vi "PDC.vi"() -> ()   [LabVIEW 2013]
uses:
  CTRLs/PMU_CMDs.ctl
panel:
  out "path":path
  out "T button?":bool
  out "PMU1 CFG Packet 2":string[](array[string])
  out "PMU Row Number":i32
  out "UDP STRNG 2":string
  out "Date/Time 4":string
  out "Phasor Row Number":i32
  in  "Tab Control 2":T1(tab)
  out "MagnitudePMU":waveform(sgl)(graph)
  out "FrequencyPMU":waveform(sgl)(graph)
  out "PMUROCOF":waveform(sgl)(graph)
  out "PMUAnalogs":waveform(sgl)(graph)
  out "seconds":dbl
  out "Array 2":u16[][](array[numeric]) format="%b"
  out "Array":string[][](array[string])
  out "Analogs":string[][](array[string])
  out "Freq Floating?":bool[](array[boolean])
  out "Analog Floating?":bool[](array[boolean])
  out "Polar?":bool[](array[boolean])
  out "Transposed":string[][](array[string])
  out "Real":string[][](array[string])
  out "Imaginary":string[][](array[string])
  out "transposed array 5":sgl[][](array[numeric])
  out "transposed array 4":sgl[][](array[numeric])
  out "Phasors Floatingpoint?":bool[](array[boolean])
  out "Format":u16[](array[numeric]) format="%b"
  out "Digitals":u16[](array[numeric])
  out "Analog":u16[](array[numeric])
  out "Phasor":u16[](array[numeric])
  out "DGTL Packet":string[](array[string])
  out "ANG Packet":string[](array[string])
  out "DFREQ Packet":string[](array[string])
  out "FREQ Packet":string[](array[string])
  out "PZRs Packet":string[](array[string])
  out "UNITs 2":T2
  out "Date/Time 3":string
  out "PMU DATA Packet 2":string[](array[string])
  out "DATA FRAME 2":string
  out "error out 2":errorcluster
  out "UDP STRNG":string
  out "UNITs":T2
  out "Date/Time 2":string
  in  "Start Com Button":bool
  in  "User Configuration":T3(tab)
  in  "IP Address":string="127.0.0.1"
  in  "remote port":u16=4712
  in  "Device ID":u16
  in  "Unicast Address":string="192.168.0.101"
  in  "Local Port":u16=58431
  in  "TTL":u16=16
  in  "Send to Port":u16=58432
  out "Alert Incorrect \nNetwork Info":bool
  in  "Data Display":T4(tab)
  in  "PMU Phasors":i32(listbox)
  in  "PMU Analogs":i32(listbox)
  in  "PMU Digitals":i32(listbox)
  in  "dFreq":sgl[](array[numeric])
  in  "Frequency":sgl[](array[numeric])
  in  "Tab Control":T5(tab)
  in  "Complex Phasors":csg[][](array[numeric])
  in  "Magnitude":sgl[][](array[numeric])
  in  "Angle":sgl[][](array[numeric])
  in  "Analog Values":sgl[][](array[numeric])
  out "Boolean array":bool[][](array[boolean])
  out "Magnitude":sgl[](array[numeric])
  out "Angle":sgl[](array[numeric])
  out "Complex Phasors":csg[](array[numeric])
  out "DFREQ Values":dbl[](array[numeric])
  out "FREQ Values":dbl[](array[numeric])
  out "Chosen Data 2":i32(listbox)
  out "DATA ONLINE":bool
  in  "Display Cluster Output":bool
  out "UDP String":string
  in  "Data Selector":T6(tab)
  out "No. of Digitals in this PMU":u8
  out "No. of Analogs in this PMU":u8
  out "No. of Phasors in this PMU":u8
  out "Freq/dFreq Format":string
  out "Analog Format":string
  out "Phasor Format":string
  out "Phasor Type":string
  out "DATA_RATE":u32
  in  "Names of PMUs":i32(listbox)
  out "Nominal_Frequency":string
  out "NUM_of_PMUs":u32
  in  "PMU Phasors List 2":i32(listbox)
  out "Phasor_Names":string[](array[string])
  in  "PMU Phasors List":i32(listbox)
  out "Phasors Index":u16[](array[numeric])
  out "PMU number in List":i32[](array[numeric])
  out "Phasor number in selected PMU":i32[](array[numeric])
  out "PMU DATA Packet":string[](array[string])
  out "Data size to read":u32
  out "Size of DATA Frame":u32
  out "CFG-2 Frame":string
  out "PMU1 CFG Packet":string[](array[string])
  out "Date/Time":string
  out "TIME_BASE":u32
  out "FRACSEC":u64
  out "SOC":u64
  out "IDCODE":u32
  out "FRAMSIZE":u32
  out "SYNC":u32
  out "Valid?!":bool
  out "CRC-Bytes":string
  out "DATA FRAME":string
  in  "Stop Button":bool
  out "COMMAND Frame":string
  out "bytes written":i32
  in  "DATA ON":bool
  in  "DATA OFF":bool
  out "length":i32
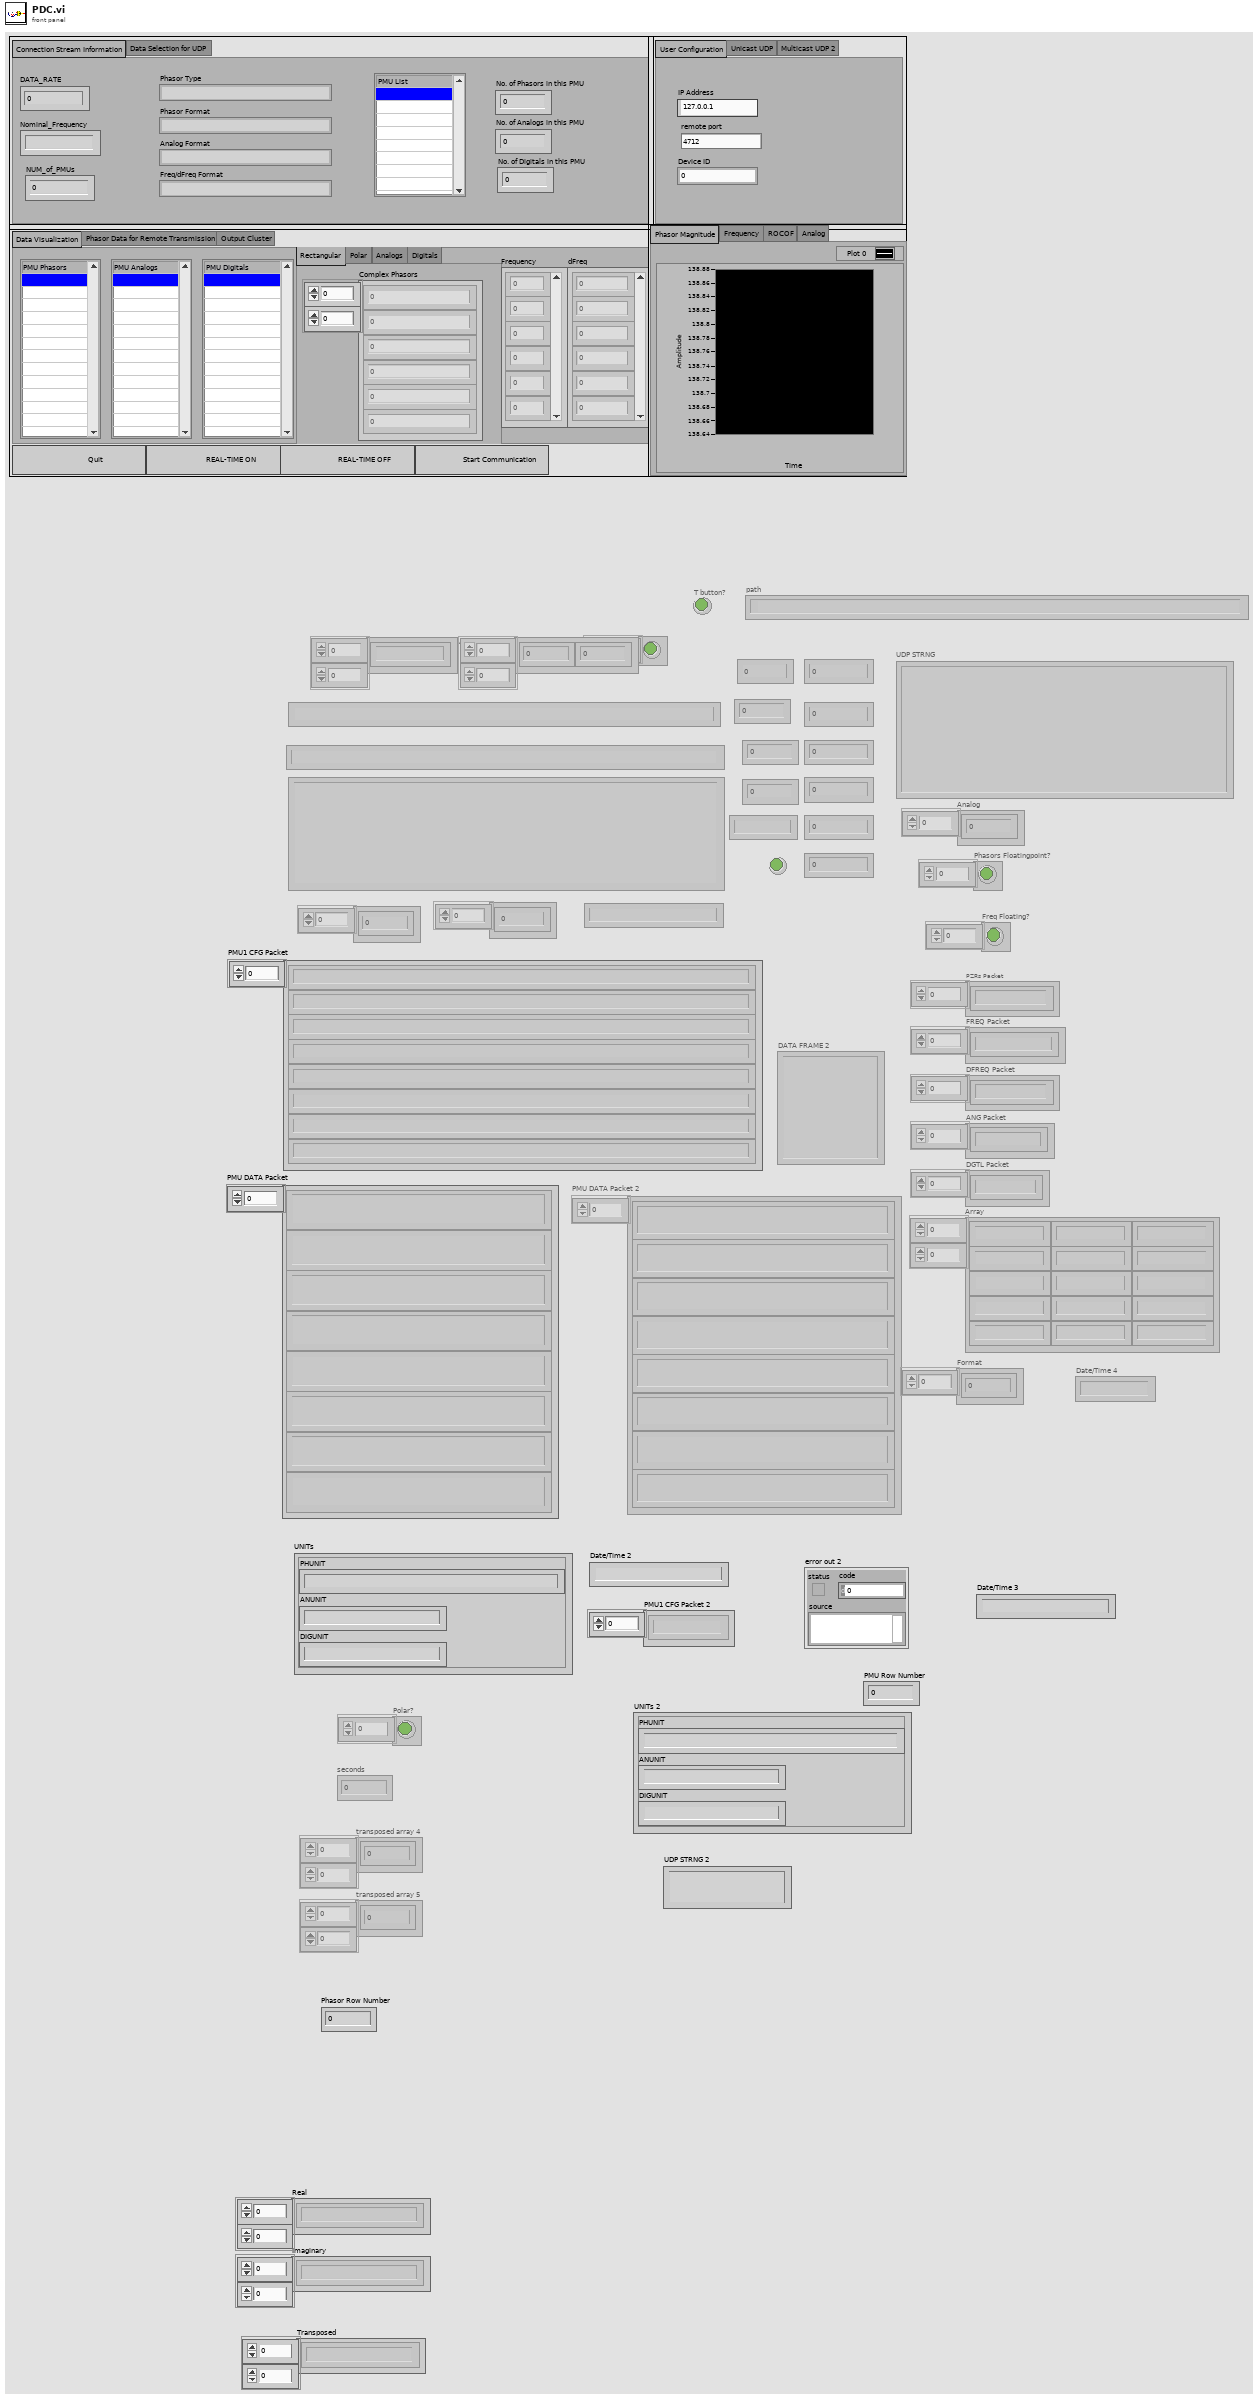
[diagram p1: front panel]
types:
  T1 = enum32{"Phasor Magnitude", "Frequency", "ROCOF", "Analog"}
  T2 = cluster{"PHUNIT":string, "ANUNIT":string, "DIGUNIT":string}
  T3 = enum32{"User Configuration", "Unicast UDP", "Multicast UDP 2"}
  T4 = enum32{"Data Visualization", "Phasor Data for Remote Transmission", "Output Cluster"}
  T5 = enum32{"Rectangular", "Polar", "Analogs", "Digitals"}
  T6 = enum32{"Connection Stream Information", "Data Selection for UDP"}
  T7 = cluster{"Date/Time":string, "DATA_DTLD":cluster{"PZRs Packet":string[], "FREQ Packet":string[], "DFREQ Packet":string[], "ANG Packet":string[], "DGTL Packet":string[]}}
  T8 = typedef "PMU_CMDs.ctl" = enum16{"dummy", "Turn off Transmission of Data Frame", "Turn on Transmission of Data Frame", "Send Header Frame", "Send CFG-1 Frame", "Send CFG-2 Frame", "Extended Frame"}
  T9 = cluster{"SYNC":u32, "FRAMSIZE":u32, "IDCODE":u32, "SOC":u64, "DATA_RATE":u32, "FRACSEC":u64, "TIME_BASE":u32, "NUM_PMU":u32}
  T10 = cluster{"PHASORS":cluster{"PZR 1":string, "PZR 2":string, "PZR 3":string, "PZR 4":string, "PZR 5":string, "PZR 6":string}, "NUMs":cluster{"PHNMR":u8, "ANNMR":u8, "DGNMR":u8}, "FORMAT":cluster{"PH_MAG_ANG":u16, "PH_FLOATING":u16, "AN_FLOATING":u16, "FREQ_DFREQ_FLOATING":u16}, "ANGs":cluster{"AN1":string, "AN2":string, "AN3":string}, "DIGs":cluster{"DIG 1":string, "DIG 2":string, "DIG 3":string, "DIG 4":string, "DIG 5":string, "DIG 6":string, "DIG 7":string, "DIG 8":string, "DIG 9":string, "DIG 10":string, "DIG 11":string, "DIG 12":string, "DIG 13":string, "DIG 14":string, "DIG 15":string, "DIG 16":string}, "IDCODE":u16, "Station Name":string, "UNITs":cluster{"PHUNIT":string, "ANUNIT":string, "DIGUNIT":string}, "FNOM":string, "CFGCNT":string}
  T11 = cluster{"PZRs Packet":string[], "FREQ Packet":string[], "DFREQ Packet":string[], "ANG Packet":string[], "DGTL Packet":string[]}
  T12 = typedef "LVDateTimeRec.ctl" = cluster{"fractional second":dbl, "second":i32, "minute":i32, "hour":i32, "day of month":i32, "month":i32, "year":i32, "day of week":i32, "day of year":i32, "DST":i32}
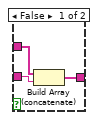
[diagram p4: hidden frame]
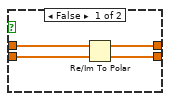
[diagram p5: hidden frame]
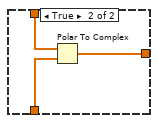
[diagram p6: hidden frame]
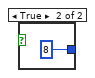
[diagram p7: hidden frame]
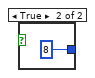
[diagram p8: hidden frame]
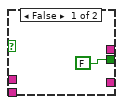
[diagram p11: hidden frame]
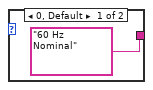
[diagram p14: hidden frame]
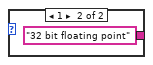
[diagram p15: hidden frame]
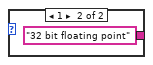
[diagram p16: hidden frame]
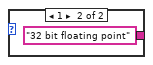
[diagram p17: hidden frame]
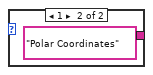
[diagram p18: hidden frame]
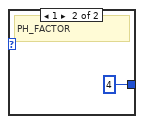
[diagram p19: hidden frame]
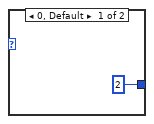
[diagram p20: hidden frame]
diagram:
  # "This file is part of BFE.\n\n    BFE is free software: you can redistribute it and/or modify\n    it under the terms of the GNU General Public License as published by\n    the Free Software Foundation, either version 3 of the License, or\n    (at your option) any later version.\n\n   BFE is distributed in the hope that it will be useful,\n    but WITHOUT ANY WARRANTY; without even the implied warranty of\n    MERCHANTABILITY or FITNESS FOR A PARTICULAR PURPOSE.  See the\n    GNU General Public License for more details.\n\n    You should have received a copy of the GNU General Public License\n    along with BFE.  If not, see <http://www.gnu.org/licenses/>."
  n1 = flat-sequence {
    tunnel: [w84] -> w64
    tunnel: [w83] -> w62
    frame #0 {
      w74 = "" ("Phasor Type")
      w73 = u8 0 ("No. of Phasors in this PMU")
      w72 = string[] [""] ("Phasor Name")
      # "License Prompt"
      # "Initializing all variables to their default values"
      n2 = Two Button Dialog(message="<BFE>  Copyright (C) <2016>  <Luigi Vanfretti, Muhammad Shoaib Almas, Maxime Baudette>\n    This program comes with ABSOLUTELY NO WARRANTY; for details click on \"show details\"'.\n    This is free software, and you are welcome to redistribute it\n    under certain conditions; click on `show details' for details.", 1:"Show Details" ("F button name (\"Cancel\")"), 2:"OK" ("T button name (\"OK\")")) -> (T button?=w67:bool)
      "T button?" <- w67
      n3 = Equal?(x=w67, y=FALSE) -> (x = y?=w65:bool)
      n4 = case shown="True" w65 {
        frame False {
        }
        frame True {
          n5 = Current VI's Path() -> (path=w79:path)
          "path" <- w79
          n6 = Strip Path(path=w79) -> (stripped path=w77:path)  [unwired: 1 out]
          n7 = Build Path(base path=w77, name or relative path="License") -> (appended path=w75:path)
          n8 = call <vilib>:"System Exec.vi"("working directory"=w75, "command line"="Notepad COPYING") -> ()  [unwired: 6 in, 4 out]
        }
      }
      n9 = property on="NUM_of_PMUs" class="DigNum (strict)"("Value"=w73) -> ()  [unwired: 2 in, 2 out]
      n10 = property on="DATA_RATE" class="DigNum (strict)"("Value"=w73) -> ()  [unwired: 2 in, 2 out]
      n11 = property on="No. of Phasors in this PMU" class="DigNum (strict)"("Value"=w73) -> ()  [unwired: 2 in, 2 out]
      n12 = property on="No. of Analogs in this PMU" class="DigNum (strict)"("Value"=w73) -> ()  [unwired: 2 in, 2 out]
      n13 = property on="No. of Digitals in this PMU" class="DigNum (strict)"("Value"=w73) -> ()  [unwired: 2 in, 2 out]
      n14 = property on="Analog Format" class="Str"("Value"=w74) -> ()  [unwired: 2 in, 2 out]
      n15 = property on="Phasor Type" class="Str"("Value"=w74) -> ()  [unwired: 2 in, 2 out]
      n16 = property on="Phasor Format" class="Str"("Value"=w74) -> ()  [unwired: 2 in, 2 out]
      n17 = property on="Freq/dFreq Format" class="Str"("Value"=w74) -> ()  [unwired: 2 in, 2 out]
      n18 = property on="Phasors Index" class="Arr (strict)"("Value"=u16[] [0, 0, 0, 0] ("Phasors Index")) -> ()  [unwired: 2 in, 2 out]
      n19 = property on="Nominal_Frequency" class="Str"("Value"=w74) -> ()  [unwired: 2 in, 2 out]
      n20 = property on="PMU Phasors List" class="LstBox (strict)"("Item Names"=w72) -> ()  [unwired: 2 in, 2 out]
      n21 = property on="PMU Analogs" class="LstBox (strict)"("Item Names"=w72) -> ()  [unwired: 2 in, 2 out]
      n22 = property on="PMU Phasors" class="LstBox (strict)"("Item Names"=w72) -> ()  [unwired: 2 in, 2 out]
      n23 = property on="PMU Digitals" class="LstBox (strict)"("Item Names"=w72) -> ()  [unwired: 2 in, 2 out]
      n24 = property on="Names of PMUs" class="LstBox (strict)"("Item Names"=w72) -> ()  [unwired: 2 in, 2 out]
      n25 = property on="Names of PMUs" class="LstBox (strict)"("Item Names"=w72) -> ()  [unwired: 2 in, 2 out]
      n26 = property on="Phasor_Names" class="Arr (strict)"("Value"=w72) -> ()  [unwired: 2 in, 2 out]
    }
    frame #1 {
      n27 = while {
        stop <- "Start Com Button" stop-if-true
      }
    }
    frame #2 {
      n28 = TCP Open Connection(address="IP Address", remote port or service name="remote port") -> (connection ID=w84:refnum<k5>, error out=w83:errorcluster)  [unwired: 3 in]
    }
  }
  n29 = flat-sequence {
    tunnel: w64 -> [w90]
    tunnel: w62 -> [w91]
    tunnel: [w89] -> w50
    tunnel: [w88] -> w49
    tunnel: ["Device ID"] -> w24
    tunnel: w50 -> [w95]
    tunnel: [w98] -> w48
    tunnel: w49 -> [w96]
    tunnel: [w97] -> w46
    tunnel: w24 -> [w92]
    tunnel: [w92] -> w23
    tunnel: w48 -> [w107]
    tunnel: [w108] -> w47
    tunnel: w46 -> [w106]
    tunnel: [w109] -> w45
    tunnel: [w100] -> w44
    tunnel: w23 -> [w99]
    tunnel: [w99] -> w22
    tunnel: w47 -> [w114]
    tunnel: [w114] -> w52
    tunnel: w45 -> [w113]
    tunnel: [w113] -> w51
    tunnel: w44 -> [w111]
    tunnel: [w111] -> w43
    tunnel: w22 -> [w110]
    tunnel: [w110] -> w21
    tunnel: w52 -> [w120]
    tunnel: [w119] -> w41
    tunnel: w51 -> [w118]
    tunnel: [w117] -> w40
    tunnel: w43 -> [w122]
    tunnel: [w122] -> w39
    tunnel: w21 -> [w115]
    tunnel: [w115] -> w20
    tunnel: w41 -> [w127]
    tunnel: w40 -> [w126]
    tunnel: [w129] -> w60
    tunnel: [w128] -> w59
    tunnel: w39 -> [w124]
    tunnel: [w124] -> w42
    tunnel: w20 -> [w123]
    tunnel: w60 -> [w141]
    tunnel: w59 -> [w140]
    tunnel: [w143] -> w58
    tunnel: [w142] -> w57
    tunnel: [w131] -> w56
    tunnel: w42 -> [w139]
    tunnel: w58 -> [w158]
    tunnel: w57 -> [w157]
    tunnel: w56 -> [w149]
    tunnel: [w158] -> w55
    tunnel: [w157] -> w54
    tunnel: [w149] -> w53
    tunnel: [w144] -> w38
    tunnel: w55 -> [w197]
    tunnel: w54 -> [w196]
    tunnel: w53 -> [w195]
    tunnel: w38 -> [w176]
    tunnel: [w197] -> w33
    tunnel: [w196] -> w32
    tunnel: [w172] -> w31
    tunnel: w33 -> [w218]
    tunnel: w32 -> [w217]
    tunnel: w31 -> [w216]
    tunnel: [w218] -> w28
    tunnel: [w217] -> w27
    tunnel: [w216] -> w26
    tunnel: [w230] -> w30
    tunnel: [w227] -> w61
    tunnel: [w225] -> w63
    tunnel: w28 -> [w226]
    tunnel: w27 -> [w228]
    tunnel: w26 -> [w230]
    frame #0 {
      n30 = call "CMD.vi"("PMU ID"="Device ID", "command"=PMU_CMDs."Turn off Transmission of Data Frame") -> ("CMD"=w87:string)  [unwired: 4 in, 1 out]
      n31 = TCP Write(connection ID=w90, data in=w87, error in (no error)=w91) -> (connection ID out=w89:refnum<k5>, error out=w88:errorcluster)  [unwired: 1 in, 1 out]
    }
    frame #1 {
      n32 = call "CMD.vi"("PMU ID"=w92, "command"=PMU_CMDs."Send CFG-2 Frame") -> ("CMD"=w93:string)  [unwired: 4 in, 1 out]
      n33 = TCP Write(connection ID=w95, data in=w93, error in (no error)=w96) -> (connection ID out=w98:refnum<k5>, error out=w97:errorcluster)  [unwired: 1 in, 1 out]
    }
    frame #2 {
      w103 = 2 ("offset (0)")
      n34 = TCP Read(connection ID=w107, bytes to read=4, error in (no error)=w106) -> (connection ID out=w108:refnum<k5>, data out=w104:string, error out=w109:errorcluster)  [unwired: 2 in]
      n35 = String Subset(string=w104, offset (0)=w103, length (rest)=w103) -> (substring=w102:string)
      n36 = Type Cast(type=u16 0 ("bytes to read"), x=w102) -> (*(type *) &x=w100:u16)
    }
    frame #3 {
      n37 = Wait (ms)(milliseconds to wait=u32 20) -> ()  [unwired: 1 out]
    }
    frame #4 {
      n38 = call "CMD.vi"("PMU ID"=w115, "command"=PMU_CMDs."Turn off Transmission of Data Frame") -> ("CMD"=w121:string)  [unwired: 4 in, 1 out]
      n39 = TCP Write(connection ID=w120, data in=w121, error in (no error)=w118) -> (connection ID out=w119:refnum<k5>, error out=w117:errorcluster)  [unwired: 1 in, 1 out]
    }
    frame #5 {
      n40 = call "CMD.vi"("PMU ID"=w123, "command"=PMU_CMDs."Send CFG-2 Frame") -> ("CMD"=w125:string)  [unwired: 4 in, 1 out]
      n41 = TCP Write(connection ID=w127, data in=w125, error in (no error)=w126) -> (connection ID out=w129:refnum<k5>, error out=w128:errorcluster)  [unwired: 1 in, 1 out]
    }
    frame #6 {
      w137 = 4 ("y")
      n42 = TCP Read(connection ID=w141, bytes to read=w139, error in (no error)=w140) -> (connection ID out=w143:refnum<k5>, data out=w132:string, error out=w142:errorcluster)  [unwired: 2 in]
      n43 = String Length(string=w132) -> (length=w138:i32)
      n44 = Subtract(x=w138, y=w137) -> (x-y=w133:i32)
      n45 = String Subset(string=w132, offset (0)=w133, length (rest)=w137) -> (substring=w136:string)
      n46 = String Subset(string=w132, offset (0)=0, length (rest)=w133) -> (substring=w135:string)
      n47 = Concatenate Strings(w136, w135) -> (w131:string)
      "CFG-2 Frame" <- w131
    }
    frame #7 {
      n48 = call "CHK_CRC.vi"("data in"=w149) -> ("Valid?!"=→"Valid?!":bool, "CRC-Bytes"=→"CRC-Bytes":string)
      n49 = call "SYS_INFO.vi"("CFG-2"=w149) -> ("output cluster"=w150:T9)
      n50 = Unbundle By Name(w150) -> ("SYNC"=→"SYNC":u32, "FRAMSIZE"=→"FRAMSIZE":u32, "IDCODE"=→"IDCODE":u32, "SOC"=w148:u64, "FRACSEC"=w146:u64, "TIME_BASE"=w145:u32, "NUM_PMU"=w144:u32, "DATA_RATE"=→"DATA_RATE":u32)
      "SOC" <- w148
      "FRACSEC" <- w146
      "TIME_BASE" <- w145
      "NUM_of_PMUs" <- w144
      n51 = call "UNIX-DATE_TIME.vi"("TIME_BASE"=w145, "FRACSEC"=w146, "SOC"=w148) -> ("Date/Time"=→"Date/Time":string)  [unwired: 1 out]
    }
    frame #8 {
      w192 = 4
      w174 = 2
      n52 = call "PMU_CFG-2_PACK.vi"("String"=w195) -> ("PMU1 CFG Packet"=w172:string[])
      "PMU1 CFG Packet" <- w172
      n53 = Index Array(array=w172, index=0) -> (element=w194:string)
      n54 = call "PMU_INFO.vi"("data in"=w194) -> ("RET_DATA"=w162:T10)
      n55 = Unbundle By Name(w162) -> ("FNOM"=w161:string)
      n56 = Type Cast(type=u16 2 ("length (rest)"), x=w161) -> (*(type *) &x=w160:u16)
      n57 = Unbundle By Name(w162) -> ("FORMAT.PH_MAG_ANG"=w168:u16, "FORMAT.PH_FLOATING"=w167:u16, "FORMAT.AN_FLOATING"=w166:u16, "FORMAT.FREQ_DFREQ_FLOATING"=w165:u16)
      n58 = case shown="1" w160 {
        tunnel: ["60 Hz Nominal" "50 Hz"] -> w159
        frame 0, Default {
        }
        frame 1 {
        }
      }
      "Nominal_Frequency" <- w159
      n59 = case shown="0, Default" w168 {
        tunnel: ["Rectangular Coordinates" "Polar Coordinates"] -> w164
        frame 0, Default {
        }
        frame 1 {
        }
      }
      "Phasor Type" <- w164
      n60 = case shown="0, Default" w167 {
        tunnel: ["16 bit integer" "32 bit floating point"] -> w171
        frame 0, Default {
        }
        frame 1 {
        }
      }
      "Phasor Format" <- w171
      n61 = case shown="0, Default" w166 {
        tunnel: ["16 bit integer" "32 bit floating point"] -> w170
        frame 0, Default {
        }
        frame 1 {
        }
      }
      "Analog Format" <- w170
      n62 = case shown="0, Default" w165 {
        tunnel: ["16 bit integer" "32 bit floating point"] -> w169
        frame 0, Default {
        }
        frame 1 {
        }
      }
      "Freq/dFreq Format" <- w169
      n63 = Unbundle By Name(w162) -> ("FORMAT.PH_FLOATING"=w185:u16, "FORMAT.AN_FLOATING"=w184:u16, "FORMAT.FREQ_DFREQ_FLOATING"=w186:u16, "NUMs.PHNMR"=w190:u8, "NUMs.ANNMR"=w182:u8, "NUMs.DGNMR"=w179:u8)  [unwired: 1 out]
      n64 = case shown="0, Default" w185 {
        tunnel: [4 8] -> w191
        frame 0, Default {
        }
        frame 1 {
          # "PH_FACTOR"
        }
      }
      n65 = case shown="0, Default" w184 {
        tunnel: [2 4] -> w183
        frame 0, Default {
        }
        frame 1 {
          # "PH_FACTOR"
        }
      }
      n66 = Multiply(x=w179, y=2) -> (x*y=w180:i32)
      n67 = case shown="1" w186 {
        tunnel: [2 4] -> w187
        frame 0, Default {
        }
        frame 1 {
          # "PH_FACTOR"
        }
      }
      n68 = Multiply(x=w191, y=w190) -> (x*y=w188:i32)
      n69 = Multiply(x=w182, y=w183) -> (x*y=w181:i32)
      n70 = Compound Arithmetic op=ADD(2, w188, w187, w187, w181, w180) -> (w177:i32)
      n71 = Multiply(x=w177, y=w176) -> (x*y=w175:u32)
      n72 = Compound Arithmetic op=ADD(w174, w174, w174, w192, w192, w175, w174) -> (→"Size of DATA Frame":u32)
    }
    frame #9 {
      n73 = property on="NUM_of_PMUs" class="DigNum (strict)"() -> ("Value"=w215:u32)  [unwired: 2 in, 2 out]
      n74 = for {
        N: w215 -> [_]
        tunnel: w216 -> [w222] mode=indexing
        tunnel: [w219] -> w214 mode=indexing
        n75 = String Subset(string=w222, offset (0)=0, length (rest)=16 ("length (rest)")) -> (substring=w219:string)
      }
      n76 = property on="PMU Phasors List 2" class="LstBox (strict)"("Item Names"=w214) -> ()  [unwired: 2 in, 2 out]
      n77 = property on="Names of PMUs" class="LstBox (strict)"("Item Names"=w214) -> ()  [unwired: 2 in, 2 out]
    }
    frame #10 {
      n78 = local read "Device ID"() -> (w223:u16)
      n79 = call "CMD.vi"("PMU ID"=w223, "command"=PMU_CMDs."Turn off Transmission of Data Frame") -> ("CMD"=w229:string)  [unwired: 4 in, 1 out]
      n80 = TCP Write(connection ID=w226, data in=w229, error in (no error)=w228) -> (connection ID out=w225:refnum<k5>, error out=w227:errorcluster)  [unwired: 1 in, 1 out]
    }
  }
  n81 = flat-sequence {
    tunnel: ["Send to Port"] -> w10
    tunnel: [w249] -> w7
    tunnel: [w248] -> w9
    tunnel: [w236] -> w8
    frame #0 {
      # "Local Port number on this\nmachine"
      # "Time To Live edit\nbox usually 16 is the\nbest to send over networks"
      # "IP Address of destination\nsite over UDP."
      # "send the phasor\nparameters to this\nUDP port edit box"
      # "Open a UDP port for Multicast Write Only."
      n82 = String To IP(1:"0.0.0.0" ("x")) -> (0:w245:u32)
      n83 = String To IP(1:"223.255.255.255" ("x")) -> (0:w244:u32)
      n84 = String To IP(1:"Unicast Address") -> (0:w236:u32)
      n85 = String To IP(1:"240.255.255.255" ("x")) -> (0:w240:u32)
      n86 = String To IP(1:"247.255.255.255" ("x")) -> (0:w239:u32)
      n87 = Greater Or Equal?(x=w236, y=w245) -> (x >= y?=w247:bool)
      n88 = Less Or Equal?(x=w236, y=w244) -> (x <= y?=w246:bool)
      n89 = Greater Or Equal?(x=w236, y=w240) -> (x >= y?=w235:bool)
      n90 = Less Or Equal?(x=w236, y=w239) -> (x <= y?=w234:bool)
      n91 = Not And(1:w246, 2:w247) -> (0:w233:bool)
      n92 = Not And(1:w234, 2:w235) -> (0:w232:bool)
      n93 = And(x=w233, y=w232) -> (x .and. y?=w231:bool)
      "Alert Incorrect \nNetwork Info" <- w231
      n94 = case shown="True" w231 {
        frame False {
        }
        frame True {
          n95 = call "Display Message to User"() -> ()  [unwired: 10 in, 2 out]
        }
      }
      n96 = UDP Open(9:"TTL", 11:"Local Port") -> (port=w249:refnum<k16>, 0:w248:errorcluster)  [unwired: 3 in, 1 out]
      "error out 2" <- w248
    }
  }
  n97 = Obtain Queue(name (unnamed)="DISP DATA", element data type=T7 {"Date/Time"="26-12-2013, 0:30:36 0.866666", "DATA_DTLD"={"PZRs Packet"=[], "FREQ Packet"=[], "DFREQ Packet"=[], "ANG Packet"=[], "DGTL Packet"=[]}}) -> (queue out=w4:refnum<queue>, error out=w3:errorcluster)  [unwired: 3 in, 1 out]
  n98 = Obtain Queue(name (unnamed)="DATA FRAME", element data type=cluster{"DATA Type":string, "CFG Type":string[]} {"DATA Type"="", "CFG Type"=["PMU.001\u0000\u0000\u0000\u0000\u0000\u0000\u0000\u0000\u0000\u0000\u0001\u0000\u000f\u0000\u0006\u0000\u0003\u0000\u0001PZR.AI          PZR.BV          PZR.CI          PZR.AV          PZR.BI          PZR.CV          ANA1            ANA2            ANA3            DIG.stat1_01    DIG.stat1_02    DIG.stat1_03    DIG.stat1_04    DIG.stat1_05    DIG.stat1_06    DIG.stat1_07    DIG.stat1_08    DIG.stat1_09    DIG.stat1_10    DIG.stat1_11    DIG.stat1_12    DIG.stat1_13    DIG.stat1_14    DIG.stat1_15    DIG.stat1_16    \u0001\u0000\u0000\u0000\u0000\u0000\u0000\u0000\u0001\u0000\u0000\u0000\u0000\u0000\u0000\u0000\u0001\u0000\u0000\u0000\u0000\u0000\u0000\u0000\u0000\u0000\u0000\u0000\u0000\u0000\u0000\u0000\u0000\u0000\u0000\u0000ÿÿ\u0000\u0000\u0000\u0000\u0000\u0000", "PMU.002\u0000\u0000\u0000\u0000\u0000\u0000\u0000\u0000\u0000\u0000\u0002\u0000\u000f\u0000\u0006\u0000\u0003\u0000\u0001PZR.AI          PZR.BV          PZR.CI          PZR.AV          PZR.BI          PZR.CV          ANA1            ANA2            ANA3            DIG.stat1_01    DIG.stat1_02    DIG.stat1_03    DIG.stat1_04    DIG.stat1_05    DIG.stat1_06    DIG.stat1_07    DIG.stat1_08    DIG.stat1_09    DIG.stat1_10    DIG.stat1_11    DIG.stat1_12    DIG.stat1_13    DIG.stat1_14    DIG.stat1_15    DIG.stat1_16    \u0001\u0000\u0000\u0000\u0000\u0000\u0000\u0000\u0001\u0000\u0000\u0000\u0000\u0000\u0000\u0000\u0001\u0000\u0000\u0000\u0000\u0000\u0000\u0000\u0000\u0000\u0000\u0000\u0000\u0000\u0000\u0000\u0000\u0000\u0000\u0000ÿÿ\u0000\u0000\u0000\u0000\u0000\u0000", "PMU.003\u0000\u0000\u0000\u0000\u0000\u0000\u0000\u0000\u0000\u0000\u0003\u0000\u000f\u0000\u0006\u0000\u0003\u0000\u0001PZR.AI          PZR.BV          PZR.CI          PZR.AV          PZR.BI          PZR.CV          ANA1            ANA2            ANA3            DIG.stat1_01    DIG.stat1_02    DIG.stat1_03    DIG.stat1_04    DIG.stat1_05    DIG.stat1_06    DIG.stat1_07    DIG.stat1_08    DIG.stat1_09    DIG.stat1_10    DIG.stat1_11    DIG.stat1_12    DIG.stat1_13    DIG.stat1_14    DIG.stat1_15    DIG.stat1_16    \u0001\u0000\u0000\u0000\u0000\u0000\u0000\u0000\u0001\u0000\u0000\u0000\u0000\u0000\u0000\u0000\u0001\u0000\u0000\u0000\u0000\u0000\u0000\u0000\u0000\u0000\u0000\u0000\u0000\u0000\u0000\u0000\u0000\u0000\u0000\u0000ÿÿ\u0000\u0000\u0000\u0000\u0000\u0000", "PMU.004\u0000\u0000\u0000\u0000\u0000\u0000\u0000\u0000\u0000\u0000\u0004\u0000\u000f\u0000\u0006\u0000\u0003\u0000\u0001PZR.AI          PZR.BV          PZR.CI          PZR.AV          PZR.BI          PZR.CV          ANA1            ANA2            ANA3            DIG.stat1_01    DIG.stat1_02    DIG.stat1_03    DIG.stat1_04    DIG.stat1_05    DIG.stat1_06    DIG.stat1_07    DIG.stat1_08    DIG.stat1_09    DIG.stat1_10    DIG.stat1_11    DIG.stat1_12    DIG.stat1_13    DIG.stat1_14    DIG.stat1_15    DIG.stat1_16    \u0001\u0000\u0000\u0000\u0000\u0000\u0000\u0000\u0001\u0000\u0000\u0000\u0000\u0000\u0000\u0000\u0001\u0000\u0000\u0000\u0000\u0000\u0000\u0000\u0000\u0000\u0000\u0000\u0000\u0000\u0000\u0000\u0000\u0000\u0000\u0000ÿÿ\u0000\u0000\u0000\u0000\u0000\u0000", "PMU.005\u0000\u0000\u0000\u0000\u0000\u0000\u0000\u0000\u0000\u0000\u0005\u0000\u000f\u0000\u0006\u0000\u0003\u0000\u0001PZR.AI          PZR.BV          PZR.CI          PZR.AV          PZR.BI          PZR.CV          ANA1            ANA2            ANA3            DIG.stat1_01    DIG.stat1_02    DIG.stat1_03    DIG.stat1_04    DIG.stat1_05    DIG.stat1_06    DIG.stat1_07    DIG.stat1_08    DIG.stat1_09    DIG.stat1_10    DIG.stat1_11    DIG.stat1_12    DIG.stat1_13    DIG.stat1_14    DIG.stat1_15    DIG.stat1_16    \u0001\u0000\u0000\u0000\u0000\u0000\u0000\u0000\u0001\u0000\u0000\u0000\u0000\u0000\u0000\u0000\u0001\u0000\u0000\u0000\u0000\u0000\u0000\u0000\u0000\u0000\u0000\u0000\u0000\u0000\u0000\u0000\u0000\u0000\u0000\u0000ÿÿ\u0000\u0000\u0000\u0000\u0000\u0000", "PMU.006\u0000\u0000\u0000\u0000\u0000\u0000\u0000\u0000\u0000\u0000\u0006\u0000\u000f\u0000\u0006\u0000\u0003\u0000\u0001PZR.AI          PZR.BV          PZR.CI          PZR.AV          PZR.BI          PZR.CV          ANA1            ANA2            ANA3            DIG.stat1_01    DIG.stat1_02    DIG.stat1_03    DIG.stat1_04    DIG.stat1_05    DIG.stat1_06    DIG.stat1_07    DIG.stat1_08    DIG.stat1_09    DIG.stat1_10    DIG.stat1_11    DIG.stat1_12    DIG.stat1_13    DIG.stat1_14    DIG.stat1_15    DIG.stat1_16    \u0001\u0000\u0000\u0000\u0000\u0000\u0000\u0000\u0001\u0000\u0000\u0000\u0000\u0000\u0000\u0000\u0001\u0000\u0000\u0000\u0000\u0000\u0000\u0000\u0000\u0000\u0000\u0000\u0000\u0000\u0000\u0000\u0000\u0000\u0000\u0000ÿÿ\u0000\u0000\u0000\u0000\u0000\u0000", "PMU.007\u0000\u0000\u0000\u0000\u0000\u0000\u0000\u0000\u0000\u0000\u0007\u0000\u000f\u0000\u0006\u0000\u0003\u0000\u0001PZR.AI          PZR.BV          PZR.CI          PZR.AV          PZR.BI          PZR.CV          ANA1            ANA2            ANA3            DIG.stat1_01    DIG.stat1_02    DIG.stat1_03    DIG.stat1_04    DIG.stat1_05    DIG.stat1_06    DIG.stat1_07    DIG.stat1_08    DIG.stat1_09    DIG.stat1_10    DIG.stat1_11    DIG.stat1_12    DIG.stat1_13    DIG.stat1_14    DIG.stat1_15    DIG.stat1_16    \u0001\u0000\u0000\u0000\u0000\u0000\u0000\u0000\u0001\u0000\u0000\u0000\u0000\u0000\u0000\u0000\u0001\u0000\u0000\u0000\u0000\u0000\u0000\u0000\u0000\u0000\u0000\u0000\u0000\u0000\u0000\u0000\u0000\u0000\u0000\u0000ÿÿ\u0000\u0000\u0000\u0000\u0000\u0000", "PMU.008\u0000\u0000\u0000\u0000\u0000\u0000\u0000\u0000\u0000\u0000\b\u0000\u000f\u0000\u0006\u0000\u0003\u0000\u0001PZR.AI          PZR.BV          PZR.CI          PZR.AV          PZR.BI          PZR.CV          ANA1            ANA2            ANA3            DIG.stat1_01    DIG.stat1_02    DIG.stat1_03    DIG.stat1_04    DIG.stat1_05    DIG.stat1_06    DIG.stat1_07    DIG.stat1_08    DIG.stat1_09    DIG.stat1_10    DIG.stat1_11    DIG.stat1_12    DIG.stat1_13    DIG.stat1_14    DIG.stat1_15    DIG.stat1_16    \u0001\u0000\u0000\u0000\u0000\u0000\u0000\u0000\u0001\u0000\u0000\u0000\u0000\u0000\u0000\u0000\u0001\u0000\u0000\u0000\u0000\u0000\u0000\u0000\u0000\u0000\u0000\u0000\u0000\u0000\u0000\u0000\u0000\u0000\u0000\u0000ÿÿ\u0000\u0000\u0000\u0000\u0000\u0000", "PMU.009\u0000\u0000\u0000\u0000\u0000\u0000\u0000\u0000\u0000\u0000\t\u0000\u000f\u0000\u0006\u0000\u0003\u0000\u0001PZR.AI          PZR.BV          PZR.CI          PZR.AV          PZR.BI          PZR.CV          ANA1            ANA2            ANA3            DIG.stat1_01    DIG.stat1_02    DIG.stat1_03    DIG.stat1_04    DIG.stat1_05    DIG.stat1_06    DIG.stat1_07    DIG.stat1_08    DIG.stat1_09    DIG.stat1_10    DIG.stat1_11    DIG.stat1_12    DIG.stat1_13    DIG.stat1_14    DIG.stat1_15    DIG.stat1_16    \u0001\u0000\u0000\u0000\u0000\u0000\u0000\u0000\u0001\u0000\u0000\u0000\u0000\u0000\u0000\u0000\u0001\u0000\u0000\u0000\u0000\u0000\u0000\u0000\u0000\u0000\u0000\u0000\u0000\u0000\u0000\u0000\u0000\u0000\u0000\u0000ÿÿ\u0000\u0000\u0000\u0000\u0000\u0000", "PMU.010\u0000\u0000\u0000\u0000\u0000\u0000\u0000\u0000\u0000\u0000\n\u0000\u000f\u0000\u0006\u0000\u0003\u0000\u0001PZR.AI          PZR.BV          PZR.CI          PZR.AV          PZR.BI          PZR.CV          ANA1            ANA2            ANA3            DIG.stat1_01    DIG.stat1_02    DIG.stat1_03    DIG.stat1_04    DIG.stat1_05    DIG.stat1_06    DIG.stat1_07    DIG.stat1_08    DIG.stat1_09    DIG.stat1_10    DIG.stat1_11    DIG.stat1_12    DIG.stat1_13    DIG.stat1_14    DIG.stat1_15    DIG.stat1_16    \u0001\u0000\u0000\u0000\u0000\u0000\u0000\u0000\u0001\u0000\u0000\u0000\u0000\u0000\u0000\u0000\u0001\u0000\u0000\u0000\u0000\u0000\u0000\u0000\u0000\u0000\u0000\u0000\u0000\u0000\u0000\u0000\u0000\u0000\u0000\u0000ÿÿ\u0000\u0000\u0000\u0000\u0000\u0000", "PMU.011\u0000\u0000\u0000\u0000\u0000\u0000\u0000\u0000\u0000\u0000\u000b\u0000\u000f\u0000\u0006\u0000\u0003\u0000\u0001PZR.AI          PZR.BV          PZR.CI          PZR.AV          PZR.BI          PZR.CV          ANA1            ANA2            ANA3            DIG.stat1_01    DIG.stat1_02    DIG.stat1_03    DIG.stat1_04    DIG.stat1_05    DIG.stat1_06    DIG.stat1_07    DIG.stat1_08    DIG.stat1_09    DIG.stat1_10    DIG.stat1_11    DIG.stat1_12    DIG.stat1_13    DIG.stat1_14    DIG.stat1_15    DIG.stat1_16    \u0001\u0000\u0000\u0000\u0000\u0000\u0000\u0000\u0001\u0000\u0000\u0000\u0000\u0000\u0000\u0000\u0001\u0000\u0000\u0000\u0000\u0000\u0000\u0000\u0000\u0000\u0000\u0000\u0000\u0000\u0000\u0000\u0000\u0000\u0000\u0000ÿÿ\u0000\u0000\u0000\u0000\u0000\u0000", "PMU.012\u0000\u0000\u0000\u0000\u0000\u0000\u0000\u0000\u0000\u0000\f\u0000\u000f\u0000\u0006\u0000\u0003\u0000\u0001PZR.AI          PZR.BV          PZR.CI          PZR.AV          PZR.BI          PZR.CV          ANA1            ANA2            ANA3            DIG.stat1_01    DIG.stat1_02    DIG.stat1_03    DIG.stat1_04    DIG.stat1_05    DIG.stat1_06    DIG.stat1_07    DIG.stat1_08    DIG.stat1_09    DIG.stat1_10    DIG.stat1_11    DIG.stat1_12    DIG.stat1_13    DIG.stat1_14    DIG.stat1_15    DIG.stat1_16    \u0001\u0000\u0000\u0000\u0000\u0000\u0000\u0000\u0001\u0000\u0000\u0000\u0000\u0000\u0000\u0000\u0001\u0000\u0000\u0000\u0000\u0000\u0000\u0000\u0000\u0000\u0000\u0000\u0000\u0000\u0000\u0000\u0000\u0000\u0000\u0000ÿÿ\u0000\u0000\u0000\u0000\u0000\u0000", "PMU.013\u0000\u0000\u0000\u0000\u0000\u0000\u0000\u0000\u0000\u0000\r\u0000\u000f\u0000\u0006\u0000\u0003\u0000\u0001PZR.AI          PZR.BV          PZR.CI          PZR.AV          PZR.BI          PZR.CV          ANA1            ANA2            ANA3            DIG.stat1_01    DIG.stat1_02    DIG.stat1_03    DIG.stat1_04    DIG.stat1_05    DIG.stat1_06    DIG.stat1_07    DIG.stat1_08    DIG.stat1_09    DIG.stat1_10    DIG.stat1_11    DIG.stat1_12    DIG.stat1_13    DIG.stat1_14    DIG.stat1_15    DIG.stat1_16    \u0001\u0000\u0000\u0000\u0000\u0000\u0000\u0000\u0001\u0000\u0000\u0000\u0000\u0000\u0000\u0000\u0001\u0000\u0000\u0000\u0000\u0000\u0000\u0000\u0000\u0000\u0000\u0000\u0000\u0000\u0000\u0000\u0000\u0000\u0000\u0000ÿÿ\u0000\u0000\u0000\u0000\u0000\u0000", "PMU.014\u0000\u0000\u0000\u0000\u0000\u0000\u0000\u0000\u0000\u0000\u000e\u0000\u000f\u0000\u0006\u0000\u0003\u0000\u0001PZR.AI          PZR.BV          PZR.CI          PZR.AV          PZR.BI          PZR.CV          ANA1            ANA2            ANA3            DIG.stat1_01    DIG.stat1_02    DIG.stat1_03    DIG.stat1_04    DIG.stat1_05    DIG.stat1_06    DIG.stat1_07    DIG.stat1_08    DIG.stat1_09    DIG.stat1_10    DIG.stat1_11    DIG.stat1_12    DIG.stat1_13    DIG.stat1_14    DIG.stat1_15    DIG.stat1_16    \u0001\u0000\u0000\u0000\u0000\u0000\u0000\u0000\u0001\u0000\u0000\u0000\u0000\u0000\u0000\u0000\u0001\u0000\u0000\u0000\u0000\u0000\u0000\u0000\u0000\u0000\u0000\u0000\u0000\u0000\u0000\u0000\u0000\u0000\u0000\u0000ÿÿ\u0000\u0000\u0000\u0000\u0000\u0000", "PMU.015\u0000\u0000\u0000\u0000\u0000\u0000\u0000\u0000\u0000\u0000\u000f\u0000\u000f\u0000\u0006\u0000\u0003\u0000\u0001PZR.AI          PZR.BV          PZR.CI          PZR.AV          PZR.BI          PZR.CV          ANA1            ANA2            ANA3            DIG.stat1_01    DIG.stat1_02    DIG.stat1_03    DIG.stat1_04    DIG.stat1_05    DIG.stat1_06    DIG.stat1_07    DIG.stat1_08    DIG.stat1_09    DIG.stat1_10    DIG.stat1_11    DIG.stat1_12    DIG.stat1_13    DIG.stat1_14    DIG.stat1_15    DIG.stat1_16    \u0001\u0000\u0000\u0000\u0000\u0000\u0000\u0000\u0001\u0000\u0000\u0000\u0000\u0000\u0000\u0000\u0001\u0000\u0000\u0000\u0000\u0000\u0000\u0000\u0000\u0000\u0000\u0000\u0000\u0000\u0000\u0000\u0000\u0000\u0000\u0000ÿÿ\u0000\u0000\u0000\u0000\u0000\u0000", "PMU.016\u0000\u0000\u0000\u0000\u0000\u0000\u0000\u0000\u0000\u0000\u0010\u0000\u000f\u0000\u0006\u0000\u0003\u0000\u0001PZR.AI          PZR.BV          PZR.CI          PZR.AV          PZR.BI          PZR.CV          ANA1            ANA2            ANA3            DIG.stat1_01    DIG.stat1_02    DIG.stat1_03    DIG.stat1_04    DIG.stat1_05    DIG.stat1_06    DIG.stat1_07    DIG.stat1_08    DIG.stat1_09    DIG.stat1_10    DIG.stat1_11    DIG.stat1_12    DIG.stat1_13    DIG.stat1_14    DIG.stat1_15    DIG.stat1_16    \u0001\u0000\u0000\u0000\u0000\u0000\u0000\u0000\u0001\u0000\u0000\u0000\u0000\u0000\u0000\u0000\u0001\u0000\u0000\u0000\u0000\u0000\u0000\u0000\u0000\u0000\u0000\u0000\u0000\u0000\u0000\u0000\u0000\u0000\u0000\u0000ÿÿ\u0000\u0000\u0000\u0000\u0000\u0000", "PMU.017\u0000\u0000\u0000\u0000\u0000\u0000\u0000\u0000\u0000\u0000\u0011\u0000\u000f\u0000\u0006\u0000\u0003\u0000\u0001PZR.AI          PZR.BV          PZR.CI          PZR.AV          PZR.BI          PZR.CV          ANA1            ANA2            ANA3            DIG.stat1_01    DIG.stat1_02    DIG.stat1_03    DIG.stat1_04    DIG.stat1_05    DIG.stat1_06    DIG.stat1_07    DIG.stat1_08    DIG.stat1_09    DIG.stat1_10    DIG.stat1_11    DIG.stat1_12    DIG.stat1_13    DIG.stat1_14    DIG.stat1_15    DIG.stat1_16    \u0001\u0000\u0000\u0000\u0000\u0000\u0000\u0000\u0001\u0000\u0000\u0000\u0000\u0000\u0000\u0000\u0001\u0000\u0000\u0000\u0000\u0000\u0000\u0000\u0000\u0000\u0000\u0000\u0000\u0000\u0000\u0000\u0000\u0000\u0000\u0000ÿÿ\u0000\u0000\u0000\u0000\u0000\u0000", "PMU.018\u0000\u0000\u0000\u0000\u0000\u0000\u0000\u0000\u0000\u0000\u0012\u0000\u000f\u0000\u0006\u0000\u0003\u0000\u0001PZR.AI          PZR.BV          PZR.CI          PZR.AV          PZR.BI          PZR.CV          ANA1            ANA2            ANA3            DIG.stat1_01    DIG.stat1_02    DIG.stat1_03    DIG.stat1_04    DIG.stat1_05    DIG.stat1_06    DIG.stat1_07    DIG.stat1_08    DIG.stat1_09    DIG.stat1_10    DIG.stat1_11    DIG.stat1_12    DIG.stat1_13    DIG.stat1_14    DIG.stat1_15    DIG.stat1_16    \u0001\u0000\u0000\u0000\u0000\u0000\u0000\u0000\u0001\u0000\u0000\u0000\u0000\u0000\u0000\u0000\u0001\u0000\u0000\u0000\u0000\u0000\u0000\u0000\u0000\u0000\u0000\u0000\u0000\u0000\u0000\u0000\u0000\u0000\u0000\u0000ÿÿ\u0000\u0000\u0000\u0000\u0000\u0000", "PMU.019\u0000\u0000\u0000\u0000\u0000\u0000\u0000\u0000\u0000\u0000\u0013\u0000\u000f\u0000\u0006\u0000\u0003\u0000\u0001PZR.AI          PZR.BV          PZR.CI          PZR.AV          PZR.BI          PZR.CV          ANA1            ANA2            ANA3            DIG.stat1_01    DIG.stat1_02    DIG.stat1_03    DIG.stat1_04    DIG.stat1_05    DIG.stat1_06    DIG.stat1_07    DIG.stat1_08    DIG.stat1_09    DIG.stat1_10    DIG.stat1_11    DIG.stat1_12    DIG.stat1_13    DIG.stat1_14    DIG.stat1_15    DIG.stat1_16    \u0001\u0000\u0000\u0000\u0000\u0000\u0000\u0000\u0001\u0000\u0000\u0000\u0000\u0000\u0000\u0000\u0001\u0000\u0000\u0000\u0000\u0000\u0000\u0000\u0000\u0000\u0000\u0000\u0000\u0000\u0000\u0000\u0000\u0000\u0000\u0000ÿÿ\u0000\u0000\u0000\u0000\u0000\u0000", "PMU.020\u0000\u0000\u0000\u0000\u0000\u0000\u0000\u0000\u0000\u0000\u0014\u0000\u000f\u0000\u0006\u0000\u0003\u0000\u0001PZR.AI          PZR.BV          PZR.CI          PZR.AV          PZR.BI          PZR.CV          ANA1            ANA2            ANA3            DIG.stat1_01    DIG.stat1_02    DIG.stat1_03    DIG.stat1_04    DIG.stat1_05    DIG.stat1_06    DIG.stat1_07    DIG.stat1_08    DIG.stat1_09    DIG.stat1_10    DIG.stat1_11    DIG.stat1_12    DIG.stat1_13    DIG.stat1_14    DIG.stat1_15    DIG.stat1_16    \u0001\u0000\u0000\u0000\u0000\u0000\u0000\u0000\u0001\u0000\u0000\u0000\u0000\u0000\u0000\u0000\u0001\u0000\u0000\u0000\u0000\u0000\u0000\u0000\u0000\u0000\u0000\u0000\u0000\u0000\u0000\u0000\u0000\u0000\u0000\u0000ÿÿ\u0000\u0000\u0000\u0000\u0000\u0000", "PMU.021\u0000\u0000\u0000\u0000\u0000\u0000\u0000\u0000\u0000\u0000\u0015\u0000\u000f\u0000\u0006\u0000\u0003\u0000\u0001PZR.AI          PZR.BV          PZR.CI          PZR.AV          PZR.BI          PZR.CV          ANA1            ANA2            ANA3            DIG.stat1_01    DIG.stat1_02    DIG.stat1_03    DIG.stat1_04    DIG.stat1_05    DIG.stat1_06    DIG.stat1_07    DIG.stat1_08    DIG.stat1_09    DIG.stat1_10    DIG.stat1_11    DIG.stat1_12    DIG.stat1_13    DIG.stat1_14    DIG.stat1_15    DIG.stat1_16    \u0001\u0000\u0000\u0000\u0000\u0000\u0000\u0000\u0001\u0000\u0000\u0000\u0000\u0000\u0000\u0000\u0001\u0000\u0000\u0000\u0000\u0000\u0000\u0000\u0000\u0000\u0000\u0000\u0000\u0000\u0000\u0000\u0000\u0000\u0000\u0000ÿÿ\u0000\u0000\u0000\u0000\u0000\u0000", "PMU.022\u0000\u0000\u0000\u0000\u0000\u0000\u0000\u0000\u0000\u0000\u0016\u0000\u000f\u0000\u0006\u0000\u0003\u0000\u0001PZR.AI          PZR.BV          PZR.CI          PZR.AV          PZR.BI          PZR.CV          ANA1            ANA2            ANA3            DIG.stat1_01    DIG.stat1_02    DIG.stat1_03    DIG.stat1_04    DIG.stat1_05    DIG.stat1_06    DIG.stat1_07    DIG.stat1_08    DIG.stat1_09    DIG.stat1_10    DIG.stat1_11    DIG.stat1_12    DIG.stat1_13    DIG.stat1_14    DIG.stat1_15    DIG.stat1_16    \u0001\u0000\u0000\u0000\u0000\u0000\u0000\u0000\u0001\u0000\u0000\u0000\u0000\u0000\u0000\u0000\u0001\u0000\u0000\u0000\u0000\u0000\u0000\u0000\u0000\u0000\u0000\u0000\u0000\u0000\u0000\u0000\u0000\u0000\u0000\u0000ÿÿ\u0000\u0000\u0000\u0000\u0000\u0000", "PMU.023\u0000\u0000\u0000\u0000\u0000\u0000\u0000\u0000\u0000\u0000\u0017\u0000\u000f\u0000\u0006\u0000\u0003\u0000\u0001PZR.AI          PZR.BV          PZR.CI          PZR.AV          PZR.BI          PZR.CV          ANA1            ANA2            ANA3            DIG.stat1_01    DIG.stat1_02    DIG.stat1_03    DIG.stat1_04    DIG.stat1_05    DIG.stat1_06    DIG.stat1_07    DIG.stat1_08    DIG.stat1_09    DIG.stat1_10    DIG.stat1_11    DIG.stat1_12    DIG.stat1_13    DIG.stat1_14    DIG.stat1_15    DIG.stat1_16    \u0001\u0000\u0000\u0000\u0000\u0000\u0000\u0000\u0001\u0000\u0000\u0000\u0000\u0000\u0000\u0000\u0001\u0000\u0000\u0000\u0000\u0000\u0000\u0000\u0000\u0000\u0000\u0000\u0000\u0000\u0000\u0000\u0000\u0000\u0000\u0000ÿÿ\u0000\u0000\u0000\u0000\u0000\u0000", "PMU.024\u0000\u0000\u0000\u0000\u0000\u0000\u0000\u0000\u0000\u0000\u0018\u0000\u000f\u0000\u0006\u0000\u0003\u0000\u0001PZR.AI          PZR.BV          PZR.CI          PZR.AV          PZR.BI          PZR.CV          ANA1            ANA2            ANA3            DIG.stat1_01    DIG.stat1_02    DIG.stat1_03    DIG.stat1_04    DIG.stat1_05    DIG.stat1_06    DIG.stat1_07    DIG.stat1_08    DIG.stat1_09    DIG.stat1_10    DIG.stat1_11    DIG.stat1_12    DIG.stat1_13    DIG.stat1_14    DIG.stat1_15    DIG.stat1_16    \u0001\u0000\u0000\u0000\u0000\u0000\u0000\u0000\u0001\u0000\u0000\u0000\u0000\u0000\u0000\u0000\u0001\u0000\u0000\u0000\u0000\u0000\u0000\u0000\u0000\u0000\u0000\u0000\u0000\u0000\u0000\u0000\u0000\u0000\u0000\u0000ÿÿ\u0000\u0000\u0000\u0000\u0000\u0000", "PMU.025\u0000\u0000\u0000\u0000\u0000\u0000\u0000\u0000\u0000\u0000\u0019\u0000\u000f\u0000\u0006\u0000\u0003\u0000\u0001PZR.AI          PZR.BV          PZR.CI          PZR.AV          PZR.BI          PZR.CV          ANA1            ANA2            ANA3            DIG.stat1_01    DIG.stat1_02    DIG.stat1_03    DIG.stat1_04    DIG.stat1_05    DIG.stat1_06    DIG.stat1_07    DIG.stat1_08    DIG.stat1_09    DIG.stat1_10    DIG.stat1_11    DIG.stat1_12    DIG.stat1_13    DIG.stat1_14    DIG.stat1_15    DIG.stat1_16    \u0001\u0000\u0000\u0000\u0000\u0000\u0000\u0000\u0001\u0000\u0000\u0000\u0000\u0000\u0000\u0000\u0001\u0000\u0000\u0000\u0000\u0000\u0000\u0000\u0000\u0000\u0000\u0000\u0000\u0000\u0000\u0000\u0000\u0000\u0000\u0000ÿÿ\u0000\u0000\u0000\u0000\u0000\u0000", "PMU.026\u0000\u0000\u0000\u0000\u0000\u0000\u0000\u0000\u0000\u0000\u001a\u0000\u000f\u0000\u0006\u0000\u0003\u0000\u0001PZR.AI          PZR.BV          PZR.CI          PZR.AV          PZR.BI          PZR.CV          ANA1            ANA2            ANA3            DIG.stat1_01    DIG.stat1_02    DIG.stat1_03    DIG.stat1_04    DIG.stat1_05    DIG.stat1_06    DIG.stat1_07    DIG.stat1_08    DIG.stat1_09    DIG.stat1_10    DIG.stat1_11    DIG.stat1_12    DIG.stat1_13    DIG.stat1_14    DIG.stat1_15    DIG.stat1_16    \u0001\u0000\u0000\u0000\u0000\u0000\u0000\u0000\u0001\u0000\u0000\u0000\u0000\u0000\u0000\u0000\u0001\u0000\u0000\u0000\u0000\u0000\u0000\u0000\u0000\u0000\u0000\u0000\u0000\u0000\u0000\u0000\u0000\u0000\u0000\u0000ÿÿ\u0000\u0000\u0000\u0000\u0000\u0000", "PMU.027\u0000\u0000\u0000\u0000\u0000\u0000\u0000\u0000\u0000\u0000\u001b\u0000\u000f\u0000\u0006\u0000\u0003\u0000\u0001PZR.AI          PZR.BV          PZR.CI          PZR.AV          PZR.BI          PZR.CV          ANA1            ANA2            ANA3            DIG.stat1_01    DIG.stat1_02    DIG.stat1_03    DIG.stat1_04    DIG.stat1_05    DIG.stat1_06    DIG.stat1_07    DIG.stat1_08    DIG.stat1_09    DIG.stat1_10    DIG.stat1_11    DIG.stat1_12    DIG.stat1_13    DIG.stat1_14    DIG.stat1_15    DIG.stat1_16    \u0001\u0000\u0000\u0000\u0000\u0000\u0000\u0000\u0001\u0000\u0000\u0000\u0000\u0000\u0000\u0000\u0001\u0000\u0000\u0000\u0000\u0000\u0000\u0000\u0000\u0000\u0000\u0000\u0000\u0000\u0000\u0000\u0000\u0000\u0000\u0000ÿÿ\u0000\u0000\u0000\u0000\u0000\u0000", "PMU.028\u0000\u0000\u0000\u0000\u0000\u0000\u0000\u0000\u0000\u0000\u001c\u0000\u000f\u0000\u0006\u0000\u0003\u0000\u0001PZR.AI          PZR.BV          PZR.CI          PZR.AV          PZR.BI          PZR.CV          ANA1            ANA2            ANA3            DIG.stat1_01    DIG.stat1_02    DIG.stat1_03    DIG.stat1_04    DIG.stat1_05    DIG.stat1_06    DIG.stat1_07    DIG.stat1_08    DIG.stat1_09    DIG.stat1_10    DIG.stat1_11    DIG.stat1_12    DIG.stat1_13    DIG.stat1_14    DIG.stat1_15    DIG.stat1_16    \u0001\u0000\u0000\u0000\u0000\u0000\u0000\u0000\u0001\u0000\u0000\u0000\u0000\u0000\u0000\u0000\u0001\u0000\u0000\u0000\u0000\u0000\u0000\u0000\u0000\u0000\u0000\u0000\u0000\u0000\u0000\u0000\u0000\u0000\u0000\u0000ÿÿ\u0000\u0000\u0000\u0000\u0000\u0000", "PMU.029\u0000\u0000\u0000\u0000\u0000\u0000\u0000\u0000\u0000\u0000\u001d\u0000\u000f\u0000\u0006\u0000\u0003\u0000\u0001PZR.AI          PZR.BV          PZR.CI          PZR.AV          PZR.BI          PZR.CV          ANA1            ANA2            ANA3            DIG.stat1_01    DIG.stat1_02    DIG.stat1_03    DIG.stat1_04    DIG.stat1_05    DIG.stat1_06    DIG.stat1_07    DIG.stat1_08    DIG.stat1_09    DIG.stat1_10    DIG.stat1_11    DIG.stat1_12    DIG.stat1_13    DIG.stat1_14    DIG.stat1_15    DIG.stat1_16    \u0001\u0000\u0000\u0000\u0000\u0000\u0000\u0000\u0001\u0000\u0000\u0000\u0000\u0000\u0000\u0000\u0001\u0000\u0000\u0000\u0000\u0000\u0000\u0000\u0000\u0000\u0000\u0000\u0000\u0000\u0000\u0000\u0000\u0000\u0000\u0000ÿÿ\u0000\u0000\u0000\u0000\u0000\u0000", "PMU.030\u0000\u0000\u0000\u0000\u0000\u0000\u0000\u0000\u0000\u0000\u001e\u0000\u000f\u0000\u0006\u0000\u0003\u0000\u0001PZR.AI          PZR.BV          PZR.CI          PZR.AV          PZR.BI          PZR.CV          ANA1            ANA2            ANA3            DIG.stat1_01    DIG.stat1_02    DIG.stat1_03    DIG.stat1_04    DIG.stat1_05    DIG.stat1_06    DIG.stat1_07    DIG.stat1_08    DIG.stat1_09    DIG.stat1_10    DIG.stat1_11    DIG.stat1_12    DIG.stat1_13    DIG.stat1_14    DIG.stat1_15    DIG.stat1_16    \u0001\u0000\u0000\u0000\u0000\u0000\u0000\u0000\u0001\u0000\u0000\u0000\u0000\u0000\u0000\u0000\u0001\u0000\u0000\u0000\u0000\u0000\u0000\u0000\u0000\u0000\u0000\u0000\u0000\u0000\u0000\u0000\u0000\u0000\u0000\u0000ÿÿ\u0000\u0000\u0000\u0000\u0000\u0000", "PMU.031\u0000\u0000\u0000\u0000\u0000\u0000\u0000\u0000\u0000\u0000\u001f\u0000\u000f\u0000\u0006\u0000\u0003\u0000\u0001PZR.AI          PZR.BV          PZR.CI          PZR.AV          PZR.BI          PZR.CV          ANA1            ANA2            ANA3            DIG.stat1_01    DIG.stat1_02    DIG.stat1_03    DIG.stat1_04    DIG.stat1_05    DIG.stat1_06    DIG.stat1_07    DIG.stat1_08    DIG.stat1_09    DIG.stat1_10    DIG.stat1_11    DIG.stat1_12    DIG.stat1_13    DIG.stat1_14    DIG.stat1_15    DIG.stat1_16    \u0001\u0000\u0000\u0000\u0000\u0000\u0000\u0000\u0001\u0000\u0000\u0000\u0000\u0000\u0000\u0000\u0001\u0000\u0000\u0000\u0000\u0000\u0000\u0000\u0000\u0000\u0000\u0000\u0000\u0000\u0000\u0000\u0000\u0000\u0000\u0000ÿÿ\u0000\u0000\u0000\u0000\u0000\u0000", "PMU.032\u0000\u0000\u0000\u0000\u0000\u0000\u0000\u0000\u0000\u0000 \u0000\u000f\u0000\u0006\u0000\u0003\u0000\u0001PZR.AI          PZR.BV          PZR.CI          PZR.AV          PZR.BI          PZR.CV          ANA1            ANA2            ANA3            DIG.stat1_01    DIG.stat1_02    DIG.stat1_03    DIG.stat1_04    DIG.stat1_05    DIG.stat1_06    DIG.stat1_07    DIG.stat1_08    DIG.stat1_09    DIG.stat1_10    DIG.stat1_11    DIG.stat1_12    DIG.stat1_13    DIG.stat1_14    DIG.stat1_15    DIG.stat1_16    \u0001\u0000\u0000\u0000\u0000\u0000\u0000\u0000\u0001\u0000\u0000\u0000\u0000\u0000\u0000\u0000\u0001\u0000\u0000\u0000\u0000\u0000\u0000\u0000\u0000\u0000\u0000\u0000\u0000\u0000\u0000\u0000\u0000\u0000\u0000\u0000ÿÿ\u0000\u0000\u0000\u0000\u0000\u0000", "PMU.033\u0000\u0000\u0000\u0000\u0000\u0000\u0000\u0000\u0000\u0000!\u0000\u000f\u0000\u0006\u0000\u0003\u0000\u0001PZR.AI          PZR.BV          PZR.CI          PZR.AV          PZR.BI          PZR.CV          ANA1            ANA2            ANA3            DIG.stat1_01    DIG.stat1_02    DIG.stat1_03    DIG.stat1_04    DIG.stat1_05    DIG.stat1_06    DIG.stat1_07    DIG.stat1_08    DIG.stat1_09    DIG.stat1_10    DIG.stat1_11    DIG.stat1_12    DIG.stat1_13    DIG.stat1_14    DIG.stat1_15    DIG.stat1_16    \u0001\u0000\u0000\u0000\u0000\u0000\u0000\u0000\u0001\u0000\u0000\u0000\u0000\u0000\u0000\u0000\u0001\u0000\u0000\u0000\u0000\u0000\u0000\u0000\u0000\u0000\u0000\u0000\u0000\u0000\u0000\u0000\u0000\u0000\u0000\u0000ÿÿ\u0000\u0000\u0000\u0000\u0000\u0000", "PMU.034\u0000\u0000\u0000\u0000\u0000\u0000\u0000\u0000\u0000\u0000\"\u0000\u000f\u0000\u0006\u0000\u0003\u0000\u0001PZR.AI          PZR.BV          PZR.CI          PZR.AV          PZR.BI          PZR.CV          ANA1            ANA2            ANA3            DIG.stat1_01    DIG.stat1_02    DIG.stat1_03    DIG.stat1_04    DIG.stat1_05    DIG.stat1_06    DIG.stat1_07    DIG.stat1_08    DIG.stat1_09    DIG.stat1_10    DIG.stat1_11    DIG.stat1_12    DIG.stat1_13    DIG.stat1_14    DIG.stat1_15    DIG.stat1_16    \u0001\u0000\u0000\u0000\u0000\u0000\u0000\u0000\u0001\u0000\u0000\u0000\u0000\u0000\u0000\u0000\u0001\u0000\u0000\u0000\u0000\u0000\u0000\u0000\u0000\u0000\u0000\u0000\u0000\u0000\u0000\u0000\u0000\u0000\u0000\u0000ÿÿ\u0000\u0000\u0000\u0000\u0000\u0000", "PMU.035\u0000\u0000\u0000\u0000\u0000\u0000\u0000\u0000\u0000\u0000#\u0000\u000f\u0000\u0006\u0000\u0003\u0000\u0001PZR.AI          PZR.BV          PZR.CI          PZR.AV          PZR.BI          PZR.CV          ANA1            ANA2            ANA3            DIG.stat1_01    DIG.stat1_02    DIG.stat1_03    DIG.stat1_04    DIG.stat1_05    DIG.stat1_06    DIG.stat1_07    DIG.stat1_08    DIG.stat1_09    DIG.stat1_10    DIG.stat1_11    DIG.stat1_12    DIG.stat1_13    DIG.stat1_14    DIG.stat1_15    DIG.stat1_16    \u0001\u0000\u0000\u0000\u0000\u0000\u0000\u0000\u0001\u0000\u0000\u0000\u0000\u0000\u0000\u0000\u0001\u0000\u0000\u0000\u0000\u0000\u0000\u0000\u0000\u0000\u0000\u0000\u0000\u0000\u0000\u0000\u0000\u0000\u0000\u0000ÿÿ\u0000\u0000\u0000\u0000\u0000\u0000", "PMU.036\u0000\u0000\u0000\u0000\u0000\u0000\u0000\u0000\u0000\u0000$\u0000\u000f\u0000\u0006\u0000\u0003\u0000\u0001PZR.AI          PZR.BV          PZR.CI          PZR.AV          PZR.BI          PZR.CV          ANA1            ANA2            ANA3            DIG.stat1_01    DIG.stat1_02    DIG.stat1_03    DIG.stat1_04    DIG.stat1_05    DIG.stat1_06    DIG.stat1_07    DIG.stat1_08    DIG.stat1_09    DIG.stat1_10    DIG.stat1_11    DIG.stat1_12    DIG.stat1_13    DIG.stat1_14    DIG.stat1_15    DIG.stat1_16    \u0001\u0000\u0000\u0000\u0000\u0000\u0000\u0000\u0001\u0000\u0000\u0000\u0000\u0000\u0000\u0000\u0001\u0000\u0000\u0000\u0000\u0000\u0000\u0000\u0000\u0000\u0000\u0000\u0000\u0000\u0000\u0000\u0000\u0000\u0000\u0000ÿÿ\u0000\u0000\u0000\u0000\u0000\u0000", "PMU.037\u0000\u0000\u0000\u0000\u0000\u0000\u0000\u0000\u0000\u0000%\u0000\u000f\u0000\u0006\u0000\u0003\u0000\u0001PZR.AI          PZR.BV          PZR.CI          PZR.AV          PZR.BI          PZR.CV          ANA1            ANA2            ANA3            DIG.stat1_01    DIG.stat1_02    DIG.stat1_03    DIG.stat1_04    DIG.stat1_05    DIG.stat1_06    DIG.stat1_07    DIG.stat1_08    DIG.stat1_09    DIG.stat1_10    DIG.stat1_11    DIG.stat1_12    DIG.stat1_13    DIG.stat1_14    DIG.stat1_15    DIG.stat1_16    \u0001\u0000\u0000\u0000\u0000\u0000\u0000\u0000\u0001\u0000\u0000\u0000\u0000\u0000\u0000\u0000\u0001\u0000\u0000\u0000\u0000\u0000\u0000\u0000\u0000\u0000\u0000\u0000\u0000\u0000\u0000\u0000\u0000\u0000\u0000\u0000ÿÿ\u0000\u0000\u0000\u0000\u0000\u0000", "PMU.038\u0000\u0000\u0000\u0000\u0000\u0000\u0000\u0000\u0000\u0000&\u0000\u000f\u0000\u0006\u0000\u0003\u0000\u0001PZR.AI          PZR.BV          PZR.CI          PZR.AV          PZR.BI          PZR.CV          ANA1            ANA2            ANA3            DIG.stat1_01    DIG.stat1_02    DIG.stat1_03    DIG.stat1_04    DIG.stat1_05    DIG.stat1_06    DIG.stat1_07    DIG.stat1_08    DIG.stat1_09    DIG.stat1_10    DIG.stat1_11    DIG.stat1_12    DIG.stat1_13    DIG.stat1_14    DIG.stat1_15    DIG.stat1_16    \u0001\u0000\u0000\u0000\u0000\u0000\u0000\u0000\u0001\u0000\u0000\u0000\u0000\u0000\u0000\u0000\u0001\u0000\u0000\u0000\u0000\u0000\u0000\u0000\u0000\u0000\u0000\u0000\u0000\u0000\u0000\u0000\u0000\u0000\u0000\u0000ÿÿ\u0000\u0000\u0000\u0000\u0000\u0000", "PMU.039\u0000\u0000\u0000\u0000\u0000\u0000\u0000\u0000\u0000\u0000'\u0000\u000f\u0000\u0006\u0000\u0003\u0000\u0001PZR.AI          PZR.BV          PZR.CI          PZR.AV          PZR.BI          PZR.CV          ANA1            ANA2            ANA3            DIG.stat1_01    DIG.stat1_02    DIG.stat1_03    DIG.stat1_04    DIG.stat1_05    DIG.stat1_06    DIG.stat1_07    DIG.stat1_08    DIG.stat1_09    DIG.stat1_10    DIG.stat1_11    DIG.stat1_12    DIG.stat1_13    DIG.stat1_14    DIG.stat1_15    DIG.stat1_16    \u0001\u0000\u0000\u0000\u0000\u0000\u0000\u0000\u0001\u0000\u0000\u0000\u0000\u0000\u0000\u0000\u0001\u0000\u0000\u0000\u0000\u0000\u0000\u0000\u0000\u0000\u0000\u0000\u0000\u0000\u0000\u0000\u0000\u0000\u0000\u0000ÿÿ\u0000\u0000\u0000\u0000\u0000\u0000", "PMU.040\u0000\u0000\u0000\u0000\u0000\u0000\u0000\u0000\u0000\u0000(\u0000\u000f\u0000\u0006\u0000\u0003\u0000\u0001PZR.AI          PZR.BV          PZR.CI          PZR.AV          PZR.BI          PZR.CV          ANA1            ANA2            ANA3            DIG.stat1_01    DIG.stat1_02    DIG.stat1_03    DIG.stat1_04    DIG.stat1_05    DIG.stat1_06    DIG.stat1_07    DIG.stat1_08    DIG.stat1_09    DIG.stat1_10    DIG.stat1_11    DIG.stat1_12    DIG.stat1_13    DIG.stat1_14    DIG.stat1_15    DIG.stat1_16    \u0001\u0000\u0000\u0000\u0000\u0000\u0000\u0000\u0001\u0000\u0000\u0000\u0000\u0000\u0000\u0000\u0001\u0000\u0000\u0000\u0000\u0000\u0000\u0000\u0000\u0000\u0000\u0000\u0000\u0000\u0000\u0000\u0000\u0000\u0000\u0000ÿÿ\u0000\u0000\u0000\u0000\u0000\u0000", "PMU.041\u0000\u0000\u0000\u0000\u0000\u0000\u0000\u0000\u0000\u0000)\u0000\u000f\u0000\u0006\u0000\u0003\u0000\u0001PZR.AI          PZR.BV          PZR.CI          PZR.AV          PZR.BI          PZR.CV          ANA1            ANA2            ANA3            DIG.stat1_01    DIG.stat1_02    DIG.stat1_03    DIG.stat1_04    DIG.stat1_05    DIG.stat1_06    DIG.stat1_07    DIG.stat1_08    DIG.stat1_09    DIG.stat1_10    DIG.stat1_11    DIG.stat1_12    DIG.stat1_13    DIG.stat1_14    DIG.stat1_15    DIG.stat1_16    \u0001\u0000\u0000\u0000\u0000\u0000\u0000\u0000\u0001\u0000\u0000\u0000\u0000\u0000\u0000\u0000\u0001\u0000\u0000\u0000\u0000\u0000\u0000\u0000\u0000\u0000\u0000\u0000\u0000\u0000\u0000\u0000\u0000\u0000\u0000\u0000ÿÿ\u0000\u0000\u0000\u0000\u0000\u0000", "PMU.042\u0000\u0000\u0000\u0000\u0000\u0000\u0000\u0000\u0000\u0000*\u0000\u000f\u0000\u0006\u0000\u0003\u0000\u0001PZR.AI          PZR.BV          PZR.CI          PZR.AV          PZR.BI          PZR.CV          ANA1            ANA2            ANA3            DIG.stat1_01    DIG.stat1_02    DIG.stat1_03    DIG.stat1_04    DIG.stat1_05    DIG.stat1_06    DIG.stat1_07    DIG.stat1_08    DIG.stat1_09    DIG.stat1_10    DIG.stat1_11    DIG.stat1_12    DIG.stat1_13    DIG.stat1_14    DIG.stat1_15    DIG.stat1_16    \u0001\u0000\u0000\u0000\u0000\u0000\u0000\u0000\u0001\u0000\u0000\u0000\u0000\u0000\u0000\u0000\u0001\u0000\u0000\u0000\u0000\u0000\u0000\u0000\u0000\u0000\u0000\u0000\u0000\u0000\u0000\u0000\u0000\u0000\u0000\u0000ÿÿ\u0000\u0000\u0000\u0000\u0000\u0000", "PMU.043\u0000\u0000\u0000\u0000\u0000\u0000\u0000\u0000\u0000\u0000+\u0000\u000f\u0000\u0006\u0000\u0003\u0000\u0001PZR.AI          PZR.BV          PZR.CI          PZR.AV          PZR.BI          PZR.CV          ANA1            ANA2            ANA3            DIG.stat1_01    DIG.stat1_02    DIG.stat1_03    DIG.stat1_04    DIG.stat1_05    DIG.stat1_06    DIG.stat1_07    DIG.stat1_08    DIG.stat1_09    DIG.stat1_10    DIG.stat1_11    DIG.stat1_12    DIG.stat1_13    DIG.stat1_14    DIG.stat1_15    DIG.stat1_16    \u0001\u0000\u0000\u0000\u0000\u0000\u0000\u0000\u0001\u0000\u0000\u0000\u0000\u0000\u0000\u0000\u0001\u0000\u0000\u0000\u0000\u0000\u0000\u0000\u0000\u0000\u0000\u0000\u0000\u0000\u0000\u0000\u0000\u0000\u0000\u0000ÿÿ\u0000\u0000\u0000\u0000\u0000\u0000", "PMU.044\u0000\u0000\u0000\u0000\u0000\u0000\u0000\u0000\u0000\u0000,\u0000\u000f\u0000\u0006\u0000\u0003\u0000\u0001PZR.AI          PZR.BV          PZR.CI          PZR.AV          PZR.BI          PZR.CV          ANA1            ANA2            ANA3            DIG.stat1_01    DIG.stat1_02    DIG.stat1_03    DIG.stat1_04    DIG.stat1_05    DIG.stat1_06    DIG.stat1_07    DIG.stat1_08    DIG.stat1_09    DIG.stat1_10    DIG.stat1_11    DIG.stat1_12    DIG.stat1_13    DIG.stat1_14    DIG.stat1_15    DIG.stat1_16    \u0001\u0000\u0000\u0000\u0000\u0000\u0000\u0000\u0001\u0000\u0000\u0000\u0000\u0000\u0000\u0000\u0001\u0000\u0000\u0000\u0000\u0000\u0000\u0000\u0000\u0000\u0000\u0000\u0000\u0000\u0000\u0000\u0000\u0000\u0000\u0000ÿÿ\u0000\u0000\u0000\u0000\u0000\u0000", "PMU.045\u0000\u0000\u0000\u0000\u0000\u0000\u0000\u0000\u0000\u0000-\u0000\u000f\u0000\u0006\u0000\u0003\u0000\u0001PZR.AI          PZR.BV          PZR.CI          PZR.AV          PZR.BI          PZR.CV          ANA1            ANA2            ANA3            DIG.stat1_01    DIG.stat1_02    DIG.stat1_03    DIG.stat1_04    DIG.stat1_05    DIG.stat1_06    DIG.stat1_07    DIG.stat1_08    DIG.stat1_09    DIG.stat1_10    DIG.stat1_11    DIG.stat1_12    DIG.stat1_13    DIG.stat1_14    DIG.stat1_15    DIG.stat1_16    \u0001\u0000\u0000\u0000\u0000\u0000\u0000\u0000\u0001\u0000\u0000\u0000\u0000\u0000\u0000\u0000\u0001\u0000\u0000\u0000\u0000\u0000\u0000\u0000\u0000\u0000\u0000\u0000\u0000\u0000\u0000\u0000\u0000\u0000\u0000\u0000ÿÿ\u0000\u0000\u0000\u0000\u0000\u0000", "PMU.046\u0000\u0000\u0000\u0000\u0000\u0000\u0000\u0000\u0000\u0000.\u0000\u000f\u0000\u0006\u0000\u0003\u0000\u0001PZR.AI          PZR.BV          PZR.CI          PZR.AV          PZR.BI          PZR.CV          ANA1            ANA2            ANA3            DIG.stat1_01    DIG.stat1_02    DIG.stat1_03    DIG.stat1_04    DIG.stat1_05    DIG.stat1_06    DIG.stat1_07    DIG.stat1_08    DIG.stat1_09    DIG.stat1_10    DIG.stat1_11    DIG.stat1_12    DIG.stat1_13    DIG.stat1_14    DIG.stat1_15    DIG.stat1_16    \u0001\u0000\u0000\u0000\u0000\u0000\u0000\u0000\u0001\u0000\u0000\u0000\u0000\u0000\u0000\u0000\u0001\u0000\u0000\u0000\u0000\u0000\u0000\u0000\u0000\u0000\u0000\u0000\u0000\u0000\u0000\u0000\u0000\u0000\u0000\u0000ÿÿ\u0000\u0000\u0000\u0000\u0000\u0000", "PMU.047\u0000\u0000\u0000\u0000\u0000\u0000\u0000\u0000\u0000\u0000/\u0000\u000f\u0000\u0006\u0000\u0003\u0000\u0001PZR.AI          PZR.BV          PZR.CI          PZR.AV          PZR.BI          PZR.CV          ANA1            ANA2            ANA3            DIG.stat1_01    DIG.stat1_02    DIG.stat1_03    DIG.stat1_04    DIG.stat1_05    DIG.stat1_06    DIG.stat1_07    DIG.stat1_08    DIG.stat1_09    DIG.stat1_10    DIG.stat1_11    DIG.stat1_12    DIG.stat1_13    DIG.stat1_14    DIG.stat1_15    DIG.stat1_16    \u0001\u0000\u0000\u0000\u0000\u0000\u0000\u0000\u0001\u0000\u0000\u0000\u0000\u0000\u0000\u0000\u0001\u0000\u0000\u0000\u0000\u0000\u0000\u0000\u0000\u0000\u0000\u0000\u0000\u0000\u0000\u0000\u0000\u0000\u0000\u0000ÿÿ\u0000\u0000\u0000\u0000\u0000\u0000", "PMU.048\u0000\u0000\u0000\u0000\u0000\u0000\u0000\u0000\u0000\u00000\u0000\u000f\u0000\u0006\u0000\u0003\u0000\u0001PZR.AI          PZR.BV          PZR.CI          PZR.AV          PZR.BI          PZR.CV          ANA1            ANA2            ANA3            DIG.stat1_01    DIG.stat1_02    DIG.stat1_03    DIG.stat1_04    DIG.stat1_05    DIG.stat1_06    DIG.stat1_07    DIG.stat1_08    DIG.stat1_09    DIG.stat1_10    DIG.stat1_11    DIG.stat1_12    DIG.stat1_13    DIG.stat1_14    DIG.stat1_15    DIG.stat1_16    \u0001\u0000\u0000\u0000\u0000\u0000\u0000\u0000\u0001\u0000\u0000\u0000\u0000\u0000\u0000\u0000\u0001\u0000\u0000\u0000\u0000\u0000\u0000\u0000\u0000\u0000\u0000\u0000\u0000\u0000\u0000\u0000\u0000\u0000\u0000\u0000ÿÿ\u0000\u0000\u0000\u0000\u0000\u0000", "PMU.049\u0000\u0000\u0000\u0000\u0000\u0000\u0000\u0000\u0000\u00001\u0000\u000f\u0000\u0006\u0000\u0003\u0000\u0001PZR.AI          PZR.BV          PZR.CI          PZR.AV          PZR.BI          PZR.CV          ANA1            ANA2            ANA3            DIG.stat1_01    DIG.stat1_02    DIG.stat1_03    DIG.stat1_04    DIG.stat1_05    DIG.stat1_06    DIG.stat1_07    DIG.stat1_08    DIG.stat1_09    DIG.stat1_10    DIG.stat1_11    DIG.stat1_12    DIG.stat1_13    DIG.stat1_14    DIG.stat1_15    DIG.stat1_16    \u0001\u0000\u0000\u0000\u0000\u0000\u0000\u0000\u0001\u0000\u0000\u0000\u0000\u0000\u0000\u0000\u0001\u0000\u0000\u0000\u0000\u0000\u0000\u0000\u0000\u0000\u0000\u0000\u0000\u0000\u0000\u0000\u0000\u0000\u0000\u0000ÿÿ\u0000\u0000\u0000\u0000\u0000\u0000", "PMU.050\u0000\u0000\u0000\u0000\u0000\u0000\u0000\u0000\u0000\u00002\u0000\u000f\u0000\u0006\u0000\u0003\u0000\u0001PZR.AI          PZR.BV          PZR.CI          PZR.AV          PZR.BI          PZR.CV          ANA1            ANA2            ANA3            DIG.stat1_01    DIG.stat1_02    DIG.stat1_03    DIG.stat1_04    DIG.stat1_05    DIG.stat1_06    DIG.stat1_07    DIG.stat1_08    DIG.stat1_09    DIG.stat1_10    DIG.stat1_11    DIG.stat1_12    DIG.stat1_13    DIG.stat1_14    DIG.stat1_15    DIG.stat1_16    \u0001\u0000\u0000\u0000\u0000\u0000\u0000\u0000\u0001\u0000\u0000\u0000\u0000\u0000\u0000\u0000\u0001\u0000\u0000\u0000\u0000\u0000\u0000\u0000\u0000\u0000\u0000\u0000\u0000\u0000\u0000\u0000\u0000\u0000\u0000\u0000ÿÿ\u0000\u0000\u0000\u0000\u0000\u0000", "PMU.051\u0000\u0000\u0000\u0000\u0000\u0000\u0000\u0000\u0000\u00003\u0000\u000f\u0000\u0006\u0000\u0003\u0000\u0001PZR.AI          PZR.BV          PZR.CI          PZR.AV          PZR.BI          PZR.CV          ANA1            ANA2            ANA3            DIG.stat1_01    DIG.stat1_02    DIG.stat1_03    DIG.stat1_04    DIG.stat1_05    DIG.stat1_06    DIG.stat1_07    DIG.stat1_08    DIG.stat1_09    DIG.stat1_10    DIG.stat1_11    DIG.stat1_12    DIG.stat1_13    DIG.stat1_14    DIG.stat1_15    DIG.stat1_16    \u0001\u0000\u0000\u0000\u0000\u0000\u0000\u0000\u0001\u0000\u0000\u0000\u0000\u0000\u0000\u0000\u0001\u0000\u0000\u0000\u0000\u0000\u0000\u0000\u0000\u0000\u0000\u0000\u0000\u0000\u0000\u0000\u0000\u0000\u0000\u0000ÿÿ\u0000\u0000\u0000\u0000\u0000\u0000", "PMU.052\u0000\u0000\u0000\u0000\u0000\u0000\u0000\u0000\u0000\u00004\u0000\u000f\u0000\u0006\u0000\u0003\u0000\u0001PZR.AI          PZR.BV          PZR.CI          PZR.AV          PZR.BI          PZR.CV          ANA1            ANA2            ANA3            DIG.stat1_01    DIG.stat1_02    DIG.stat1_03    DIG.stat1_04    DIG.stat1_05    DIG.stat1_06    DIG.stat1_07    DIG.stat1_08    DIG.stat1_09    DIG.stat1_10    DIG.stat1_11    DIG.stat1_12    DIG.stat1_13    DIG.stat1_14    DIG.stat1_15    DIG.stat1_16    \u0001\u0000\u0000\u0000\u0000\u0000\u0000\u0000\u0001\u0000\u0000\u0000\u0000\u0000\u0000\u0000\u0001\u0000\u0000\u0000\u0000\u0000\u0000\u0000\u0000\u0000\u0000\u0000\u0000\u0000\u0000\u0000\u0000\u0000\u0000\u0000ÿÿ\u0000\u0000\u0000\u0000\u0000\u0000", "PMU.053\u0000\u0000\u0000\u0000\u0000\u0000\u0000\u0000\u0000\u00005\u0000\u000f\u0000\u0006\u0000\u0003\u0000\u0001PZR.AI          PZR.BV          PZR.CI          PZR.AV          PZR.BI          PZR.CV          ANA1            ANA2            ANA3            DIG.stat1_01    DIG.stat1_02    DIG.stat1_03    DIG.stat1_04    DIG.stat1_05    DIG.stat1_06    DIG.stat1_07    DIG.stat1_08    DIG.stat1_09    DIG.stat1_10    DIG.stat1_11    DIG.stat1_12    DIG.stat1_13    DIG.stat1_14    DIG.stat1_15    DIG.stat1_16    \u0001\u0000\u0000\u0000\u0000\u0000\u0000\u0000\u0001\u0000\u0000\u0000\u0000\u0000\u0000\u0000\u0001\u0000\u0000\u0000\u0000\u0000\u0000\u0000\u0000\u0000\u0000\u0000\u0000\u0000\u0000\u0000\u0000\u0000\u0000\u0000ÿÿ\u0000\u0000\u0000\u0000\u0000\u0000", "PMU.054\u0000\u0000\u0000\u0000\u0000\u0000\u0000\u0000\u0000\u00006\u0000\u000f\u0000\u0006\u0000\u0003\u0000\u0001PZR.AI          PZR.BV          PZR.CI          PZR.AV          PZR.BI          PZR.CV          ANA1            ANA2            ANA3            DIG.stat1_01    DIG.stat1_02    DIG.stat1_03    DIG.stat1_04    DIG.stat1_05    DIG.stat1_06    DIG.stat1_07    DIG.stat1_08    DIG.stat1_09    DIG.stat1_10    DIG.stat1_11    DIG.stat1_12    DIG.stat1_13    DIG.stat1_14    DIG.stat1_15    DIG.stat1_16    \u0001\u0000\u0000\u0000\u0000\u0000\u0000\u0000\u0001\u0000\u0000\u0000\u0000\u0000\u0000\u0000\u0001\u0000\u0000\u0000\u0000\u0000\u0000\u0000\u0000\u0000\u0000\u0000\u0000\u0000\u0000\u0000\u0000\u0000\u0000\u0000ÿÿ\u0000\u0000\u0000\u0000\u0000\u0000", "PMU.055\u0000\u0000\u0000\u0000\u0000\u0000\u0000\u0000\u0000\u00007\u0000\u000f\u0000\u0006\u0000\u0003\u0000\u0001PZR.AI          PZR.BV          PZR.CI          PZR.AV          PZR.BI          PZR.CV          ANA1            ANA2            ANA3            DIG.stat1_01    DIG.stat1_02    DIG.stat1_03    DIG.stat1_04    DIG.stat1_05    DIG.stat1_06    DIG.stat1_07    DIG.stat1_08    DIG.stat1_09    DIG.stat1_10    DIG.stat1_11    DIG.stat1_12    DIG.stat1_13    DIG.stat1_14    DIG.stat1_15    DIG.stat1_16    \u0001\u0000\u0000\u0000\u0000\u0000\u0000\u0000\u0001\u0000\u0000\u0000\u0000\u0000\u0000\u0000\u0001\u0000\u0000\u0000\u0000\u0000\u0000\u0000\u0000\u0000\u0000\u0000\u0000\u0000\u0000\u0000\u0000\u0000\u0000\u0000ÿÿ\u0000\u0000\u0000\u0000\u0000\u0000", "PMU.056\u0000\u0000\u0000\u0000\u0000\u0000\u0000\u0000\u0000\u00008\u0000\u000f\u0000\u0006\u0000\u0003\u0000\u0001PZR.AI          PZR.BV          PZR.CI          PZR.AV          PZR.BI          PZR.CV          ANA1            ANA2            ANA3            DIG.stat1_01    DIG.stat1_02    DIG.stat1_03    DIG.stat1_04    DIG.stat1_05    DIG.stat1_06    DIG.stat1_07    DIG.stat1_08    DIG.stat1_09    DIG.stat1_10    DIG.stat1_11    DIG.stat1_12    DIG.stat1_13    DIG.stat1_14    DIG.stat1_15    DIG.stat1_16    \u0001\u0000\u0000\u0000\u0000\u0000\u0000\u0000\u0001\u0000\u0000\u0000\u0000\u0000\u0000\u0000\u0001\u0000\u0000\u0000\u0000\u0000\u0000\u0000\u0000\u0000\u0000\u0000\u0000\u0000\u0000\u0000\u0000\u0000\u0000\u0000ÿÿ\u0000\u0000\u0000\u0000\u0000\u0000", "PMU.057\u0000\u0000\u0000\u0000\u0000\u0000\u0000\u0000\u0000\u00009\u0000\u000f\u0000\u0006\u0000\u0003\u0000\u0001PZR.AI          PZR.BV          PZR.CI          PZR.AV          PZR.BI          PZR.CV          ANA1            ANA2            ANA3            DIG.stat1_01    DIG.stat1_02    DIG.stat1_03    DIG.stat1_04    DIG.stat1_05    DIG.stat1_06    DIG.stat1_07    DIG.stat1_08    DIG.stat1_09    DIG.stat1_10    DIG.stat1_11    DIG.stat1_12    DIG.stat1_13    DIG.stat1_14    DIG.stat1_15    DIG.stat1_16    \u0001\u0000\u0000\u0000\u0000\u0000\u0000\u0000\u0001\u0000\u0000\u0000\u0000\u0000\u0000\u0000\u0001\u0000\u0000\u0000\u0000\u0000\u0000\u0000\u0000\u0000\u0000\u0000\u0000\u0000\u0000\u0000\u0000\u0000\u0000\u0000ÿÿ\u0000\u0000\u0000\u0000\u0000\u0000", "PMU.058\u0000\u0000\u0000\u0000\u0000\u0000\u0000\u0000\u0000\u0000:\u0000\u000f\u0000\u0006\u0000\u0003\u0000\u0001PZR.AI          PZR.BV          PZR.CI          PZR.AV          PZR.BI          PZR.CV          ANA1            ANA2            ANA3            DIG.stat1_01    DIG.stat1_02    DIG.stat1_03    DIG.stat1_04    DIG.stat1_05    DIG.stat1_06    DIG.stat1_07    DIG.stat1_08    DIG.stat1_09    DIG.stat1_10    DIG.stat1_11    DIG.stat1_12    DIG.stat1_13    DIG.stat1_14    DIG.stat1_15    DIG.stat1_16    \u0001\u0000\u0000\u0000\u0000\u0000\u0000\u0000\u0001\u0000\u0000\u0000\u0000\u0000\u0000\u0000\u0001\u0000\u0000\u0000\u0000\u0000\u0000\u0000\u0000\u0000\u0000\u0000\u0000\u0000\u0000\u0000\u0000\u0000\u0000\u0000ÿÿ\u0000\u0000\u0000\u0000\u0000\u0000", "PMU.059\u0000\u0000\u0000\u0000\u0000\u0000\u0000\u0000\u0000\u0000;\u0000\u000f\u0000\u0006\u0000\u0003\u0000\u0001PZR.AI          PZR.BV          PZR.CI          PZR.AV          PZR.BI          PZR.CV          ANA1            ANA2            ANA3            DIG.stat1_01    DIG.stat1_02    DIG.stat1_03    DIG.stat1_04    DIG.stat1_05    DIG.stat1_06    DIG.stat1_07    DIG.stat1_08    DIG.stat1_09    DIG.stat1_10    DIG.stat1_11    DIG.stat1_12    DIG.stat1_13    DIG.stat1_14    DIG.stat1_15    DIG.stat1_16    \u0001\u0000\u0000\u0000\u0000\u0000\u0000\u0000\u0001\u0000\u0000\u0000\u0000\u0000\u0000\u0000\u0001\u0000\u0000\u0000\u0000\u0000\u0000\u0000\u0000\u0000\u0000\u0000\u0000\u0000\u0000\u0000\u0000\u0000\u0000\u0000ÿÿ\u0000\u0000\u0000\u0000\u0000\u0000", "PMU.060\u0000\u0000\u0000\u0000\u0000\u0000\u0000\u0000\u0000\u0000<\u0000\u000f\u0000\u0006\u0000\u0003\u0000\u0001PZR.AI          PZR.BV          PZR.CI          PZR.AV          PZR.BI          PZR.CV          ANA1            ANA2            ANA3            DIG.stat1_01    DIG.stat1_02    DIG.stat1_03    DIG.stat1_04    DIG.stat1_05    DIG.stat1_06    DIG.stat1_07    DIG.stat1_08    DIG.stat1_09    DIG.stat1_10    DIG.stat1_11    DIG.stat1_12    DIG.stat1_13    DIG.stat1_14    DIG.stat1_15    DIG.stat1_16    \u0001\u0000\u0000\u0000\u0000\u0000\u0000\u0000\u0001\u0000\u0000\u0000\u0000\u0000\u0000\u0000\u0001\u0000\u0000\u0000\u0000\u0000\u0000\u0000\u0000\u0000\u0000\u0000\u0000\u0000\u0000\u0000\u0000\u0000\u0000\u0000ÿÿ\u0000\u0000\u0000\u0000\u0000\u0000", "PMU.061\u0000\u0000\u0000\u0000\u0000\u0000\u0000\u0000\u0000\u0000=\u0000\u000f\u0000\u0006\u0000\u0003\u0000\u0001PZR.AI          PZR.BV          PZR.CI          PZR.AV          PZR.BI          PZR.CV          ANA1            ANA2            ANA3            DIG.stat1_01    DIG.stat1_02    DIG.stat1_03    DIG.stat1_04    DIG.stat1_05    DIG.stat1_06    DIG.stat1_07    DIG.stat1_08    DIG.stat1_09    DIG.stat1_10    DIG.stat1_11    DIG.stat1_12    DIG.stat1_13    DIG.stat1_14    DIG.stat1_15    DIG.stat1_16    \u0001\u0000\u0000\u0000\u0000\u0000\u0000\u0000\u0001\u0000\u0000\u0000\u0000\u0000\u0000\u0000\u0001\u0000\u0000\u0000\u0000\u0000\u0000\u0000\u0000\u0000\u0000\u0000\u0000\u0000\u0000\u0000\u0000\u0000\u0000\u0000ÿÿ\u0000\u0000\u0000\u0000\u0000\u0000", "PMU.062\u0000\u0000\u0000\u0000\u0000\u0000\u0000\u0000\u0000\u0000>\u0000\u000f\u0000\u0006\u0000\u0003\u0000\u0001PZR.AI          PZR.BV          PZR.CI          PZR.AV          PZR.BI          PZR.CV          ANA1            ANA2            ANA3            DIG.stat1_01    DIG.stat1_02    DIG.stat1_03    DIG.stat1_04    DIG.stat1_05    DIG.stat1_06    DIG.stat1_07    DIG.stat1_08    DIG.stat1_09    DIG.stat1_10    DIG.stat1_11    DIG.stat1_12    DIG.stat1_13    DIG.stat1_14    DIG.stat1_15    DIG.stat1_16    \u0001\u0000\u0000\u0000\u0000\u0000\u0000\u0000\u0001\u0000\u0000\u0000\u0000\u0000\u0000\u0000\u0001\u0000\u0000\u0000\u0000\u0000\u0000\u0000\u0000\u0000\u0000\u0000\u0000\u0000\u0000\u0000\u0000\u0000\u0000\u0000ÿÿ\u0000\u0000\u0000\u0000\u0000\u0000", "PMU.063\u0000\u0000\u0000\u0000\u0000\u0000\u0000\u0000\u0000\u0000?\u0000\u000f\u0000\u0006\u0000\u0003\u0000\u0001PZR.AI          PZR.BV          PZR.CI          PZR.AV          PZR.BI          PZR.CV          ANA1            ANA2            ANA3            DIG.stat1_01    DIG.stat1_02    DIG.stat1_03    DIG.stat1_04    DIG.stat1_05    DIG.stat1_06    DIG.stat1_07    DIG.stat1_08    DIG.stat1_09    DIG.stat1_10    DIG.stat1_11    DIG.stat1_12    DIG.stat1_13    DIG.stat1_14    DIG.stat1_15    DIG.stat1_16    \u0001\u0000\u0000\u0000\u0000\u0000\u0000\u0000\u0001\u0000\u0000\u0000\u0000\u0000\u0000\u0000\u0001\u0000\u0000\u0000\u0000\u0000\u0000\u0000\u0000\u0000\u0000\u0000\u0000\u0000\u0000\u0000\u0000\u0000\u0000\u0000ÿÿ\u0000\u0000\u0000\u0000\u0000\u0000", "PMU.064\u0000\u0000\u0000\u0000\u0000\u0000\u0000\u0000\u0000\u0000@\u0000\u000f\u0000\u0006\u0000\u0003\u0000\u0001PZR.AI          PZR.BV          PZR.CI          PZR.AV          PZR.BI          PZR.CV          ANA1            ANA2            ANA3            DIG.stat1_01    DIG.stat1_02    DIG.stat1_03    DIG.stat1_04    DIG.stat1_05    DIG.stat1_06    DIG.stat1_07    DIG.stat1_08    DIG.stat1_09    DIG.stat1_10    DIG.stat1_11    DIG.stat1_12    DIG.stat1_13    DIG.stat1_14    DIG.stat1_15    DIG.stat1_16    \u0001\u0000\u0000\u0000\u0000\u0000\u0000\u0000\u0001\u0000\u0000\u0000\u0000\u0000\u0000\u0000\u0001\u0000\u0000\u0000\u0000\u0000\u0000\u0000\u0000\u0000\u0000\u0000\u0000\u0000\u0000\u0000\u0000\u0000\u0000\u0000ÿÿ\u0000\u0000\u0000\u0000\u0000\u0000", "PMU.065\u0000\u0000\u0000\u0000\u0000\u0000\u0000\u0000\u0000\u0000A\u0000\u000f\u0000\u0006\u0000\u0003\u0000\u0001PZR.AI          PZR.BV          PZR.CI          PZR.AV          PZR.BI          PZR.CV          ANA1            ANA2            ANA3            DIG.stat1_01    DIG.stat1_02    DIG.stat1_03    DIG.stat1_04    DIG.stat1_05    DIG.stat1_06    DIG.stat1_07    DIG.stat1_08    DIG.stat1_09    DIG.stat1_10    DIG.stat1_11    DIG.stat1_12    DIG.stat1_13    DIG.stat1_14    DIG.stat1_15    DIG.stat1_16    \u0001\u0000\u0000\u0000\u0000\u0000\u0000\u0000\u0001\u0000\u0000\u0000\u0000\u0000\u0000\u0000\u0001\u0000\u0000\u0000\u0000\u0000\u0000\u0000\u0000\u0000\u0000\u0000\u0000\u0000\u0000\u0000\u0000\u0000\u0000\u0000ÿÿ\u0000\u0000\u0000\u0000\u0000\u0000", "PMU.066\u0000\u0000\u0000\u0000\u0000\u0000\u0000\u0000\u0000\u0000B\u0000\u000f\u0000\u0006\u0000\u0003\u0000\u0001PZR.AI          PZR.BV          PZR.CI          PZR.AV          PZR.BI          PZR.CV          ANA1            ANA2            ANA3            DIG.stat1_01    DIG.stat1_02    DIG.stat1_03    DIG.stat1_04    DIG.stat1_05    DIG.stat1_06    DIG.stat1_07    DIG.stat1_08    DIG.stat1_09    DIG.stat1_10    DIG.stat1_11    DIG.stat1_12    DIG.stat1_13    DIG.stat1_14    DIG.stat1_15    DIG.stat1_16    \u0001\u0000\u0000\u0000\u0000\u0000\u0000\u0000\u0001\u0000\u0000\u0000\u0000\u0000\u0000\u0000\u0001\u0000\u0000\u0000\u0000\u0000\u0000\u0000\u0000\u0000\u0000\u0000\u0000\u0000\u0000\u0000\u0000\u0000\u0000\u0000ÿÿ\u0000\u0000\u0000\u0000\u0000\u0000", "PMU.067\u0000\u0000\u0000\u0000\u0000\u0000\u0000\u0000\u0000\u0000C\u0000\u000f\u0000\u0006\u0000\u0003\u0000\u0001PZR.AI          PZR.BV          PZR.CI          PZR.AV          PZR.BI          PZR.CV          ANA1            ANA2            ANA3            DIG.stat1_01    DIG.stat1_02    DIG.stat1_03    DIG.stat1_04    DIG.stat1_05    DIG.stat1_06    DIG.stat1_07    DIG.stat1_08    DIG.stat1_09    DIG.stat1_10    DIG.stat1_11    DIG.stat1_12    DIG.stat1_13    DIG.stat1_14    DIG.stat1_15    DIG.stat1_16    \u0001\u0000\u0000\u0000\u0000\u0000\u0000\u0000\u0001\u0000\u0000\u0000\u0000\u0000\u0000\u0000\u0001\u0000\u0000\u0000\u0000\u0000\u0000\u0000\u0000\u0000\u0000\u0000\u0000\u0000\u0000\u0000\u0000\u0000\u0000\u0000ÿÿ\u0000\u0000\u0000\u0000\u0000\u0000", "PMU.068\u0000\u0000\u0000\u0000\u0000\u0000\u0000\u0000\u0000\u0000D\u0000\u000f\u0000\u0006\u0000\u0003\u0000\u0001PZR.AI          PZR.BV          PZR.CI          PZR.AV          PZR.BI          PZR.CV          ANA1            ANA2            ANA3            DIG.stat1_01    DIG.stat1_02    DIG.stat1_03    DIG.stat1_04    DIG.stat1_05    DIG.stat1_06    DIG.stat1_07    DIG.stat1_08    DIG.stat1_09    DIG.stat1_10    DIG.stat1_11    DIG.stat1_12    DIG.stat1_13    DIG.stat1_14    DIG.stat1_15    DIG.stat1_16    \u0001\u0000\u0000\u0000\u0000\u0000\u0000\u0000\u0001\u0000\u0000\u0000\u0000\u0000\u0000\u0000\u0001\u0000\u0000\u0000\u0000\u0000\u0000\u0000\u0000\u0000\u0000\u0000\u0000\u0000\u0000\u0000\u0000\u0000\u0000\u0000ÿÿ\u0000\u0000\u0000\u0000\u0000\u0000", "PMU.069\u0000\u0000\u0000\u0000\u0000\u0000\u0000\u0000\u0000\u0000E\u0000\u000f\u0000\u0006\u0000\u0003\u0000\u0001PZR.AI          PZR.BV          PZR.CI          PZR.AV          PZR.BI          PZR.CV          ANA1            ANA2            ANA3            DIG.stat1_01    DIG.stat1_02    DIG.stat1_03    DIG.stat1_04    DIG.stat1_05    DIG.stat1_06    DIG.stat1_07    DIG.stat1_08    DIG.stat1_09    DIG.stat1_10    DIG.stat1_11    DIG.stat1_12    DIG.stat1_13    DIG.stat1_14    DIG.stat1_15    DIG.stat1_16    \u0001\u0000\u0000\u0000\u0000\u0000\u0000\u0000\u0001\u0000\u0000\u0000\u0000\u0000\u0000\u0000\u0001\u0000\u0000\u0000\u0000\u0000\u0000\u0000\u0000\u0000\u0000\u0000\u0000\u0000\u0000\u0000\u0000\u0000\u0000\u0000ÿÿ\u0000\u0000\u0000\u0000\u0000\u0000", "PMU.070\u0000\u0000\u0000\u0000\u0000\u0000\u0000\u0000\u0000\u0000F\u0000\u000f\u0000\u0006\u0000\u0003\u0000\u0001PZR.AI          PZR.BV          PZR.CI          PZR.AV          PZR.BI          PZR.CV          ANA1            ANA2            ANA3            DIG.stat1_01    DIG.stat1_02    DIG.stat1_03    DIG.stat1_04    DIG.stat1_05    DIG.stat1_06    DIG.stat1_07    DIG.stat1_08    DIG.stat1_09    DIG.stat1_10    DIG.stat1_11    DIG.stat1_12    DIG.stat1_13    DIG.stat1_14    DIG.stat1_15    DIG.stat1_16    \u0001\u0000\u0000\u0000\u0000\u0000\u0000\u0000\u0001\u0000\u0000\u0000\u0000\u0000\u0000\u0000\u0001\u0000\u0000\u0000\u0000\u0000\u0000\u0000\u0000\u0000\u0000\u0000\u0000\u0000\u0000\u0000\u0000\u0000\u0000\u0000ÿÿ\u0000\u0000\u0000\u0000\u0000\u0000", "PMU.071\u0000\u0000\u0000\u0000\u0000\u0000\u0000\u0000\u0000\u0000G\u0000\u000f\u0000\u0006\u0000\u0003\u0000\u0001PZR.AI          PZR.BV          PZR.CI          PZR.AV          PZR.BI          PZR.CV          ANA1            ANA2            ANA3            DIG.stat1_01    DIG.stat1_02    DIG.stat1_03    DIG.stat1_04    DIG.stat1_05    DIG.stat1_06    DIG.stat1_07    DIG.stat1_08    DIG.stat1_09    DIG.stat1_10    DIG.stat1_11    DIG.stat1_12    DIG.stat1_13    DIG.stat1_14    DIG.stat1_15    DIG.stat1_16    \u0001\u0000\u0000\u0000\u0000\u0000\u0000\u0000\u0001\u0000\u0000\u0000\u0000\u0000\u0000\u0000\u0001\u0000\u0000\u0000\u0000\u0000\u0000\u0000\u0000\u0000\u0000\u0000\u0000\u0000\u0000\u0000\u0000\u0000\u0000\u0000ÿÿ\u0000\u0000\u0000\u0000\u0000\u0000", "PMU.072\u0000\u0000\u0000\u0000\u0000\u0000\u0000\u0000\u0000\u0000H\u0000\u000f\u0000\u0006\u0000\u0003\u0000\u0001PZR.AI          PZR.BV          PZR.CI          PZR.AV          PZR.BI          PZR.CV          ANA1            ANA2            ANA3            DIG.stat1_01    DIG.stat1_02    DIG.stat1_03    DIG.stat1_04    DIG.stat1_05    DIG.stat1_06    DIG.stat1_07    DIG.stat1_08    DIG.stat1_09    DIG.stat1_10    DIG.stat1_11    DIG.stat1_12    DIG.stat1_13    DIG.stat1_14    DIG.stat1_15    DIG.stat1_16    \u0001\u0000\u0000\u0000\u0000\u0000\u0000\u0000\u0001\u0000\u0000\u0000\u0000\u0000\u0000\u0000\u0001\u0000\u0000\u0000\u0000\u0000\u0000\u0000\u0000\u0000\u0000\u0000\u0000\u0000\u0000\u0000\u0000\u0000\u0000\u0000ÿÿ\u0000\u0000\u0000\u0000\u0000\u0000", "PMU.073\u0000\u0000\u0000\u0000\u0000\u0000\u0000\u0000\u0000\u0000I\u0000\u000f\u0000\u0006\u0000\u0003\u0000\u0001PZR.AI          PZR.BV          PZR.CI          PZR.AV          PZR.BI          PZR.CV          ANA1            ANA2            ANA3            DIG.stat1_01    DIG.stat1_02    DIG.stat1_03    DIG.stat1_04    DIG.stat1_05    DIG.stat1_06    DIG.stat1_07    DIG.stat1_08    DIG.stat1_09    DIG.stat1_10    DIG.stat1_11    DIG.stat1_12    DIG.stat1_13    DIG.stat1_14    DIG.stat1_15    DIG.stat1_16    \u0001\u0000\u0000\u0000\u0000\u0000\u0000\u0000\u0001\u0000\u0000\u0000\u0000\u0000\u0000\u0000\u0001\u0000\u0000\u0000\u0000\u0000\u0000\u0000\u0000\u0000\u0000\u0000\u0000\u0000\u0000\u0000\u0000\u0000\u0000\u0000ÿÿ\u0000\u0000\u0000\u0000\u0000\u0000", "PMU.074\u0000\u0000\u0000\u0000\u0000\u0000\u0000\u0000\u0000\u0000J\u0000\u000f\u0000\u0006\u0000\u0003\u0000\u0001PZR.AI          PZR.BV          PZR.CI          PZR.AV          PZR.BI          PZR.CV          ANA1            ANA2            ANA3            DIG.stat1_01    DIG.stat1_02    DIG.stat1_03    DIG.stat1_04    DIG.stat1_05    DIG.stat1_06    DIG.stat1_07    DIG.stat1_08    DIG.stat1_09    DIG.stat1_10    DIG.stat1_11    DIG.stat1_12    DIG.stat1_13    DIG.stat1_14    DIG.stat1_15    DIG.stat1_16    \u0001\u0000\u0000\u0000\u0000\u0000\u0000\u0000\u0001\u0000\u0000\u0000\u0000\u0000\u0000\u0000\u0001\u0000\u0000\u0000\u0000\u0000\u0000\u0000\u0000\u0000\u0000\u0000\u0000\u0000\u0000\u0000\u0000\u0000\u0000\u0000ÿÿ\u0000\u0000\u0000\u0000\u0000\u0000", "PMU.075\u0000\u0000\u0000\u0000\u0000\u0000\u0000\u0000\u0000\u0000K\u0000\u000f\u0000\u0006\u0000\u0003\u0000\u0001PZR.AI          PZR.BV          PZR.CI          PZR.AV          PZR.BI          PZR.CV          ANA1            ANA2            ANA3            DIG.stat1_01    DIG.stat1_02    DIG.stat1_03    DIG.stat1_04    DIG.stat1_05    DIG.stat1_06    DIG.stat1_07    DIG.stat1_08    DIG.stat1_09    DIG.stat1_10    DIG.stat1_11    DIG.stat1_12    DIG.stat1_13    DIG.stat1_14    DIG.stat1_15    DIG.stat1_16    \u0001\u0000\u0000\u0000\u0000\u0000\u0000\u0000\u0001\u0000\u0000\u0000\u0000\u0000\u0000\u0000\u0001\u0000\u0000\u0000\u0000\u0000\u0000\u0000\u0000\u0000\u0000\u0000\u0000\u0000\u0000\u0000\u0000\u0000\u0000\u0000ÿÿ\u0000\u0000\u0000\u0000\u0000\u0000", "PMU.076\u0000\u0000\u0000\u0000\u0000\u0000\u0000\u0000\u0000\u0000L\u0000\u000f\u0000\u0006\u0000\u0003\u0000\u0001PZR.AI          PZR.BV          PZR.CI          PZR.AV          PZR.BI          PZR.CV          ANA1            ANA2            ANA3            DIG.stat1_01    DIG.stat1_02    DIG.stat1_03    DIG.stat1_04    DIG.stat1_05    DIG.stat1_06    DIG.stat1_07    DIG.stat1_08    DIG.stat1_09    DIG.stat1_10    DIG.stat1_11    DIG.stat1_12    DIG.stat1_13    DIG.stat1_14    DIG.stat1_15    DIG.stat1_16    \u0001\u0000\u0000\u0000\u0000\u0000\u0000\u0000\u0001\u0000\u0000\u0000\u0000\u0000\u0000\u0000\u0001\u0000\u0000\u0000\u0000\u0000\u0000\u0000\u0000\u0000\u0000\u0000\u0000\u0000\u0000\u0000\u0000\u0000\u0000\u0000ÿÿ\u0000\u0000\u0000\u0000\u0000\u0000", "PMU.077\u0000\u0000\u0000\u0000\u0000\u0000\u0000\u0000\u0000\u0000M\u0000\u000f\u0000\u0006\u0000\u0003\u0000\u0001PZR.AI          PZR.BV          PZR.CI          PZR.AV          PZR.BI          PZR.CV          ANA1            ANA2            ANA3            DIG.stat1_01    DIG.stat1_02    DIG.stat1_03    DIG.stat1_04    DIG.stat1_05    DIG.stat1_06    DIG.stat1_07    DIG.stat1_08    DIG.stat1_09    DIG.stat1_10    DIG.stat1_11    DIG.stat1_12    DIG.stat1_13    DIG.stat1_14    DIG.stat1_15    DIG.stat1_16    \u0001\u0000\u0000\u0000\u0000\u0000\u0000\u0000\u0001\u0000\u0000\u0000\u0000\u0000\u0000\u0000\u0001\u0000\u0000\u0000\u0000\u0000\u0000\u0000\u0000\u0000\u0000\u0000\u0000\u0000\u0000\u0000\u0000\u0000\u0000\u0000ÿÿ\u0000\u0000\u0000\u0000\u0000\u0000", "PMU.078\u0000\u0000\u0000\u0000\u0000\u0000\u0000\u0000\u0000\u0000N\u0000\u000f\u0000\u0006\u0000\u0003\u0000\u0001PZR.AI          PZR.BV          PZR.CI          PZR.AV          PZR.BI          PZR.CV          ANA1            ANA2            ANA3            DIG.stat1_01    DIG.stat1_02    DIG.stat1_03    DIG.stat1_04    DIG.stat1_05    DIG.stat1_06    DIG.stat1_07    DIG.stat1_08    DIG.stat1_09    DIG.stat1_10    DIG.stat1_11    DIG.stat1_12    DIG.stat1_13    DIG.stat1_14    DIG.stat1_15    DIG.stat1_16    \u0001\u0000\u0000\u0000\u0000\u0000\u0000\u0000\u0001\u0000\u0000\u0000\u0000\u0000\u0000\u0000\u0001\u0000\u0000\u0000\u0000\u0000\u0000\u0000\u0000\u0000\u0000\u0000\u0000\u0000\u0000\u0000\u0000\u0000\u0000\u0000ÿÿ\u0000\u0000\u0000\u0000\u0000\u0000", "PMU.079\u0000\u0000\u0000\u0000\u0000\u0000\u0000\u0000\u0000\u0000O\u0000\u000f\u0000\u0006\u0000\u0003\u0000\u0001PZR.AI          PZR.BV          PZR.CI          PZR.AV          PZR.BI          PZR.CV          ANA1            ANA2            ANA3            DIG.stat1_01    DIG.stat1_02    DIG.stat1_03    DIG.stat1_04    DIG.stat1_05    DIG.stat1_06    DIG.stat1_07    DIG.stat1_08    DIG.stat1_09    DIG.stat1_10    DIG.stat1_11    DIG.stat1_12    DIG.stat1_13    DIG.stat1_14    DIG.stat1_15    DIG.stat1_16    \u0001\u0000\u0000\u0000\u0000\u0000\u0000\u0000\u0001\u0000\u0000\u0000\u0000\u0000\u0000\u0000\u0001\u0000\u0000\u0000\u0000\u0000\u0000\u0000\u0000\u0000\u0000\u0000\u0000\u0000\u0000\u0000\u0000\u0000\u0000\u0000ÿÿ\u0000\u0000\u0000\u0000\u0000\u0000", "PMU.080\u0000\u0000\u0000\u0000\u0000\u0000\u0000\u0000\u0000\u0000P\u0000\u000f\u0000\u0006\u0000\u0003\u0000\u0001PZR.AI          PZR.BV          PZR.CI          PZR.AV          PZR.BI          PZR.CV          ANA1            ANA2            ANA3            DIG.stat1_01    DIG.stat1_02    DIG.stat1_03    DIG.stat1_04    DIG.stat1_05    DIG.stat1_06    DIG.stat1_07    DIG.stat1_08    DIG.stat1_09    DIG.stat1_10    DIG.stat1_11    DIG.stat1_12    DIG.stat1_13    DIG.stat1_14    DIG.stat1_15    DIG.stat1_16    \u0001\u0000\u0000\u0000\u0000\u0000\u0000\u0000\u0001\u0000\u0000\u0000\u0000\u0000\u0000\u0000\u0001\u0000\u0000\u0000\u0000\u0000\u0000\u0000\u0000\u0000\u0000\u0000\u0000\u0000\u0000\u0000\u0000\u0000\u0000\u0000ÿÿ\u0000\u0000\u0000\u0000\u0000\u0000", "PMU.081\u0000\u0000\u0000\u0000\u0000\u0000\u0000\u0000\u0000\u0000Q\u0000\u000f\u0000\u0006\u0000\u0003\u0000\u0001PZR.AI          PZR.BV          PZR.CI          PZR.AV          PZR.BI          PZR.CV          ANA1            ANA2            ANA3            DIG.stat1_01    DIG.stat1_02    DIG.stat1_03    DIG.stat1_04    DIG.stat1_05    DIG.stat1_06    DIG.stat1_07    DIG.stat1_08    DIG.stat1_09    DIG.stat1_10    DIG.stat1_11    DIG.stat1_12    DIG.stat1_13    DIG.stat1_14    DIG.stat1_15    DIG.stat1_16    \u0001\u0000\u0000\u0000\u0000\u0000\u0000\u0000\u0001\u0000\u0000\u0000\u0000\u0000\u0000\u0000\u0001\u0000\u0000\u0000\u0000\u0000\u0000\u0000\u0000\u0000\u0000\u0000\u0000\u0000\u0000\u0000\u0000\u0000\u0000\u0000ÿÿ\u0000\u0000\u0000\u0000\u0000\u0000", "PMU.082\u0000\u0000\u0000\u0000\u0000\u0000\u0000\u0000\u0000\u0000R\u0000\u000f\u0000\u0006\u0000\u0003\u0000\u0001PZR.AI          PZR.BV          PZR.CI          PZR.AV          PZR.BI          PZR.CV          ANA1            ANA2            ANA3            DIG.stat1_01    DIG.stat1_02    DIG.stat1_03    DIG.stat1_04    DIG.stat1_05    DIG.stat1_06    DIG.stat1_07    DIG.stat1_08    DIG.stat1_09    DIG.stat1_10    DIG.stat1_11    DIG.stat1_12    DIG.stat1_13    DIG.stat1_14    DIG.stat1_15    DIG.stat1_16    \u0001\u0000\u0000\u0000\u0000\u0000\u0000\u0000\u0001\u0000\u0000\u0000\u0000\u0000\u0000\u0000\u0001\u0000\u0000\u0000\u0000\u0000\u0000\u0000\u0000\u0000\u0000\u0000\u0000\u0000\u0000\u0000\u0000\u0000\u0000\u0000ÿÿ\u0000\u0000\u0000\u0000\u0000\u0000", "PMU.083\u0000\u0000\u0000\u0000\u0000\u0000\u0000\u0000\u0000\u0000S\u0000\u000f\u0000\u0006\u0000\u0003\u0000\u0001PZR.AI          PZR.BV          PZR.CI          PZR.AV          PZR.BI          PZR.CV          ANA1            ANA2            ANA3            DIG.stat1_01    DIG.stat1_02    DIG.stat1_03    DIG.stat1_04    DIG.stat1_05    DIG.stat1_06    DIG.stat1_07    DIG.stat1_08    DIG.stat1_09    DIG.stat1_10    DIG.stat1_11    DIG.stat1_12    DIG.stat1_13    DIG.stat1_14    DIG.stat1_15    DIG.stat1_16    \u0001\u0000\u0000\u0000\u0000\u0000\u0000\u0000\u0001\u0000\u0000\u0000\u0000\u0000\u0000\u0000\u0001\u0000\u0000\u0000\u0000\u0000\u0000\u0000\u0000\u0000\u0000\u0000\u0000\u0000\u0000\u0000\u0000\u0000\u0000\u0000ÿÿ\u0000\u0000\u0000\u0000\u0000\u0000", "PMU.084\u0000\u0000\u0000\u0000\u0000\u0000\u0000\u0000\u0000\u0000T\u0000\u000f\u0000\u0006\u0000\u0003\u0000\u0001PZR.AI          PZR.BV          PZR.CI          PZR.AV          PZR.BI          PZR.CV          ANA1            ANA2            ANA3            DIG.stat1_01    DIG.stat1_02    DIG.stat1_03    DIG.stat1_04    DIG.stat1_05    DIG.stat1_06    DIG.stat1_07    DIG.stat1_08    DIG.stat1_09    DIG.stat1_10    DIG.stat1_11    DIG.stat1_12    DIG.stat1_13    DIG.stat1_14    DIG.stat1_15    DIG.stat1_16    \u0001\u0000\u0000\u0000\u0000\u0000\u0000\u0000\u0001\u0000\u0000\u0000\u0000\u0000\u0000\u0000\u0001\u0000\u0000\u0000\u0000\u0000\u0000\u0000\u0000\u0000\u0000\u0000\u0000\u0000\u0000\u0000\u0000\u0000\u0000\u0000ÿÿ\u0000\u0000\u0000\u0000\u0000\u0000", "PMU.085\u0000\u0000\u0000\u0000\u0000\u0000\u0000\u0000\u0000\u0000U\u0000\u000f\u0000\u0006\u0000\u0003\u0000\u0001PZR.AI          PZR.BV          PZR.CI          PZR.AV          PZR.BI          PZR.CV          ANA1            ANA2            ANA3            DIG.stat1_01    DIG.stat1_02    DIG.stat1_03    DIG.stat1_04    DIG.stat1_05    DIG.stat1_06    DIG.stat1_07    DIG.stat1_08    DIG.stat1_09    DIG.stat1_10    DIG.stat1_11    DIG.stat1_12    DIG.stat1_13    DIG.stat1_14    DIG.stat1_15    DIG.stat1_16    \u0001\u0000\u0000\u0000\u0000\u0000\u0000\u0000\u0001\u0000\u0000\u0000\u0000\u0000\u0000\u0000\u0001\u0000\u0000\u0000\u0000\u0000\u0000\u0000\u0000\u0000\u0000\u0000\u0000\u0000\u0000\u0000\u0000\u0000\u0000\u0000ÿÿ\u0000\u0000\u0000\u0000\u0000\u0000", "PMU.086\u0000\u0000\u0000\u0000\u0000\u0000\u0000\u0000\u0000\u0000V\u0000\u000f\u0000\u0006\u0000\u0003\u0000\u0001PZR.AI          PZR.BV          PZR.CI          PZR.AV          PZR.BI          PZR.CV          ANA1            ANA2            ANA3            DIG.stat1_01    DIG.stat1_02    DIG.stat1_03    DIG.stat1_04    DIG.stat1_05    DIG.stat1_06    DIG.stat1_07    DIG.stat1_08    DIG.stat1_09    DIG.stat1_10    DIG.stat1_11    DIG.stat1_12    DIG.stat1_13    DIG.stat1_14    DIG.stat1_15    DIG.stat1_16    \u0001\u0000\u0000\u0000\u0000\u0000\u0000\u0000\u0001\u0000\u0000\u0000\u0000\u0000\u0000\u0000\u0001\u0000\u0000\u0000\u0000\u0000\u0000\u0000\u0000\u0000\u0000\u0000\u0000\u0000\u0000\u0000\u0000\u0000\u0000\u0000ÿÿ\u0000\u0000\u0000\u0000\u0000\u0000", "PMU.087\u0000\u0000\u0000\u0000\u0000\u0000\u0000\u0000\u0000\u0000W\u0000\u000f\u0000\u0006\u0000\u0003\u0000\u0001PZR.AI          PZR.BV          PZR.CI          PZR.AV          PZR.BI          PZR.CV          ANA1            ANA2            ANA3            DIG.stat1_01    DIG.stat1_02    DIG.stat1_03    DIG.stat1_04    DIG.stat1_05    DIG.stat1_06    DIG.stat1_07    DIG.stat1_08    DIG.stat1_09    DIG.stat1_10    DIG.stat1_11    DIG.stat1_12    DIG.stat1_13    DIG.stat1_14    DIG.stat1_15    DIG.stat1_16    \u0001\u0000\u0000\u0000\u0000\u0000\u0000\u0000\u0001\u0000\u0000\u0000\u0000\u0000\u0000\u0000\u0001\u0000\u0000\u0000\u0000\u0000\u0000\u0000\u0000\u0000\u0000\u0000\u0000\u0000\u0000\u0000\u0000\u0000\u0000\u0000ÿÿ\u0000\u0000\u0000\u0000\u0000\u0000", "PMU.088\u0000\u0000\u0000\u0000\u0000\u0000\u0000\u0000\u0000\u0000X\u0000\u000f\u0000\u0006\u0000\u0003\u0000\u0001PZR.AI          PZR.BV          PZR.CI          PZR.AV          PZR.BI          PZR.CV          ANA1            ANA2            ANA3            DIG.stat1_01    DIG.stat1_02    DIG.stat1_03    DIG.stat1_04    DIG.stat1_05    DIG.stat1_06    DIG.stat1_07    DIG.stat1_08    DIG.stat1_09    DIG.stat1_10    DIG.stat1_11    DIG.stat1_12    DIG.stat1_13    DIG.stat1_14    DIG.stat1_15    DIG.stat1_16    \u0001\u0000\u0000\u0000\u0000\u0000\u0000\u0000\u0001\u0000\u0000\u0000\u0000\u0000\u0000\u0000\u0001\u0000\u0000\u0000\u0000\u0000\u0000\u0000\u0000\u0000\u0000\u0000\u0000\u0000\u0000\u0000\u0000\u0000\u0000\u0000ÿÿ\u0000\u0000\u0000\u0000\u0000\u0000", "PMU.089\u0000\u0000\u0000\u0000\u0000\u0000\u0000\u0000\u0000\u0000Y\u0000\u000f\u0000\u0006\u0000\u0003\u0000\u0001PZR.AI          PZR.BV          PZR.CI          PZR.AV          PZR.BI          PZR.CV          ANA1            ANA2            ANA3            DIG.stat1_01    DIG.stat1_02    DIG.stat1_03    DIG.stat1_04    DIG.stat1_05    DIG.stat1_06    DIG.stat1_07    DIG.stat1_08    DIG.stat1_09    DIG.stat1_10    DIG.stat1_11    DIG.stat1_12    DIG.stat1_13    DIG.stat1_14    DIG.stat1_15    DIG.stat1_16    \u0001\u0000\u0000\u0000\u0000\u0000\u0000\u0000\u0001\u0000\u0000\u0000\u0000\u0000\u0000\u0000\u0001\u0000\u0000\u0000\u0000\u0000\u0000\u0000\u0000\u0000\u0000\u0000\u0000\u0000\u0000\u0000\u0000\u0000\u0000\u0000ÿÿ\u0000\u0000\u0000\u0000\u0000\u0000", "PMU.090\u0000\u0000\u0000\u0000\u0000\u0000\u0000\u0000\u0000\u0000Z\u0000\u000f\u0000\u0006\u0000\u0003\u0000\u0001PZR.AI          PZR.BV          PZR.CI          PZR.AV          PZR.BI          PZR.CV          ANA1            ANA2            ANA3            DIG.stat1_01    DIG.stat1_02    DIG.stat1_03    DIG.stat1_04    DIG.stat1_05    DIG.stat1_06    DIG.stat1_07    DIG.stat1_08    DIG.stat1_09    DIG.stat1_10    DIG.stat1_11    DIG.stat1_12    DIG.stat1_13    DIG.stat1_14    DIG.stat1_15    DIG.stat1_16    \u0001\u0000\u0000\u0000\u0000\u0000\u0000\u0000\u0001\u0000\u0000\u0000\u0000\u0000\u0000\u0000\u0001\u0000\u0000\u0000\u0000\u0000\u0000\u0000\u0000\u0000\u0000\u0000\u0000\u0000\u0000\u0000\u0000\u0000\u0000\u0000ÿÿ\u0000\u0000\u0000\u0000\u0000\u0000", "PMU.091\u0000\u0000\u0000\u0000\u0000\u0000\u0000\u0000\u0000\u0000[\u0000\u000f\u0000\u0006\u0000\u0003\u0000\u0001PZR.AI          PZR.BV          PZR.CI          PZR.AV          PZR.BI          PZR.CV          ANA1            ANA2            ANA3            DIG.stat1_01    DIG.stat1_02    DIG.stat1_03    DIG.stat1_04    DIG.stat1_05    DIG.stat1_06    DIG.stat1_07    DIG.stat1_08    DIG.stat1_09    DIG.stat1_10    DIG.stat1_11    DIG.stat1_12    DIG.stat1_13    DIG.stat1_14    DIG.stat1_15    DIG.stat1_16    \u0001\u0000\u0000\u0000\u0000\u0000\u0000\u0000\u0001\u0000\u0000\u0000\u0000\u0000\u0000\u0000\u0001\u0000\u0000\u0000\u0000\u0000\u0000\u0000\u0000\u0000\u0000\u0000\u0000\u0000\u0000\u0000\u0000\u0000\u0000\u0000ÿÿ\u0000\u0000\u0000\u0000\u0000\u0000", "PMU.092\u0000\u0000\u0000\u0000\u0000\u0000\u0000\u0000\u0000\u0000\\\u0000\u000f\u0000\u0006\u0000\u0003\u0000\u0001PZR.AI          PZR.BV          PZR.CI          PZR.AV          PZR.BI          PZR.CV          ANA1            ANA2            ANA3            DIG.stat1_01    DIG.stat1_02    DIG.stat1_03    DIG.stat1_04    DIG.stat1_05    DIG.stat1_06    DIG.stat1_07    DIG.stat1_08    DIG.stat1_09    DIG.stat1_10    DIG.stat1_11    DIG.stat1_12    DIG.stat1_13    DIG.stat1_14    DIG.stat1_15    DIG.stat1_16    \u0001\u0000\u0000\u0000\u0000\u0000\u0000\u0000\u0001\u0000\u0000\u0000\u0000\u0000\u0000\u0000\u0001\u0000\u0000\u0000\u0000\u0000\u0000\u0000\u0000\u0000\u0000\u0000\u0000\u0000\u0000\u0000\u0000\u0000\u0000\u0000ÿÿ\u0000\u0000\u0000\u0000\u0000\u0000", "PMU.093\u0000\u0000\u0000\u0000\u0000\u0000\u0000\u0000\u0000\u0000]\u0000\u000f\u0000\u0006\u0000\u0003\u0000\u0001PZR.AI          PZR.BV          PZR.CI          PZR.AV          PZR.BI          PZR.CV          ANA1            ANA2            ANA3            DIG.stat1_01    DIG.stat1_02    DIG.stat1_03    DIG.stat1_04    DIG.stat1_05    DIG.stat1_06    DIG.stat1_07    DIG.stat1_08    DIG.stat1_09    DIG.stat1_10    DIG.stat1_11    DIG.stat1_12    DIG.stat1_13    DIG.stat1_14    DIG.stat1_15    DIG.stat1_16    \u0001\u0000\u0000\u0000\u0000\u0000\u0000\u0000\u0001\u0000\u0000\u0000\u0000\u0000\u0000\u0000\u0001\u0000\u0000\u0000\u0000\u0000\u0000\u0000\u0000\u0000\u0000\u0000\u0000\u0000\u0000\u0000\u0000\u0000\u0000\u0000ÿÿ\u0000\u0000\u0000\u0000\u0000\u0000", "PMU.094\u0000\u0000\u0000\u0000\u0000\u0000\u0000\u0000\u0000\u0000^\u0000\u000f\u0000\u0006\u0000\u0003\u0000\u0001PZR.AI          PZR.BV          PZR.CI          PZR.AV          PZR.BI          PZR.CV          ANA1            ANA2            ANA3            DIG.stat1_01    DIG.stat1_02    DIG.stat1_03    DIG.stat1_04    DIG.stat1_05    DIG.stat1_06    DIG.stat1_07    DIG.stat1_08    DIG.stat1_09    DIG.stat1_10    DIG.stat1_11    DIG.stat1_12    DIG.stat1_13    DIG.stat1_14    DIG.stat1_15    DIG.stat1_16    \u0001\u0000\u0000\u0000\u0000\u0000\u0000\u0000\u0001\u0000\u0000\u0000\u0000\u0000\u0000\u0000\u0001\u0000\u0000\u0000\u0000\u0000\u0000\u0000\u0000\u0000\u0000\u0000\u0000\u0000\u0000\u0000\u0000\u0000\u0000\u0000ÿÿ\u0000\u0000\u0000\u0000\u0000\u0000", "PMU.095\u0000\u0000\u0000\u0000\u0000\u0000\u0000\u0000\u0000\u0000_\u0000\u000f\u0000\u0006\u0000\u0003\u0000\u0001PZR.AI          PZR.BV          PZR.CI          PZR.AV          PZR.BI          PZR.CV          ANA1            ANA2            ANA3            DIG.stat1_01    DIG.stat1_02    DIG.stat1_03    DIG.stat1_04    DIG.stat1_05    DIG.stat1_06    DIG.stat1_07    DIG.stat1_08    DIG.stat1_09    DIG.stat1_10    DIG.stat1_11    DIG.stat1_12    DIG.stat1_13    DIG.stat1_14    DIG.stat1_15    DIG.stat1_16    \u0001\u0000\u0000\u0000\u0000\u0000\u0000\u0000\u0001\u0000\u0000\u0000\u0000\u0000\u0000\u0000\u0001\u0000\u0000\u0000\u0000\u0000\u0000\u0000\u0000\u0000\u0000\u0000\u0000\u0000\u0000\u0000\u0000\u0000\u0000\u0000ÿÿ\u0000\u0000\u0000\u0000\u0000\u0000", "PMU.096\u0000\u0000\u0000\u0000\u0000\u0000\u0000\u0000\u0000\u0000`\u0000\u000f\u0000\u0006\u0000\u0003\u0000\u0001PZR.AI          PZR.BV          PZR.CI          PZR.AV          PZR.BI          PZR.CV          ANA1            ANA2            ANA3            DIG.stat1_01    DIG.stat1_02    DIG.stat1_03    DIG.stat1_04    DIG.stat1_05    DIG.stat1_06    DIG.stat1_07    DIG.stat1_08    DIG.stat1_09    DIG.stat1_10    DIG.stat1_11    DIG.stat1_12    DIG.stat1_13    DIG.stat1_14    DIG.stat1_15    DIG.stat1_16    \u0001\u0000\u0000\u0000\u0000\u0000\u0000\u0000\u0001\u0000\u0000\u0000\u0000\u0000\u0000\u0000\u0001\u0000\u0000\u0000\u0000\u0000\u0000\u0000\u0000\u0000\u0000\u0000\u0000\u0000\u0000\u0000\u0000\u0000\u0000\u0000ÿÿ\u0000\u0000\u0000\u0000\u0000\u0000", "PMU.097\u0000\u0000\u0000\u0000\u0000\u0000\u0000\u0000\u0000\u0000a\u0000\u000f\u0000\u0006\u0000\u0003\u0000\u0001PZR.AI          PZR.BV          PZR.CI          PZR.AV          PZR.BI          PZR.CV          ANA1            ANA2            ANA3            DIG.stat1_01    DIG.stat1_02    DIG.stat1_03    DIG.stat1_04    DIG.stat1_05    DIG.stat1_06    DIG.stat1_07    DIG.stat1_08    DIG.stat1_09    DIG.stat1_10    DIG.stat1_11    DIG.stat1_12    DIG.stat1_13    DIG.stat1_14    DIG.stat1_15    DIG.stat1_16    \u0001\u0000\u0000\u0000\u0000\u0000\u0000\u0000\u0001\u0000\u0000\u0000\u0000\u0000\u0000\u0000\u0001\u0000\u0000\u0000\u0000\u0000\u0000\u0000\u0000\u0000\u0000\u0000\u0000\u0000\u0000\u0000\u0000\u0000\u0000\u0000ÿÿ\u0000\u0000\u0000\u0000\u0000\u0000", "PMU.098\u0000\u0000\u0000\u0000\u0000\u0000\u0000\u0000\u0000\u0000b\u0000\u000f\u0000\u0006\u0000\u0003\u0000\u0001PZR.AI          PZR.BV          PZR.CI          PZR.AV          PZR.BI          PZR.CV          ANA1            ANA2            ANA3            DIG.stat1_01    DIG.stat1_02    DIG.stat1_03    DIG.stat1_04    DIG.stat1_05    DIG.stat1_06    DIG.stat1_07    DIG.stat1_08    DIG.stat1_09    DIG.stat1_10    DIG.stat1_11    DIG.stat1_12    DIG.stat1_13    DIG.stat1_14    DIG.stat1_15    DIG.stat1_16    \u0001\u0000\u0000\u0000\u0000\u0000\u0000\u0000\u0001\u0000\u0000\u0000\u0000\u0000\u0000\u0000\u0001\u0000\u0000\u0000\u0000\u0000\u0000\u0000\u0000\u0000\u0000\u0000\u0000\u0000\u0000\u0000\u0000\u0000\u0000\u0000ÿÿ\u0000\u0000\u0000\u0000\u0000\u0000", "PMU.099\u0000\u0000\u0000\u0000\u0000\u0000\u0000\u0000\u0000\u0000c\u0000\u000f\u0000\u0006\u0000\u0003\u0000\u0001PZR.AI          PZR.BV          PZR.CI          PZR.AV          PZR.BI          PZR.CV          ANA1            ANA2            ANA3            DIG.stat1_01    DIG.stat1_02    DIG.stat1_03    DIG.stat1_04    DIG.stat1_05    DIG.stat1_06    DIG.stat1_07    DIG.stat1_08    DIG.stat1_09    DIG.stat1_10    DIG.stat1_11    DIG.stat1_12    DIG.stat1_13    DIG.stat1_14    DIG.stat1_15    DIG.stat1_16    \u0001\u0000\u0000\u0000\u0000\u0000\u0000\u0000\u0001\u0000\u0000\u0000\u0000\u0000\u0000\u0000\u0001\u0000\u0000\u0000\u0000\u0000\u0000\u0000\u0000\u0000\u0000\u0000\u0000\u0000\u0000\u0000\u0000\u0000\u0000\u0000ÿÿ\u0000\u0000\u0000\u0000\u0000\u0000", "PMU.100\u0000\u0000\u0000\u0000\u0000\u0000\u0000\u0000\u0000\u0000d\u0000\u000f\u0000\u0006\u0000\u0003\u0000\u0001PZR.AI          PZR.BV          PZR.CI          PZR.AV          PZR.BI          PZR.CV          ANA1            ANA2            ANA3            DIG.stat1_01    DIG.stat1_02    DIG.stat1_03    DIG.stat1_04    DIG.stat1_05    DIG.stat1_06    DIG.stat1_07    DIG.stat1_08    DIG.stat1_09    DIG.stat1_10    DIG.stat1_11    DIG.stat1_12    DIG.stat1_13    DIG.stat1_14    DIG.stat1_15    DIG.stat1_16    \u0001\u0000\u0000\u0000\u0000\u0000\u0000\u0000\u0001\u0000\u0000\u0000\u0000\u0000\u0000\u0000\u0001\u0000\u0000\u0000\u0000\u0000\u0000\u0000\u0000\u0000\u0000\u0000\u0000\u0000\u0000\u0000\u0000\u0000\u0000\u0000ÿÿ\u0000\u0000\u0000\u0000\u0000\u0000", "PMU.101\u0000\u0000\u0000\u0000\u0000\u0000\u0000\u0000\u0000\u0000e\u0000\u000f\u0000\u0006\u0000\u0003\u0000\u0001PZR.AI          PZR.BV          PZR.CI          PZR.AV          PZR.BI          PZR.CV          ANA1            ANA2            ANA3            DIG.stat1_01    DIG.stat1_02    DIG.stat1_03    DIG.stat1_04    DIG.stat1_05    DIG.stat1_06    DIG.stat1_07    DIG.stat1_08    DIG.stat1_09    DIG.stat1_10    DIG.stat1_11    DIG.stat1_12    DIG.stat1_13    DIG.stat1_14    DIG.stat1_15    DIG.stat1_16    \u0001\u0000\u0000\u0000\u0000\u0000\u0000\u0000\u0001\u0000\u0000\u0000\u0000\u0000\u0000\u0000\u0001\u0000\u0000\u0000\u0000\u0000\u0000\u0000\u0000\u0000\u0000\u0000\u0000\u0000\u0000\u0000\u0000\u0000\u0000\u0000ÿÿ\u0000\u0000\u0000\u0000\u0000\u0000", "PMU.102\u0000\u0000\u0000\u0000\u0000\u0000\u0000\u0000\u0000\u0000f\u0000\u000f\u0000\u0006\u0000\u0003\u0000\u0001PZR.AI          PZR.BV          PZR.CI          PZR.AV          PZR.BI          PZR.CV          ANA1            ANA2            ANA3            DIG.stat1_01    DIG.stat1_02    DIG.stat1_03    DIG.stat1_04    DIG.stat1_05    DIG.stat1_06    DIG.stat1_07    DIG.stat1_08    DIG.stat1_09    DIG.stat1_10    DIG.stat1_11    DIG.stat1_12    DIG.stat1_13    DIG.stat1_14    DIG.stat1_15    DIG.stat1_16    \u0001\u0000\u0000\u0000\u0000\u0000\u0000\u0000\u0001\u0000\u0000\u0000\u0000\u0000\u0000\u0000\u0001\u0000\u0000\u0000\u0000\u0000\u0000\u0000\u0000\u0000\u0000\u0000\u0000\u0000\u0000\u0000\u0000\u0000\u0000\u0000ÿÿ\u0000\u0000\u0000\u0000\u0000\u0000", "PMU.103\u0000\u0000\u0000\u0000\u0000\u0000\u0000\u0000\u0000\u0000g\u0000\u000f\u0000\u0006\u0000\u0003\u0000\u0001PZR.AI          PZR.BV          PZR.CI          PZR.AV          PZR.BI          PZR.CV          ANA1            ANA2            ANA3            DIG.stat1_01    DIG.stat1_02    DIG.stat1_03    DIG.stat1_04    DIG.stat1_05    DIG.stat1_06    DIG.stat1_07    DIG.stat1_08    DIG.stat1_09    DIG.stat1_10    DIG.stat1_11    DIG.stat1_12    DIG.stat1_13    DIG.stat1_14    DIG.stat1_15    DIG.stat1_16    \u0001\u0000\u0000\u0000\u0000\u0000\u0000\u0000\u0001\u0000\u0000\u0000\u0000\u0000\u0000\u0000\u0001\u0000\u0000\u0000\u0000\u0000\u0000\u0000\u0000\u0000\u0000\u0000\u0000\u0000\u0000\u0000\u0000\u0000\u0000\u0000ÿÿ\u0000\u0000\u0000\u0000\u0000\u0000", "PMU.104\u0000\u0000\u0000\u0000\u0000\u0000\u0000\u0000\u0000\u0000h\u0000\u000f\u0000\u0006\u0000\u0003\u0000\u0001PZR.AI          PZR.BV          PZR.CI          PZR.AV          PZR.BI          PZR.CV          ANA1            ANA2            ANA3            DIG.stat1_01    DIG.stat1_02    DIG.stat1_03    DIG.stat1_04    DIG.stat1_05    DIG.stat1_06    DIG.stat1_07    DIG.stat1_08    DIG.stat1_09    DIG.stat1_10    DIG.stat1_11    DIG.stat1_12    DIG.stat1_13    DIG.stat1_14    DIG.stat1_15    DIG.stat1_16    \u0001\u0000\u0000\u0000\u0000\u0000\u0000\u0000\u0001\u0000\u0000\u0000\u0000\u0000\u0000\u0000\u0001\u0000\u0000\u0000\u0000\u0000\u0000\u0000\u0000\u0000\u0000\u0000\u0000\u0000\u0000\u0000\u0000\u0000\u0000\u0000ÿÿ\u0000\u0000\u0000\u0000\u0000\u0000", "PMU.105\u0000\u0000\u0000\u0000\u0000\u0000\u0000\u0000\u0000\u0000i\u0000\u000f\u0000\u0006\u0000\u0003\u0000\u0001PZR.AI          PZR.BV          PZR.CI          PZR.AV          PZR.BI          PZR.CV          ANA1            ANA2            ANA3            DIG.stat1_01    DIG.stat1_02    DIG.stat1_03    DIG.stat1_04    DIG.stat1_05    DIG.stat1_06    DIG.stat1_07    DIG.stat1_08    DIG.stat1_09    DIG.stat1_10    DIG.stat1_11    DIG.stat1_12    DIG.stat1_13    DIG.stat1_14    DIG.stat1_15    DIG.stat1_16    \u0001\u0000\u0000\u0000\u0000\u0000\u0000\u0000\u0001\u0000\u0000\u0000\u0000\u0000\u0000\u0000\u0001\u0000\u0000\u0000\u0000\u0000\u0000\u0000\u0000\u0000\u0000\u0000\u0000\u0000\u0000\u0000\u0000\u0000\u0000\u0000ÿÿ\u0000\u0000\u0000\u0000\u0000\u0000", "PMU.106\u0000\u0000\u0000\u0000\u0000\u0000\u0000\u0000\u0000\u0000j\u0000\u000f\u0000\u0006\u0000\u0003\u0000\u0001PZR.AI          PZR.BV          PZR.CI          PZR.AV          PZR.BI          PZR.CV          ANA1            ANA2            ANA3            DIG.stat1_01    DIG.stat1_02    DIG.stat1_03    DIG.stat1_04    DIG.stat1_05    DIG.stat1_06    DIG.stat1_07    DIG.stat1_08    DIG.stat1_09    DIG.stat1_10    DIG.stat1_11    DIG.stat1_12    DIG.stat1_13    DIG.stat1_14    DIG.stat1_15    DIG.stat1_16    \u0001\u0000\u0000\u0000\u0000\u0000\u0000\u0000\u0001\u0000\u0000\u0000\u0000\u0000\u0000\u0000\u0001\u0000\u0000\u0000\u0000\u0000\u0000\u0000\u0000\u0000\u0000\u0000\u0000\u0000\u0000\u0000\u0000\u0000\u0000\u0000ÿÿ\u0000\u0000\u0000\u0000\u0000\u0000", "PMU.107\u0000\u0000\u0000\u0000\u0000\u0000\u0000\u0000\u0000\u0000k\u0000\u000f\u0000\u0006\u0000\u0003\u0000\u0001PZR.AI          PZR.BV          PZR.CI          PZR.AV          PZR.BI          PZR.CV          ANA1            ANA2            ANA3            DIG.stat1_01    DIG.stat1_02    DIG.stat1_03    DIG.stat1_04    DIG.stat1_05    DIG.stat1_06    DIG.stat1_07    DIG.stat1_08    DIG.stat1_09    DIG.stat1_10    DIG.stat1_11    DIG.stat1_12    DIG.stat1_13    DIG.stat1_14    DIG.stat1_15    DIG.stat1_16    \u0001\u0000\u0000\u0000\u0000\u0000\u0000\u0000\u0001\u0000\u0000\u0000\u0000\u0000\u0000\u0000\u0001\u0000\u0000\u0000\u0000\u0000\u0000\u0000\u0000\u0000\u0000\u0000\u0000\u0000\u0000\u0000\u0000\u0000\u0000\u0000ÿÿ\u0000\u0000\u0000\u0000\u0000\u0000", "PMU.108\u0000\u0000\u0000\u0000\u0000\u0000\u0000\u0000\u0000\u0000l\u0000\u000f\u0000\u0006\u0000\u0003\u0000\u0001PZR.AI          PZR.BV          PZR.CI          PZR.AV          PZR.BI          PZR.CV          ANA1            ANA2            ANA3            DIG.stat1_01    DIG.stat1_02    DIG.stat1_03    DIG.stat1_04    DIG.stat1_05    DIG.stat1_06    DIG.stat1_07    DIG.stat1_08    DIG.stat1_09    DIG.stat1_10    DIG.stat1_11    DIG.stat1_12    DIG.stat1_13    DIG.stat1_14    DIG.stat1_15    DIG.stat1_16    \u0001\u0000\u0000\u0000\u0000\u0000\u0000\u0000\u0001\u0000\u0000\u0000\u0000\u0000\u0000\u0000\u0001\u0000\u0000\u0000\u0000\u0000\u0000\u0000\u0000\u0000\u0000\u0000\u0000\u0000\u0000\u0000\u0000\u0000\u0000\u0000ÿÿ\u0000\u0000\u0000\u0000\u0000\u0000", "PMU.109\u0000\u0000\u0000\u0000\u0000\u0000\u0000\u0000\u0000\u0000m\u0000\u000f\u0000\u0006\u0000\u0003\u0000\u0001PZR.AI          PZR.BV          PZR.CI          PZR.AV          PZR.BI          PZR.CV          ANA1            ANA2            ANA3            DIG.stat1_01    DIG.stat1_02    DIG.stat1_03    DIG.stat1_04    DIG.stat1_05    DIG.stat1_06    DIG.stat1_07    DIG.stat1_08    DIG.stat1_09    DIG.stat1_10    DIG.stat1_11    DIG.stat1_12    DIG.stat1_13    DIG.stat1_14    DIG.stat1_15    DIG.stat1_16    \u0001\u0000\u0000\u0000\u0000\u0000\u0000\u0000\u0001\u0000\u0000\u0000\u0000\u0000\u0000\u0000\u0001\u0000\u0000\u0000\u0000\u0000\u0000\u0000\u0000\u0000\u0000\u0000\u0000\u0000\u0000\u0000\u0000\u0000\u0000\u0000ÿÿ\u0000\u0000\u0000\u0000\u0000\u0000", "PMU.110\u0000\u0000\u0000\u0000\u0000\u0000\u0000\u0000\u0000\u0000n\u0000\u000f\u0000\u0006\u0000\u0003\u0000\u0001PZR.AI          PZR.BV          PZR.CI          PZR.AV          PZR.BI          PZR.CV          ANA1            ANA2            ANA3            DIG.stat1_01    DIG.stat1_02    DIG.stat1_03    DIG.stat1_04    DIG.stat1_05    DIG.stat1_06    DIG.stat1_07    DIG.stat1_08    DIG.stat1_09    DIG.stat1_10    DIG.stat1_11    DIG.stat1_12    DIG.stat1_13    DIG.stat1_14    DIG.stat1_15    DIG.stat1_16    \u0001\u0000\u0000\u0000\u0000\u0000\u0000\u0000\u0001\u0000\u0000\u0000\u0000\u0000\u0000\u0000\u0001\u0000\u0000\u0000\u0000\u0000\u0000\u0000\u0000\u0000\u0000\u0000\u0000\u0000\u0000\u0000\u0000\u0000\u0000\u0000ÿÿ\u0000\u0000\u0000\u0000\u0000\u0000", "PMU.111\u0000\u0000\u0000\u0000\u0000\u0000\u0000\u0000\u0000\u0000o\u0000\u000f\u0000\u0006\u0000\u0003\u0000\u0001PZR.AI          PZR.BV          PZR.CI          PZR.AV          PZR.BI          PZR.CV          ANA1            ANA2            ANA3            DIG.stat1_01    DIG.stat1_02    DIG.stat1_03    DIG.stat1_04    DIG.stat1_05    DIG.stat1_06    DIG.stat1_07    DIG.stat1_08    DIG.stat1_09    DIG.stat1_10    DIG.stat1_11    DIG.stat1_12    DIG.stat1_13    DIG.stat1_14    DIG.stat1_15    DIG.stat1_16    \u0001\u0000\u0000\u0000\u0000\u0000\u0000\u0000\u0001\u0000\u0000\u0000\u0000\u0000\u0000\u0000\u0001\u0000\u0000\u0000\u0000\u0000\u0000\u0000\u0000\u0000\u0000\u0000\u0000\u0000\u0000\u0000\u0000\u0000\u0000\u0000ÿÿ\u0000\u0000\u0000\u0000\u0000\u0000", "PMU.112\u0000\u0000\u0000\u0000\u0000\u0000\u0000\u0000\u0000\u0000p\u0000\u000f\u0000\u0006\u0000\u0003\u0000\u0001PZR.AI          PZR.BV          PZR.CI          PZR.AV          PZR.BI          PZR.CV          ANA1            ANA2            ANA3            DIG.stat1_01    DIG.stat1_02    DIG.stat1_03    DIG.stat1_04    DIG.stat1_05    DIG.stat1_06    DIG.stat1_07    DIG.stat1_08    DIG.stat1_09    DIG.stat1_10    DIG.stat1_11    DIG.stat1_12    DIG.stat1_13    DIG.stat1_14    DIG.stat1_15    DIG.stat1_16    \u0001\u0000\u0000\u0000\u0000\u0000\u0000\u0000\u0001\u0000\u0000\u0000\u0000\u0000\u0000\u0000\u0001\u0000\u0000\u0000\u0000\u0000\u0000\u0000\u0000\u0000\u0000\u0000\u0000\u0000\u0000\u0000\u0000\u0000\u0000\u0000ÿÿ\u0000\u0000\u0000\u0000\u0000\u0000", "PMU.113\u0000\u0000\u0000\u0000\u0000\u0000\u0000\u0000\u0000\u0000q\u0000\u000f\u0000\u0006\u0000\u0003\u0000\u0001PZR.AI          PZR.BV          PZR.CI          PZR.AV          PZR.BI          PZR.CV          ANA1            ANA2            ANA3            DIG.stat1_01    DIG.stat1_02    DIG.stat1_03    DIG.stat1_04    DIG.stat1_05    DIG.stat1_06    DIG.stat1_07    DIG.stat1_08    DIG.stat1_09    DIG.stat1_10    DIG.stat1_11    DIG.stat1_12    DIG.stat1_13    DIG.stat1_14    DIG.stat1_15    DIG.stat1_16    \u0001\u0000\u0000\u0000\u0000\u0000\u0000\u0000\u0001\u0000\u0000\u0000\u0000\u0000\u0000\u0000\u0001\u0000\u0000\u0000\u0000\u0000\u0000\u0000\u0000\u0000\u0000\u0000\u0000\u0000\u0000\u0000\u0000\u0000\u0000\u0000ÿÿ\u0000\u0000\u0000\u0000\u0000\u0000", "PMU.114\u0000\u0000\u0000\u0000\u0000\u0000\u0000\u0000\u0000\u0000r\u0000\u000f\u0000\u0006\u0000\u0003\u0000\u0001PZR.AI          PZR.BV          PZR.CI          PZR.AV          PZR.BI          PZR.CV          ANA1            ANA2            ANA3            DIG.stat1_01    DIG.stat1_02    DIG.stat1_03    DIG.stat1_04    DIG.stat1_05    DIG.stat1_06    DIG.stat1_07    DIG.stat1_08    DIG.stat1_09    DIG.stat1_10    DIG.stat1_11    DIG.stat1_12    DIG.stat1_13    DIG.stat1_14    DIG.stat1_15    DIG.stat1_16    \u0001\u0000\u0000\u0000\u0000\u0000\u0000\u0000\u0001\u0000\u0000\u0000\u0000\u0000\u0000\u0000\u0001\u0000\u0000\u0000\u0000\u0000\u0000\u0000\u0000\u0000\u0000\u0000\u0000\u0000\u0000\u0000\u0000\u0000\u0000\u0000ÿÿ\u0000\u0000\u0000\u0000\u0000\u0000", "PMU.115\u0000\u0000\u0000\u0000\u0000\u0000\u0000\u0000\u0000\u0000s\u0000\u000f\u0000\u0006\u0000\u0003\u0000\u0001PZR.AI          PZR.BV          PZR.CI          PZR.AV          PZR.BI          PZR.CV          ANA1            ANA2            ANA3            DIG.stat1_01    DIG.stat1_02    DIG.stat1_03    DIG.stat1_04    DIG.stat1_05    DIG.stat1_06    DIG.stat1_07    DIG.stat1_08    DIG.stat1_09    DIG.stat1_10    DIG.stat1_11    DIG.stat1_12    DIG.stat1_13    DIG.stat1_14    DIG.stat1_15    DIG.stat1_16    \u0001\u0000\u0000\u0000\u0000\u0000\u0000\u0000\u0001\u0000\u0000\u0000\u0000\u0000\u0000\u0000\u0001\u0000\u0000\u0000\u0000\u0000\u0000\u0000\u0000\u0000\u0000\u0000\u0000\u0000\u0000\u0000\u0000\u0000\u0000\u0000ÿÿ\u0000\u0000\u0000\u0000\u0000\u0000", "PMU.116\u0000\u0000\u0000\u0000\u0000\u0000\u0000\u0000\u0000\u0000t\u0000\u000f\u0000\u0006\u0000\u0003\u0000\u0001PZR.AI          PZR.BV          PZR.CI          PZR.AV          PZR.BI          PZR.CV          ANA1            ANA2            ANA3            DIG.stat1_01    DIG.stat1_02    DIG.stat1_03    DIG.stat1_04    DIG.stat1_05    DIG.stat1_06    DIG.stat1_07    DIG.stat1_08    DIG.stat1_09    DIG.stat1_10    DIG.stat1_11    DIG.stat1_12    DIG.stat1_13    DIG.stat1_14    DIG.stat1_15    DIG.stat1_16    \u0001\u0000\u0000\u0000\u0000\u0000\u0000\u0000\u0001\u0000\u0000\u0000\u0000\u0000\u0000\u0000\u0001\u0000\u0000\u0000\u0000\u0000\u0000\u0000\u0000\u0000\u0000\u0000\u0000\u0000\u0000\u0000\u0000\u0000\u0000\u0000ÿÿ\u0000\u0000\u0000\u0000\u0000\u0000", "PMU.117\u0000\u0000\u0000\u0000\u0000\u0000\u0000\u0000\u0000\u0000u\u0000\u000f\u0000\u0006\u0000\u0003\u0000\u0001PZR.AI          PZR.BV          PZR.CI          PZR.AV          PZR.BI          PZR.CV          ANA1            ANA2            ANA3            DIG.stat1_01    DIG.stat1_02    DIG.stat1_03    DIG.stat1_04    DIG.stat1_05    DIG.stat1_06    DIG.stat1_07    DIG.stat1_08    DIG.stat1_09    DIG.stat1_10    DIG.stat1_11    DIG.stat1_12    DIG.stat1_13    DIG.stat1_14    DIG.stat1_15    DIG.stat1_16    \u0001\u0000\u0000\u0000\u0000\u0000\u0000\u0000\u0001\u0000\u0000\u0000\u0000\u0000\u0000\u0000\u0001\u0000\u0000\u0000\u0000\u0000\u0000\u0000\u0000\u0000\u0000\u0000\u0000\u0000\u0000\u0000\u0000\u0000\u0000\u0000ÿÿ\u0000\u0000\u0000\u0000\u0000\u0000", "PMU.118\u0000\u0000\u0000\u0000\u0000\u0000\u0000\u0000\u0000\u0000v\u0000\u000f\u0000\u0006\u0000\u0003\u0000\u0001PZR.AI          PZR.BV          PZR.CI          PZR.AV          PZR.BI          PZR.CV          ANA1            ANA2            ANA3            DIG.stat1_01    DIG.stat1_02    DIG.stat1_03    DIG.stat1_04    DIG.stat1_05    DIG.stat1_06    DIG.stat1_07    DIG.stat1_08    DIG.stat1_09    DIG.stat1_10    DIG.stat1_11    DIG.stat1_12    DIG.stat1_13    DIG.stat1_14    DIG.stat1_15    DIG.stat1_16    \u0001\u0000\u0000\u0000\u0000\u0000\u0000\u0000\u0001\u0000\u0000\u0000\u0000\u0000\u0000\u0000\u0001\u0000\u0000\u0000\u0000\u0000\u0000\u0000\u0000\u0000\u0000\u0000\u0000\u0000\u0000\u0000\u0000\u0000\u0000\u0000ÿÿ\u0000\u0000\u0000\u0000\u0000\u0000", "PMU.119\u0000\u0000\u0000\u0000\u0000\u0000\u0000\u0000\u0000\u0000w\u0000\u000f\u0000\u0006\u0000\u0003\u0000\u0001PZR.AI          PZR.BV          PZR.CI          PZR.AV          PZR.BI          PZR.CV          ANA1            ANA2            ANA3            DIG.stat1_01    DIG.stat1_02    DIG.stat1_03    DIG.stat1_04    DIG.stat1_05    DIG.stat1_06    DIG.stat1_07    DIG.stat1_08    DIG.stat1_09    DIG.stat1_10    DIG.stat1_11    DIG.stat1_12    DIG.stat1_13    DIG.stat1_14    DIG.stat1_15    DIG.stat1_16    \u0001\u0000\u0000\u0000\u0000\u0000\u0000\u0000\u0001\u0000\u0000\u0000\u0000\u0000\u0000\u0000\u0001\u0000\u0000\u0000\u0000\u0000\u0000\u0000\u0000\u0000\u0000\u0000\u0000\u0000\u0000\u0000\u0000\u0000\u0000\u0000ÿÿ\u0000\u0000\u0000\u0000\u0000\u0000", "PMU.120\u0000\u0000\u0000\u0000\u0000\u0000\u0000\u0000\u0000\u0000x\u0000\u000f\u0000\u0006\u0000\u0003\u0000\u0001PZR.AI          PZR.BV          PZR.CI          PZR.AV          PZR.BI          PZR.CV          ANA1            ANA2            ANA3            DIG.stat1_01    DIG.stat1_02    DIG.stat1_03    DIG.stat1_04    DIG.stat1_05    DIG.stat1_06    DIG.stat1_07    DIG.stat1_08    DIG.stat1_09    DIG.stat1_10    DIG.stat1_11    DIG.stat1_12    DIG.stat1_13    DIG.stat1_14    DIG.stat1_15    DIG.stat1_16    \u0001\u0000\u0000\u0000\u0000\u0000\u0000\u0000\u0001\u0000\u0000\u0000\u0000\u0000\u0000\u0000\u0001\u0000\u0000\u0000\u0000\u0000\u0000\u0000\u0000\u0000\u0000\u0000\u0000\u0000\u0000\u0000\u0000\u0000\u0000\u0000ÿÿ\u0000\u0000\u0000\u0000\u0000\u0000", "PMU.121\u0000\u0000\u0000\u0000\u0000\u0000\u0000\u0000\u0000\u0000y\u0000\u000f\u0000\u0006\u0000\u0003\u0000\u0001PZR.AI          PZR.BV          PZR.CI          PZR.AV          PZR.BI          PZR.CV          ANA1            ANA2            ANA3            DIG.stat1_01    DIG.stat1_02    DIG.stat1_03    DIG.stat1_04    DIG.stat1_05    DIG.stat1_06    DIG.stat1_07    DIG.stat1_08    DIG.stat1_09    DIG.stat1_10    DIG.stat1_11    DIG.stat1_12    DIG.stat1_13    DIG.stat1_14    DIG.stat1_15    DIG.stat1_16    \u0001\u0000\u0000\u0000\u0000\u0000\u0000\u0000\u0001\u0000\u0000\u0000\u0000\u0000\u0000\u0000\u0001\u0000\u0000\u0000\u0000\u0000\u0000\u0000\u0000\u0000\u0000\u0000\u0000\u0000\u0000\u0000\u0000\u0000\u0000\u0000ÿÿ\u0000\u0000\u0000\u0000\u0000\u0000", "PMU.122\u0000\u0000\u0000\u0000\u0000\u0000\u0000\u0000\u0000\u0000z\u0000\u000f\u0000\u0006\u0000\u0003\u0000\u0001PZR.AI          PZR.BV          PZR.CI          PZR.AV          PZR.BI          PZR.CV          ANA1            ANA2            ANA3            DIG.stat1_01    DIG.stat1_02    DIG.stat1_03    DIG.stat1_04    DIG.stat1_05    DIG.stat1_06    DIG.stat1_07    DIG.stat1_08    DIG.stat1_09    DIG.stat1_10    DIG.stat1_11    DIG.stat1_12    DIG.stat1_13    DIG.stat1_14    DIG.stat1_15    DIG.stat1_16    \u0001\u0000\u0000\u0000\u0000\u0000\u0000\u0000\u0001\u0000\u0000\u0000\u0000\u0000\u0000\u0000\u0001\u0000\u0000\u0000\u0000\u0000\u0000\u0000\u0000\u0000\u0000\u0000\u0000\u0000\u0000\u0000\u0000\u0000\u0000\u0000ÿÿ\u0000\u0000\u0000\u0000\u0000\u0000", "PMU.123\u0000\u0000\u0000\u0000\u0000\u0000\u0000\u0000\u0000\u0000{\u0000\u000f\u0000\u0006\u0000\u0003\u0000\u0001PZR.AI          PZR.BV          PZR.CI          PZR.AV          PZR.BI          PZR.CV          ANA1            ANA2            ANA3            DIG.stat1_01    DIG.stat1_02    DIG.stat1_03    DIG.stat1_04    DIG.stat1_05    DIG.stat1_06    DIG.stat1_07    DIG.stat1_08    DIG.stat1_09    DIG.stat1_10    DIG.stat1_11    DIG.stat1_12    DIG.stat1_13    DIG.stat1_14    DIG.stat1_15    DIG.stat1_16    \u0001\u0000\u0000\u0000\u0000\u0000\u0000\u0000\u0001\u0000\u0000\u0000\u0000\u0000\u0000\u0000\u0001\u0000\u0000\u0000\u0000\u0000\u0000\u0000\u0000\u0000\u0000\u0000\u0000\u0000\u0000\u0000\u0000\u0000\u0000\u0000ÿÿ\u0000\u0000\u0000\u0000\u0000\u0000", "PMU.124\u0000\u0000\u0000\u0000\u0000\u0000\u0000\u0000\u0000\u0000|\u0000\u000f\u0000\u0006\u0000\u0003\u0000\u0001PZR.AI          PZR.BV          PZR.CI          PZR.AV          PZR.BI          PZR.CV          ANA1            ANA2            ANA3            DIG.stat1_01    DIG.stat1_02    DIG.stat1_03    DIG.stat1_04    DIG.stat1_05    DIG.stat1_06    DIG.stat1_07    DIG.stat1_08    DIG.stat1_09    DIG.stat1_10    DIG.stat1_11    DIG.stat1_12    DIG.stat1_13    DIG.stat1_14    DIG.stat1_15    DIG.stat1_16    \u0001\u0000\u0000\u0000\u0000\u0000\u0000\u0000\u0001\u0000\u0000\u0000\u0000\u0000\u0000\u0000\u0001\u0000\u0000\u0000\u0000\u0000\u0000\u0000\u0000\u0000\u0000\u0000\u0000\u0000\u0000\u0000\u0000\u0000\u0000\u0000ÿÿ\u0000\u0000\u0000\u0000\u0000\u0000", "PMU.125\u0000\u0000\u0000\u0000\u0000\u0000\u0000\u0000\u0000\u0000}\u0000\u000f\u0000\u0006\u0000\u0003\u0000\u0001PZR.AI          PZR.BV          PZR.CI          PZR.AV          PZR.BI          PZR.CV          ANA1            ANA2            ANA3            DIG.stat1_01    DIG.stat1_02    DIG.stat1_03    DIG.stat1_04    DIG.stat1_05    DIG.stat1_06    DIG.stat1_07    DIG.stat1_08    DIG.stat1_09    DIG.stat1_10    DIG.stat1_11    DIG.stat1_12    DIG.stat1_13    DIG.stat1_14    DIG.stat1_15    DIG.stat1_16    \u0001\u0000\u0000\u0000\u0000\u0000\u0000\u0000\u0001\u0000\u0000\u0000\u0000\u0000\u0000\u0000\u0001\u0000\u0000\u0000\u0000\u0000\u0000\u0000\u0000\u0000\u0000\u0000\u0000\u0000\u0000\u0000\u0000\u0000\u0000\u0000ÿÿ\u0000\u0000\u0000\u0000\u0000\u0000", "PMU.126\u0000\u0000\u0000\u0000\u0000\u0000\u0000\u0000\u0000\u0000~\u0000\u000f\u0000\u0006\u0000\u0003\u0000\u0001PZR.AI          PZR.BV          PZR.CI          PZR.AV          PZR.BI          PZR.CV          ANA1            ANA2            ANA3            DIG.stat1_01    DIG.stat1_02    DIG.stat1_03    DIG.stat1_04    DIG.stat1_05    DIG.stat1_06    DIG.stat1_07    DIG.stat1_08    DIG.stat1_09    DIG.stat1_10    DIG.stat1_11    DIG.stat1_12    DIG.stat1_13    DIG.stat1_14    DIG.stat1_15    DIG.stat1_16    \u0001\u0000\u0000\u0000\u0000\u0000\u0000\u0000\u0001\u0000\u0000\u0000\u0000\u0000\u0000\u0000\u0001\u0000\u0000\u0000\u0000\u0000\u0000\u0000\u0000\u0000\u0000\u0000\u0000\u0000\u0000\u0000\u0000\u0000\u0000\u0000ÿÿ\u0000\u0000\u0000\u0000\u0000\u0000", "PMU.127\u0000\u0000\u0000\u0000\u0000\u0000\u0000\u0000\u0000\u0000\u0000\u000f\u0000\u0006\u0000\u0003\u0000\u0001PZR.AI          PZR.BV          PZR.CI          PZR.AV          PZR.BI          PZR.CV          ANA1            ANA2            ANA3            DIG.stat1_01    DIG.stat1_02    DIG.stat1_03    DIG.stat1_04    DIG.stat1_05    DIG.stat1_06    DIG.stat1_07    DIG.stat1_08    DIG.stat1_09    DIG.stat1_10    DIG.stat1_11    DIG.stat1_12    DIG.stat1_13    DIG.stat1_14    DIG.stat1_15    DIG.stat1_16    \u0001\u0000\u0000\u0000\u0000\u0000\u0000\u0000\u0001\u0000\u0000\u0000\u0000\u0000\u0000\u0000\u0001\u0000\u0000\u0000\u0000\u0000\u0000\u0000\u0000\u0000\u0000\u0000\u0000\u0000\u0000\u0000\u0000\u0000\u0000\u0000ÿÿ\u0000\u0000\u0000\u0000\u0000\u0000", "PMU.128\u0000\u0000\u0000\u0000\u0000\u0000\u0000\u0000\u0000\u0000€\u0000\u000f\u0000\u0006\u0000\u0003\u0000\u0001PZR.AI          PZR.BV          PZR.CI          PZR.AV          PZR.BI          PZR.CV          ANA1            ANA2            ANA3            DIG.stat1_01    DIG.stat1_02    DIG.stat1_03    DIG.stat1_04    DIG.stat1_05    DIG.stat1_06    DIG.stat1_07    DIG.stat1_08    DIG.stat1_09    DIG.stat1_10    DIG.stat1_11    DIG.stat1_12    DIG.stat1_13    DIG.stat1_14    DIG.stat1_15    DIG.stat1_16    \u0001\u0000\u0000\u0000\u0000\u0000\u0000\u0000\u0001\u0000\u0000\u0000\u0000\u0000\u0000\u0000\u0001\u0000\u0000\u0000\u0000\u0000\u0000\u0000\u0000\u0000\u0000\u0000\u0000\u0000\u0000\u0000\u0000\u0000\u0000\u0000ÿÿ\u0000\u0000\u0000\u0000\u0000\u0000", "PMU.129\u0000\u0000\u0000\u0000\u0000\u0000\u0000\u0000\u0000\u0000\u0000\u000f\u0000\u0006\u0000\u0003\u0000\u0001PZR.AI          PZR.BV          PZR.CI          PZR.AV          PZR.BI          PZR.CV          ANA1            ANA2            ANA3            DIG.stat1_01    DIG.stat1_02    DIG.stat1_03    DIG.stat1_04    DIG.stat1_05    DIG.stat1_06    DIG.stat1_07    DIG.stat1_08    DIG.stat1_09    DIG.stat1_10    DIG.stat1_11    DIG.stat1_12    DIG.stat1_13    DIG.stat1_14    DIG.stat1_15    DIG.stat1_16    \u0001\u0000\u0000\u0000\u0000\u0000\u0000\u0000\u0001\u0000\u0000\u0000\u0000\u0000\u0000\u0000\u0001\u0000\u0000\u0000\u0000\u0000\u0000\u0000\u0000\u0000\u0000\u0000\u0000\u0000\u0000\u0000\u0000\u0000\u0000\u0000ÿÿ\u0000\u0000\u0000\u0000\u0000\u0000", "PMU.130\u0000\u0000\u0000\u0000\u0000\u0000\u0000\u0000\u0000\u0000‚\u0000\u000f\u0000\u0006\u0000\u0003\u0000\u0001PZR.AI          PZR.BV          PZR.CI          PZR.AV          PZR.BI          PZR.CV          ANA1            ANA2            ANA3            DIG.stat1_01    DIG.stat1_02    DIG.stat1_03    DIG.stat1_04    DIG.stat1_05    DIG.stat1_06    DIG.stat1_07    DIG.stat1_08    DIG.stat1_09    DIG.stat1_10    DIG.stat1_11    DIG.stat1_12    DIG.stat1_13    DIG.stat1_14    DIG.stat1_15    DIG.stat1_16    \u0001\u0000\u0000\u0000\u0000\u0000\u0000\u0000\u0001\u0000\u0000\u0000\u0000\u0000\u0000\u0000\u0001\u0000\u0000\u0000\u0000\u0000\u0000\u0000\u0000\u0000\u0000\u0000\u0000\u0000\u0000\u0000\u0000\u0000\u0000\u0000ÿÿ\u0000\u0000\u0000\u0000\u0000\u0000", "PMU.131\u0000\u0000\u0000\u0000\u0000\u0000\u0000\u0000\u0000\u0000ƒ\u0000\u000f\u0000\u0006\u0000\u0003\u0000\u0001PZR.AI          PZR.BV          PZR.CI          PZR.AV          PZR.BI          PZR.CV          ANA1            ANA2            ANA3            DIG.stat1_01    DIG.stat1_02    DIG.stat1_03    DIG.stat1_04    DIG.stat1_05    DIG.stat1_06    DIG.stat1_07    DIG.stat1_08    DIG.stat1_09    DIG.stat1_10    DIG.stat1_11    DIG.stat1_12    DIG.stat1_13    DIG.stat1_14    DIG.stat1_15    DIG.stat1_16    \u0001\u0000\u0000\u0000\u0000\u0000\u0000\u0000\u0001\u0000\u0000\u0000\u0000\u0000\u0000\u0000\u0001\u0000\u0000\u0000\u0000\u0000\u0000\u0000\u0000\u0000\u0000\u0000\u0000\u0000\u0000\u0000\u0000\u0000\u0000\u0000ÿÿ\u0000\u0000\u0000\u0000\u0000\u0000", "PMU.132\u0000\u0000\u0000\u0000\u0000\u0000\u0000\u0000\u0000\u0000„\u0000\u000f\u0000\u0006\u0000\u0003\u0000\u0001PZR.AI          PZR.BV          PZR.CI          PZR.AV          PZR.BI          PZR.CV          ANA1            ANA2            ANA3            DIG.stat1_01    DIG.stat1_02    DIG.stat1_03    DIG.stat1_04    DIG.stat1_05    DIG.stat1_06    DIG.stat1_07    DIG.stat1_08    DIG.stat1_09    DIG.stat1_10    DIG.stat1_11    DIG.stat1_12    DIG.stat1_13    DIG.stat1_14    DIG.stat1_15    DIG.stat1_16    \u0001\u0000\u0000\u0000\u0000\u0000\u0000\u0000\u0001\u0000\u0000\u0000\u0000\u0000\u0000\u0000\u0001\u0000\u0000\u0000\u0000\u0000\u0000\u0000\u0000\u0000\u0000\u0000\u0000\u0000\u0000\u0000\u0000\u0000\u0000\u0000ÿÿ\u0000\u0000\u0000\u0000\u0000\u0000", "PMU.133\u0000\u0000\u0000\u0000\u0000\u0000\u0000\u0000\u0000\u0000…\u0000\u000f\u0000\u0006\u0000\u0003\u0000\u0001PZR.AI          PZR.BV          PZR.CI          PZR.AV          PZR.BI          PZR.CV          ANA1            ANA2            ANA3            DIG.stat1_01    DIG.stat1_02    DIG.stat1_03    DIG.stat1_04    DIG.stat1_05    DIG.stat1_06    DIG.stat1_07    DIG.stat1_08    DIG.stat1_09    DIG.stat1_10    DIG.stat1_11    DIG.stat1_12    DIG.stat1_13    DIG.stat1_14    DIG.stat1_15    DIG.stat1_16    \u0001\u0000\u0000\u0000\u0000\u0000\u0000\u0000\u0001\u0000\u0000\u0000\u0000\u0000\u0000\u0000\u0001\u0000\u0000\u0000\u0000\u0000\u0000\u0000\u0000\u0000\u0000\u0000\u0000\u0000\u0000\u0000\u0000\u0000\u0000\u0000ÿÿ\u0000\u0000\u0000\u0000\u0000\u0000", "PMU.134\u0000\u0000\u0000\u0000\u0000\u0000\u0000\u0000\u0000\u0000†\u0000\u000f\u0000\u0006\u0000\u0003\u0000\u0001PZR.AI          PZR.BV          PZR.CI          PZR.AV          PZR.BI          PZR.CV          ANA1            ANA2            ANA3            DIG.stat1_01    DIG.stat1_02    DIG.stat1_03    DIG.stat1_04    DIG.stat1_05    DIG.stat1_06    DIG.stat1_07    DIG.stat1_08    DIG.stat1_09    DIG.stat1_10    DIG.stat1_11    DIG.stat1_12    DIG.stat1_13    DIG.stat1_14    DIG.stat1_15    DIG.stat1_16    \u0001\u0000\u0000\u0000\u0000\u0000\u0000\u0000\u0001\u0000\u0000\u0000\u0000\u0000\u0000\u0000\u0001\u0000\u0000\u0000\u0000\u0000\u0000\u0000\u0000\u0000\u0000\u0000\u0000\u0000\u0000\u0000\u0000\u0000\u0000\u0000ÿÿ\u0000\u0000\u0000\u0000\u0000\u0000", "PMU.135\u0000\u0000\u0000\u0000\u0000\u0000\u0000\u0000\u0000\u0000‡\u0000\u000f\u0000\u0006\u0000\u0003\u0000\u0001PZR.AI          PZR.BV          PZR.CI          PZR.AV          PZR.BI          PZR.CV          ANA1            ANA2            ANA3            DIG.stat1_01    DIG.stat1_02    DIG.stat1_03    DIG.stat1_04    DIG.stat1_05    DIG.stat1_06    DIG.stat1_07    DIG.stat1_08    DIG.stat1_09    DIG.stat1_10    DIG.stat1_11    DIG.stat1_12    DIG.stat1_13    DIG.stat1_14    DIG.stat1_15    DIG.stat1_16    \u0001\u0000\u0000\u0000\u0000\u0000\u0000\u0000\u0001\u0000\u0000\u0000\u0000\u0000\u0000\u0000\u0001\u0000\u0000\u0000\u0000\u0000\u0000\u0000\u0000\u0000\u0000\u0000\u0000\u0000\u0000\u0000\u0000\u0000\u0000\u0000ÿÿ\u0000\u0000\u0000\u0000\u0000\u0000", "PMU.136\u0000\u0000\u0000\u0000\u0000\u0000\u0000\u0000\u0000\u0000ˆ\u0000\u000f\u0000\u0006\u0000\u0003\u0000\u0001PZR.AI          PZR.BV          PZR.CI          PZR.AV          PZR.BI          PZR.CV          ANA1            ANA2            ANA3            DIG.stat1_01    DIG.stat1_02    DIG.stat1_03    DIG.stat1_04    DIG.stat1_05    DIG.stat1_06    DIG.stat1_07    DIG.stat1_08    DIG.stat1_09    DIG.stat1_10    DIG.stat1_11    DIG.stat1_12    DIG.stat1_13    DIG.stat1_14    DIG.stat1_15    DIG.stat1_16    \u0001\u0000\u0000\u0000\u0000\u0000\u0000\u0000\u0001\u0000\u0000\u0000\u0000\u0000\u0000\u0000\u0001\u0000\u0000\u0000\u0000\u0000\u0000\u0000\u0000\u0000\u0000\u0000\u0000\u0000\u0000\u0000\u0000\u0000\u0000\u0000ÿÿ\u0000\u0000\u0000\u0000\u0000\u0000", "PMU.137\u0000\u0000\u0000\u0000\u0000\u0000\u0000\u0000\u0000\u0000‰\u0000\u000f\u0000\u0006\u0000\u0003\u0000\u0001PZR.AI          PZR.BV          PZR.CI          PZR.AV          PZR.BI          PZR.CV          ANA1            ANA2            ANA3            DIG.stat1_01    DIG.stat1_02    DIG.stat1_03    DIG.stat1_04    DIG.stat1_05    DIG.stat1_06    DIG.stat1_07    DIG.stat1_08    DIG.stat1_09    DIG.stat1_10    DIG.stat1_11    DIG.stat1_12    DIG.stat1_13    DIG.stat1_14    DIG.stat1_15    DIG.stat1_16    \u0001\u0000\u0000\u0000\u0000\u0000\u0000\u0000\u0001\u0000\u0000\u0000\u0000\u0000\u0000\u0000\u0001\u0000\u0000\u0000\u0000\u0000\u0000\u0000\u0000\u0000\u0000\u0000\u0000\u0000\u0000\u0000\u0000\u0000\u0000\u0000ÿÿ\u0000\u0000\u0000\u0000\u0000\u0000", "PMU.138\u0000\u0000\u0000\u0000\u0000\u0000\u0000\u0000\u0000\u0000Š\u0000\u000f\u0000\u0006\u0000\u0003\u0000\u0001PZR.AI          PZR.BV          PZR.CI          PZR.AV          PZR.BI          PZR.CV          ANA1            ANA2            ANA3            DIG.stat1_01    DIG.stat1_02    DIG.stat1_03    DIG.stat1_04    DIG.stat1_05    DIG.stat1_06    DIG.stat1_07    DIG.stat1_08    DIG.stat1_09    DIG.stat1_10    DIG.stat1_11    DIG.stat1_12    DIG.stat1_13    DIG.stat1_14    DIG.stat1_15    DIG.stat1_16    \u0001\u0000\u0000\u0000\u0000\u0000\u0000\u0000\u0001\u0000\u0000\u0000\u0000\u0000\u0000\u0000\u0001\u0000\u0000\u0000\u0000\u0000\u0000\u0000\u0000\u0000\u0000\u0000\u0000\u0000\u0000\u0000\u0000\u0000\u0000\u0000ÿÿ\u0000\u0000\u0000\u0000\u0000\u0000", "PMU.139\u0000\u0000\u0000\u0000\u0000\u0000\u0000\u0000\u0000\u0000‹\u0000\u000f\u0000\u0006\u0000\u0003\u0000\u0001PZR.AI          PZR.BV          PZR.CI          PZR.AV          PZR.BI          PZR.CV          ANA1            ANA2            ANA3            DIG.stat1_01    DIG.stat1_02    DIG.stat1_03    DIG.stat1_04    DIG.stat1_05    DIG.stat1_06    DIG.stat1_07    DIG.stat1_08    DIG.stat1_09    DIG.stat1_10    DIG.stat1_11    DIG.stat1_12    DIG.stat1_13    DIG.stat1_14    DIG.stat1_15    DIG.stat1_16    \u0001\u0000\u0000\u0000\u0000\u0000\u0000\u0000\u0001\u0000\u0000\u0000\u0000\u0000\u0000\u0000\u0001\u0000\u0000\u0000\u0000\u0000\u0000\u0000\u0000\u0000\u0000\u0000\u0000\u0000\u0000\u0000\u0000\u0000\u0000\u0000ÿÿ\u0000\u0000\u0000\u0000\u0000\u0000"]}) -> (queue out=w19:refnum<queue>, error out=w18:errorcluster)  [unwired: 3 in, 1 out]
  n99 = Obtain Queue(name (unnamed)="UDP Communication", element data type="" ("string")) -> (queue out=w2:refnum<queue>, error out=w1:errorcluster)  [unwired: 3 in, 1 out]
  n100 = while {
    tunnel: [w264] -> w12
    tunnel: [w263] -> w11
    tunnel: w7 -> [w262]
    tunnel: w9 -> [w261]
    tunnel: w10 -> [w259]
    tunnel: w8 -> [w258]
    tunnel: w2 -> [w256]
    tunnel: w1 -> [w255]
    stop <- w266 stop-if-true
    # "UDP Loop"
    n101 = Dequeue Element(queue=w256, error in (no error)=w255) -> (element=w254:string)  [unwired: 1 in, 3 out]
    "UDP STRNG" <- w254
    n102 = case shown="True" "Display Cluster Output" {
      tunnel: [_ w270] -> w253
      tunnel: w254 -> [_ w270]
      tunnel: [_ w269] -> w260
      tunnel: w254 -> [_ w269]
      tunnel: [FALSE TRUE] -> w257
      frame False {
      }
      frame True {
      }
    }
    "DATA ONLINE" <- w257
    "UDP String" <- w253
    n103 = local read "Stop Button"() -> (w266:bool)
    n104 = UDP Write(address=w258, port or service name=w259, connection ID=w262, data in=w260, 8:w261) -> (error out=w263:errorcluster, 3:w264:refnum<k16>)  [unwired: 1 in]
  }
  n105 = UDP Close(connection ID=w12, 8:w11) -> ()  [unwired: 2 out]
  n106 = while {
    tunnel: w19 -> [w304]
    tunnel: w18 -> [w303]
    tunnel: [w302] -> _
    tunnel: [w301] -> _
    tunnel: w4 -> [w279]
    tunnel: w3 -> [w278]
    tunnel: [w277] -> _
    tunnel: [w276] -> _
    stop <- w300 stop-if-true
    w293 = u32 0
    w289 = 4 ("length (rest)")
    # "Data Frame Parsing"
    n107 = Dequeue Element(queue=w304, error in (no error)=w303) -> (queue out=w302:refnum<queue>, element=w299:cluster{"DATA Type":string, "CFG Type":string[]}, error out=w301:errorcluster)  [unwired: 1 in, 1 out]
    n108 = Unbundle By Name(w299) -> ("DATA Type"=w285:string, "CFG Type"=w298:string[])
    "DATA FRAME" <- w285
    n109 = property on="Names of PMUs" class="LstBox (strict)"() -> ("Value"=w271:i32)  [unwired: 2 in, 2 out]
    n110 = String Subset(string=w285, offset (0)=6, length (rest)=w289) -> (substring=w291:string)
    n111 = String Subset(string=w285, offset (0)=10, length (rest)=w289) -> (substring=w287:string)
    n112 = Index Array(array=w298, index=w271) -> (element=w290:string)
    n113 = property on="TIME_BASE" class="DigNum (strict)"() -> ("Value"=w295:u32)  [unwired: 2 in, 2 out]
    n114 = property on="NUM_of_PMUs" class="DigNum (strict)"() -> ("Value"=w297:u32)  [unwired: 2 in, 2 out]
    n115 = Type Cast(type=w293, x=w291) -> (*(type *) &x=w292:u32)
    n116 = Type Cast(type=w293, x=w287) -> (*(type *) &x=w286:u32)
    n117 = call "PMU_INFO.vi"("data in"=w290) -> ("RET_DATA"=w283:T10)
    n118 = call "PMU_DATA_PACK.vi"("DATA FRAME"=w285, "DATA_IN"=w283, "PMUs_NUM"=w297) -> ("PMU DATA Packet"=→"PMU DATA Packet":string[], "DATA_DTLD"=w274:T11)  [unwired: 6 in]
    n119 = call "UNIX-DATE_TIME.vi"("TIME_BASE"=w295, "FRACSEC"=w286, "SOC"=w292) -> ("Date/Time"=w281:string)  [unwired: 1 out]
    n120 = Not Equal?(x=w281, y="1-1-1970, 2:0:0 0.000000") -> (x != y?=w284:bool)
    n121 = Unbundle By Name(w283) -> ("UNITs"=→"UNITs":T2)
    n122 = case shown="True" w284 {
      tunnel: [_ w305] -> w273
      tunnel: w281 -> [_ w305]
      frame False {
      }
      frame True {
      }
    }
    "Date/Time 2" <- w273
    n123 = Bundle By Name(cluster=T7 {"Date/Time"="26-12-2013, 0:30:36 0.866666", "DATA_DTLD"={"PZRs Packet"=[], "FREQ Packet"=[], "DFREQ Packet"=[], "ANG Packet"=[], "DGTL Packet"=[]}}, "DATA_DTLD"=w274, "Date/Time"=w273) -> (w272:T7)
    n124 = Enqueue Element(queue=w279, element=w272, error in (no error)=w278) -> (queue out=w277:refnum<queue>, error out=w276:errorcluster)  [unwired: 1 in, 1 out]
    n125 = local read "Stop Button"() -> (w300:bool)
  }
  n126 = while {
    tunnel: w30 -> [w306]
    stop <- w335 stop-if-true
    # "UI Handling Loop"
    n127 = Index Array(array=w306, index="Names of PMUs") -> (element=w308:string)
    n128 = call "PMU_INFO.vi"("data in"=w308) -> ("RET_DATA"=w331:T10)
    n129 = local read "Stop Button"() -> (w335:bool)
    n130 = Unbundle By Name(w331) -> ("NUMs.PHNMR"=→"No. of Phasors in this PMU":u8)
    n131 = Unbundle By Name(w331) -> ("NUMs.ANNMR"=→"No. of Analogs in this PMU":u8)
    n132 = Unbundle By Name(w331) -> ("NUMs.DGNMR"=w334:u8)
    n133 = Multiply(x=w334, y=u8 16) -> (x*y=→"No. of Digitals in this PMU":u8)
    n134 = local read "No. of Phasors in this PMU"() -> (w311:u8)
    n135 = String Length(string=w308) -> (length=w313:i32)
    n136 = local read "No. of Analogs in this PMU"() -> (w310:u8)
    n137 = String Subset(string=w308, offset (0)=26, length (rest)=w313) -> (substring=w324:string)
    n138 = local read "No. of Digitals in this PMU"() -> (w309:u8)
    n139 = String Length(string=w308) -> (length=w325:i32)
    n140 = Multiply(x=w311, y=u8 16) -> (x*y=w315:u8)
    n141 = String Length(string=w308) -> (length=w323:i32)
    n142 = Multiply(x=w310, y=u8 16) -> (x*y=w319:u8)
    n143 = String Subset(string=w324, offset (0)=w315, length (rest)=w323) -> (substring=w320:string)
    n144 = String Subset(string=w320, offset (0)=w319, length (rest)=w325) -> (substring=w321:string)
    n145 = for {
      N: w311 -> [_]
      tunnel: w324 -> [w353]
      tunnel: [w351] -> w307 mode=indexing
      shift-right: [w348] -> _
      shift-left: 0 ("offset (0)") -> [w350]
      n146 = String Subset(string=w353, offset (0)=w350, length (rest)=16 ("length (rest)")) -> (substring=w351:string)
      n147 = Add(x=w350, y=16) -> (x+y=w348:i32)
    }
    n148 = for {
      N: w310 -> [_]
      tunnel: w320 -> [w347]
      tunnel: [w345] -> w317 mode=indexing
      shift-right: [w342] -> _
      shift-left: 0 ("offset (0)") -> [w344]
      n149 = String Subset(string=w347, offset (0)=w344, length (rest)=16 ("length (rest)")) -> (substring=w345:string)
      n150 = Add(x=w344, y=16) -> (x+y=w342:i32)
    }
    n151 = for {
      N: w309 -> [_]
      tunnel: w321 -> [w341]
      tunnel: [w339] -> w322 mode=indexing
      shift-right: [w336] -> _
      shift-left: 0 ("offset (0)") -> [w338]
      n152 = String Subset(string=w341, offset (0)=w338, length (rest)=16 ("length (rest)")) -> (substring=w339:string)
      n153 = Add(x=w338, y=16) -> (x+y=w336:i32)
    }
    n154 = property on="PMU Analogs" class="LstBox (strict)"("Item Names"=w317) -> ()  [unwired: 2 in, 2 out]
    n155 = property on="PMU Digitals" class="LstBox (strict)"("Item Names"=w322) -> ()  [unwired: 2 in, 2 out]
    n156 = property on="PMU Phasors" class="LstBox (strict)"("Item Names"=w307) -> ()  [unwired: 2 in, 2 out]
    "PMU1 CFG Packet 2" <- w306
  }
  n157 = while {
    tunnel: w63 -> [w355]
    tunnel: w61 -> [w360]
    tunnel: [w358] -> _
    tunnel: [w359] -> _
    stop <- w356 stop-if-true
    # "Send Commands"
    n158 = event shown="[1] \"Stop Button\": Mouse Down" {
      selector: _ -> [_ _ _ _]
      dyn-events: _ -> [_ _ _ _]
      timeout: _ -> [_ _ _ _]
      tunnel: [PMU_CMDs."Turn off Transmission of Data Frame" ("command 2") w369 PMU_CMDs."Turn off Transmission of Data Frame" ("command 2") PMU_CMDs."Turn on Transmission of Data Frame" ("command 2")] -> w361
      tunnel: [TRUE ("Stop Button") TRUE ("Stop Button") FALSE ("Stop Button") FALSE ("Stop Button")] -> w356
      tunnel: [_ _ _ w374] -> w357
      tunnel: w355 -> [_ w370 _ _]
      event Timeout {
        n159 = event-data() -> ()  [unwired: 1 in, 3 out]
      }
      event "Stop Button": Mouse Down {
        w369 = PMU_CMDs."Turn off Transmission of Data Frame" ("command 2")
        n160 = event-data() -> ()  [unwired: 1 in, 4 out]
        n161 = local read "Device ID"() -> (w366:u16)
        n162 = call "CMD.vi"("PMU ID"=w366, "command"=w369) -> ("error out"=w367:errorcluster, "CMD"=w368:string)  [unwired: 4 in]
        n163 = TCP Write(connection ID=w370, data in=w368, error in (no error)=w367) -> ()  [unwired: 1 in, 3 out]
      }
      event "DATA OFF": Mouse Down {
        n164 = event-data() -> ()  [unwired: 1 in, 3 out]
      }
      event "DATA ON": Mouse Down {
        n165 = event-data() -> ()  [unwired: 1 in, 3 out]
        n166 = local read "Size of DATA Frame"() -> (w374:u32)
      }
    }
    "Data size to read" <- w357
    n167 = local read "Device ID"() -> (w354:u16)
    n168 = Stop(stop? (T)=w356) -> ()
    n169 = call "CMD.vi"("PMU ID"=w354, "command"=w361) -> ("CMD"=w362:string)  [unwired: 4 in, 1 out]
    "COMMAND Frame" <- w362
    n170 = TCP Write(connection ID=w355, data in=w362, error in (no error)=w360) -> (connection ID out=w358:refnum<k5>, bytes written=→"bytes written":i32, error out=w359:errorcluster)  [unwired: 1 in]
  }
  n171 = while {
    tunnel: w63 -> [w393]
    tunnel: w61 -> [w392]
    tunnel: [w391] -> _
    tunnel: [w390] -> _
    tunnel: w19 -> [w384]
    tunnel: [w383] -> w36
    tunnel: [w382] -> w35
    tunnel: w18 -> [w381]
    tunnel: w30 -> [w379]
    stop <- w388 stop-if-true
    # "Receive Loop"
    n172 = local read "Data size to read"() -> (w387:u32)
    n173 = TCP Read(connection ID=w393, bytes to read=w387, error in (no error)=w392) -> (connection ID out=w396:refnum<k5>, data out=w394:string, error out=w395:errorcluster)  [unwired: 2 in]
    n174 = String Length(string=w394) -> (length=w389:i32)
    "length" <- w389
    n175 = control-ref of="Data size to read"() -> (w385:refnum<vi>)
    n176 = TCP Read(connection ID=w396, bytes to read=w389, error in (no error)=w395) -> (connection ID out=w391:refnum<k5>, data out=w386:string, error out=w390:errorcluster)  [unwired: 2 in]
    n177 = call "DATA_RSHP.vi"("Digital in"=w385, "data in"=w386) -> ("DATA FRAME"=w380:string)
    n178 = Bundle By Name(cluster=cluster{"DATA Type":string, "CFG Type":string[]} {"DATA Type"="", "CFG Type"=["PMU.001\u0000\u0000\u0000\u0000\u0000\u0000\u0000\u0000\u0000\u0000\u0001\u0000\u000f\u0000\u0006\u0000\u0003\u0000\u0001PZR.AI          PZR.BV          PZR.CI          PZR.AV          PZR.BI          PZR.CV          ANA1            ANA2            ANA3            DIG.stat1_01    DIG.stat1_02    DIG.stat1_03    DIG.stat1_04    DIG.stat1_05    DIG.stat1_06    DIG.stat1_07    DIG.stat1_08    DIG.stat1_09    DIG.stat1_10    DIG.stat1_11    DIG.stat1_12    DIG.stat1_13    DIG.stat1_14    DIG.stat1_15    DIG.stat1_16    \u0001\u0000\u0000\u0000\u0000\u0000\u0000\u0000\u0001\u0000\u0000\u0000\u0000\u0000\u0000\u0000\u0001\u0000\u0000\u0000\u0000\u0000\u0000\u0000\u0000\u0000\u0000\u0000\u0000\u0000\u0000\u0000\u0000\u0000\u0000\u0000ÿÿ\u0000\u0000\u0000\u0000\u0000\u0000", "PMU.002\u0000\u0000\u0000\u0000\u0000\u0000\u0000\u0000\u0000\u0000\u0002\u0000\u000f\u0000\u0006\u0000\u0003\u0000\u0001PZR.AI          PZR.BV          PZR.CI          PZR.AV          PZR.BI          PZR.CV          ANA1            ANA2            ANA3            DIG.stat1_01    DIG.stat1_02    DIG.stat1_03    DIG.stat1_04    DIG.stat1_05    DIG.stat1_06    DIG.stat1_07    DIG.stat1_08    DIG.stat1_09    DIG.stat1_10    DIG.stat1_11    DIG.stat1_12    DIG.stat1_13    DIG.stat1_14    DIG.stat1_15    DIG.stat1_16    \u0001\u0000\u0000\u0000\u0000\u0000\u0000\u0000\u0001\u0000\u0000\u0000\u0000\u0000\u0000\u0000\u0001\u0000\u0000\u0000\u0000\u0000\u0000\u0000\u0000\u0000\u0000\u0000\u0000\u0000\u0000\u0000\u0000\u0000\u0000\u0000ÿÿ\u0000\u0000\u0000\u0000\u0000\u0000", "PMU.003\u0000\u0000\u0000\u0000\u0000\u0000\u0000\u0000\u0000\u0000\u0003\u0000\u000f\u0000\u0006\u0000\u0003\u0000\u0001PZR.AI          PZR.BV          PZR.CI          PZR.AV          PZR.BI          PZR.CV          ANA1            ANA2            ANA3            DIG.stat1_01    DIG.stat1_02    DIG.stat1_03    DIG.stat1_04    DIG.stat1_05    DIG.stat1_06    DIG.stat1_07    DIG.stat1_08    DIG.stat1_09    DIG.stat1_10    DIG.stat1_11    DIG.stat1_12    DIG.stat1_13    DIG.stat1_14    DIG.stat1_15    DIG.stat1_16    \u0001\u0000\u0000\u0000\u0000\u0000\u0000\u0000\u0001\u0000\u0000\u0000\u0000\u0000\u0000\u0000\u0001\u0000\u0000\u0000\u0000\u0000\u0000\u0000\u0000\u0000\u0000\u0000\u0000\u0000\u0000\u0000\u0000\u0000\u0000\u0000ÿÿ\u0000\u0000\u0000\u0000\u0000\u0000", "PMU.004\u0000\u0000\u0000\u0000\u0000\u0000\u0000\u0000\u0000\u0000\u0004\u0000\u000f\u0000\u0006\u0000\u0003\u0000\u0001PZR.AI          PZR.BV          PZR.CI          PZR.AV          PZR.BI          PZR.CV          ANA1            ANA2            ANA3            DIG.stat1_01    DIG.stat1_02    DIG.stat1_03    DIG.stat1_04    DIG.stat1_05    DIG.stat1_06    DIG.stat1_07    DIG.stat1_08    DIG.stat1_09    DIG.stat1_10    DIG.stat1_11    DIG.stat1_12    DIG.stat1_13    DIG.stat1_14    DIG.stat1_15    DIG.stat1_16    \u0001\u0000\u0000\u0000\u0000\u0000\u0000\u0000\u0001\u0000\u0000\u0000\u0000\u0000\u0000\u0000\u0001\u0000\u0000\u0000\u0000\u0000\u0000\u0000\u0000\u0000\u0000\u0000\u0000\u0000\u0000\u0000\u0000\u0000\u0000\u0000ÿÿ\u0000\u0000\u0000\u0000\u0000\u0000", "PMU.005\u0000\u0000\u0000\u0000\u0000\u0000\u0000\u0000\u0000\u0000\u0005\u0000\u000f\u0000\u0006\u0000\u0003\u0000\u0001PZR.AI          PZR.BV          PZR.CI          PZR.AV          PZR.BI          PZR.CV          ANA1            ANA2            ANA3            DIG.stat1_01    DIG.stat1_02    DIG.stat1_03    DIG.stat1_04    DIG.stat1_05    DIG.stat1_06    DIG.stat1_07    DIG.stat1_08    DIG.stat1_09    DIG.stat1_10    DIG.stat1_11    DIG.stat1_12    DIG.stat1_13    DIG.stat1_14    DIG.stat1_15    DIG.stat1_16    \u0001\u0000\u0000\u0000\u0000\u0000\u0000\u0000\u0001\u0000\u0000\u0000\u0000\u0000\u0000\u0000\u0001\u0000\u0000\u0000\u0000\u0000\u0000\u0000\u0000\u0000\u0000\u0000\u0000\u0000\u0000\u0000\u0000\u0000\u0000\u0000ÿÿ\u0000\u0000\u0000\u0000\u0000\u0000", "PMU.006\u0000\u0000\u0000\u0000\u0000\u0000\u0000\u0000\u0000\u0000\u0006\u0000\u000f\u0000\u0006\u0000\u0003\u0000\u0001PZR.AI          PZR.BV          PZR.CI          PZR.AV          PZR.BI          PZR.CV          ANA1            ANA2            ANA3            DIG.stat1_01    DIG.stat1_02    DIG.stat1_03    DIG.stat1_04    DIG.stat1_05    DIG.stat1_06    DIG.stat1_07    DIG.stat1_08    DIG.stat1_09    DIG.stat1_10    DIG.stat1_11    DIG.stat1_12    DIG.stat1_13    DIG.stat1_14    DIG.stat1_15    DIG.stat1_16    \u0001\u0000\u0000\u0000\u0000\u0000\u0000\u0000\u0001\u0000\u0000\u0000\u0000\u0000\u0000\u0000\u0001\u0000\u0000\u0000\u0000\u0000\u0000\u0000\u0000\u0000\u0000\u0000\u0000\u0000\u0000\u0000\u0000\u0000\u0000\u0000ÿÿ\u0000\u0000\u0000\u0000\u0000\u0000", "PMU.007\u0000\u0000\u0000\u0000\u0000\u0000\u0000\u0000\u0000\u0000\u0007\u0000\u000f\u0000\u0006\u0000\u0003\u0000\u0001PZR.AI          PZR.BV          PZR.CI          PZR.AV          PZR.BI          PZR.CV          ANA1            ANA2            ANA3            DIG.stat1_01    DIG.stat1_02    DIG.stat1_03    DIG.stat1_04    DIG.stat1_05    DIG.stat1_06    DIG.stat1_07    DIG.stat1_08    DIG.stat1_09    DIG.stat1_10    DIG.stat1_11    DIG.stat1_12    DIG.stat1_13    DIG.stat1_14    DIG.stat1_15    DIG.stat1_16    \u0001\u0000\u0000\u0000\u0000\u0000\u0000\u0000\u0001\u0000\u0000\u0000\u0000\u0000\u0000\u0000\u0001\u0000\u0000\u0000\u0000\u0000\u0000\u0000\u0000\u0000\u0000\u0000\u0000\u0000\u0000\u0000\u0000\u0000\u0000\u0000ÿÿ\u0000\u0000\u0000\u0000\u0000\u0000", "PMU.008\u0000\u0000\u0000\u0000\u0000\u0000\u0000\u0000\u0000\u0000\b\u0000\u000f\u0000\u0006\u0000\u0003\u0000\u0001PZR.AI          PZR.BV          PZR.CI          PZR.AV          PZR.BI          PZR.CV          ANA1            ANA2            ANA3            DIG.stat1_01    DIG.stat1_02    DIG.stat1_03    DIG.stat1_04    DIG.stat1_05    DIG.stat1_06    DIG.stat1_07    DIG.stat1_08    DIG.stat1_09    DIG.stat1_10    DIG.stat1_11    DIG.stat1_12    DIG.stat1_13    DIG.stat1_14    DIG.stat1_15    DIG.stat1_16    \u0001\u0000\u0000\u0000\u0000\u0000\u0000\u0000\u0001\u0000\u0000\u0000\u0000\u0000\u0000\u0000\u0001\u0000\u0000\u0000\u0000\u0000\u0000\u0000\u0000\u0000\u0000\u0000\u0000\u0000\u0000\u0000\u0000\u0000\u0000\u0000ÿÿ\u0000\u0000\u0000\u0000\u0000\u0000", "PMU.009\u0000\u0000\u0000\u0000\u0000\u0000\u0000\u0000\u0000\u0000\t\u0000\u000f\u0000\u0006\u0000\u0003\u0000\u0001PZR.AI          PZR.BV          PZR.CI          PZR.AV          PZR.BI          PZR.CV          ANA1            ANA2            ANA3            DIG.stat1_01    DIG.stat1_02    DIG.stat1_03    DIG.stat1_04    DIG.stat1_05    DIG.stat1_06    DIG.stat1_07    DIG.stat1_08    DIG.stat1_09    DIG.stat1_10    DIG.stat1_11    DIG.stat1_12    DIG.stat1_13    DIG.stat1_14    DIG.stat1_15    DIG.stat1_16    \u0001\u0000\u0000\u0000\u0000\u0000\u0000\u0000\u0001\u0000\u0000\u0000\u0000\u0000\u0000\u0000\u0001\u0000\u0000\u0000\u0000\u0000\u0000\u0000\u0000\u0000\u0000\u0000\u0000\u0000\u0000\u0000\u0000\u0000\u0000\u0000ÿÿ\u0000\u0000\u0000\u0000\u0000\u0000", "PMU.010\u0000\u0000\u0000\u0000\u0000\u0000\u0000\u0000\u0000\u0000\n\u0000\u000f\u0000\u0006\u0000\u0003\u0000\u0001PZR.AI          PZR.BV          PZR.CI          PZR.AV          PZR.BI          PZR.CV          ANA1            ANA2            ANA3            DIG.stat1_01    DIG.stat1_02    DIG.stat1_03    DIG.stat1_04    DIG.stat1_05    DIG.stat1_06    DIG.stat1_07    DIG.stat1_08    DIG.stat1_09    DIG.stat1_10    DIG.stat1_11    DIG.stat1_12    DIG.stat1_13    DIG.stat1_14    DIG.stat1_15    DIG.stat1_16    \u0001\u0000\u0000\u0000\u0000\u0000\u0000\u0000\u0001\u0000\u0000\u0000\u0000\u0000\u0000\u0000\u0001\u0000\u0000\u0000\u0000\u0000\u0000\u0000\u0000\u0000\u0000\u0000\u0000\u0000\u0000\u0000\u0000\u0000\u0000\u0000ÿÿ\u0000\u0000\u0000\u0000\u0000\u0000", "PMU.011\u0000\u0000\u0000\u0000\u0000\u0000\u0000\u0000\u0000\u0000\u000b\u0000\u000f\u0000\u0006\u0000\u0003\u0000\u0001PZR.AI          PZR.BV          PZR.CI          PZR.AV          PZR.BI          PZR.CV          ANA1            ANA2            ANA3            DIG.stat1_01    DIG.stat1_02    DIG.stat1_03    DIG.stat1_04    DIG.stat1_05    DIG.stat1_06    DIG.stat1_07    DIG.stat1_08    DIG.stat1_09    DIG.stat1_10    DIG.stat1_11    DIG.stat1_12    DIG.stat1_13    DIG.stat1_14    DIG.stat1_15    DIG.stat1_16    \u0001\u0000\u0000\u0000\u0000\u0000\u0000\u0000\u0001\u0000\u0000\u0000\u0000\u0000\u0000\u0000\u0001\u0000\u0000\u0000\u0000\u0000\u0000\u0000\u0000\u0000\u0000\u0000\u0000\u0000\u0000\u0000\u0000\u0000\u0000\u0000ÿÿ\u0000\u0000\u0000\u0000\u0000\u0000", "PMU.012\u0000\u0000\u0000\u0000\u0000\u0000\u0000\u0000\u0000\u0000\f\u0000\u000f\u0000\u0006\u0000\u0003\u0000\u0001PZR.AI          PZR.BV          PZR.CI          PZR.AV          PZR.BI          PZR.CV          ANA1            ANA2            ANA3            DIG.stat1_01    DIG.stat1_02    DIG.stat1_03    DIG.stat1_04    DIG.stat1_05    DIG.stat1_06    DIG.stat1_07    DIG.stat1_08    DIG.stat1_09    DIG.stat1_10    DIG.stat1_11    DIG.stat1_12    DIG.stat1_13    DIG.stat1_14    DIG.stat1_15    DIG.stat1_16    \u0001\u0000\u0000\u0000\u0000\u0000\u0000\u0000\u0001\u0000\u0000\u0000\u0000\u0000\u0000\u0000\u0001\u0000\u0000\u0000\u0000\u0000\u0000\u0000\u0000\u0000\u0000\u0000\u0000\u0000\u0000\u0000\u0000\u0000\u0000\u0000ÿÿ\u0000\u0000\u0000\u0000\u0000\u0000", "PMU.013\u0000\u0000\u0000\u0000\u0000\u0000\u0000\u0000\u0000\u0000\r\u0000\u000f\u0000\u0006\u0000\u0003\u0000\u0001PZR.AI          PZR.BV          PZR.CI          PZR.AV          PZR.BI          PZR.CV          ANA1            ANA2            ANA3            DIG.stat1_01    DIG.stat1_02    DIG.stat1_03    DIG.stat1_04    DIG.stat1_05    DIG.stat1_06    DIG.stat1_07    DIG.stat1_08    DIG.stat1_09    DIG.stat1_10    DIG.stat1_11    DIG.stat1_12    DIG.stat1_13    DIG.stat1_14    DIG.stat1_15    DIG.stat1_16    \u0001\u0000\u0000\u0000\u0000\u0000\u0000\u0000\u0001\u0000\u0000\u0000\u0000\u0000\u0000\u0000\u0001\u0000\u0000\u0000\u0000\u0000\u0000\u0000\u0000\u0000\u0000\u0000\u0000\u0000\u0000\u0000\u0000\u0000\u0000\u0000ÿÿ\u0000\u0000\u0000\u0000\u0000\u0000", "PMU.014\u0000\u0000\u0000\u0000\u0000\u0000\u0000\u0000\u0000\u0000\u000e\u0000\u000f\u0000\u0006\u0000\u0003\u0000\u0001PZR.AI          PZR.BV          PZR.CI          PZR.AV          PZR.BI          PZR.CV          ANA1            ANA2            ANA3            DIG.stat1_01    DIG.stat1_02    DIG.stat1_03    DIG.stat1_04    DIG.stat1_05    DIG.stat1_06    DIG.stat1_07    DIG.stat1_08    DIG.stat1_09    DIG.stat1_10    DIG.stat1_11    DIG.stat1_12    DIG.stat1_13    DIG.stat1_14    DIG.stat1_15    DIG.stat1_16    \u0001\u0000\u0000\u0000\u0000\u0000\u0000\u0000\u0001\u0000\u0000\u0000\u0000\u0000\u0000\u0000\u0001\u0000\u0000\u0000\u0000\u0000\u0000\u0000\u0000\u0000\u0000\u0000\u0000\u0000\u0000\u0000\u0000\u0000\u0000\u0000ÿÿ\u0000\u0000\u0000\u0000\u0000\u0000", "PMU.015\u0000\u0000\u0000\u0000\u0000\u0000\u0000\u0000\u0000\u0000\u000f\u0000\u000f\u0000\u0006\u0000\u0003\u0000\u0001PZR.AI          PZR.BV          PZR.CI          PZR.AV          PZR.BI          PZR.CV          ANA1            ANA2            ANA3            DIG.stat1_01    DIG.stat1_02    DIG.stat1_03    DIG.stat1_04    DIG.stat1_05    DIG.stat1_06    DIG.stat1_07    DIG.stat1_08    DIG.stat1_09    DIG.stat1_10    DIG.stat1_11    DIG.stat1_12    DIG.stat1_13    DIG.stat1_14    DIG.stat1_15    DIG.stat1_16    \u0001\u0000\u0000\u0000\u0000\u0000\u0000\u0000\u0001\u0000\u0000\u0000\u0000\u0000\u0000\u0000\u0001\u0000\u0000\u0000\u0000\u0000\u0000\u0000\u0000\u0000\u0000\u0000\u0000\u0000\u0000\u0000\u0000\u0000\u0000\u0000ÿÿ\u0000\u0000\u0000\u0000\u0000\u0000", "PMU.016\u0000\u0000\u0000\u0000\u0000\u0000\u0000\u0000\u0000\u0000\u0010\u0000\u000f\u0000\u0006\u0000\u0003\u0000\u0001PZR.AI          PZR.BV          PZR.CI          PZR.AV          PZR.BI          PZR.CV          ANA1            ANA2            ANA3            DIG.stat1_01    DIG.stat1_02    DIG.stat1_03    DIG.stat1_04    DIG.stat1_05    DIG.stat1_06    DIG.stat1_07    DIG.stat1_08    DIG.stat1_09    DIG.stat1_10    DIG.stat1_11    DIG.stat1_12    DIG.stat1_13    DIG.stat1_14    DIG.stat1_15    DIG.stat1_16    \u0001\u0000\u0000\u0000\u0000\u0000\u0000\u0000\u0001\u0000\u0000\u0000\u0000\u0000\u0000\u0000\u0001\u0000\u0000\u0000\u0000\u0000\u0000\u0000\u0000\u0000\u0000\u0000\u0000\u0000\u0000\u0000\u0000\u0000\u0000\u0000ÿÿ\u0000\u0000\u0000\u0000\u0000\u0000", "PMU.017\u0000\u0000\u0000\u0000\u0000\u0000\u0000\u0000\u0000\u0000\u0011\u0000\u000f\u0000\u0006\u0000\u0003\u0000\u0001PZR.AI          PZR.BV          PZR.CI          PZR.AV          PZR.BI          PZR.CV          ANA1            ANA2            ANA3            DIG.stat1_01    DIG.stat1_02    DIG.stat1_03    DIG.stat1_04    DIG.stat1_05    DIG.stat1_06    DIG.stat1_07    DIG.stat1_08    DIG.stat1_09    DIG.stat1_10    DIG.stat1_11    DIG.stat1_12    DIG.stat1_13    DIG.stat1_14    DIG.stat1_15    DIG.stat1_16    \u0001\u0000\u0000\u0000\u0000\u0000\u0000\u0000\u0001\u0000\u0000\u0000\u0000\u0000\u0000\u0000\u0001\u0000\u0000\u0000\u0000\u0000\u0000\u0000\u0000\u0000\u0000\u0000\u0000\u0000\u0000\u0000\u0000\u0000\u0000\u0000ÿÿ\u0000\u0000\u0000\u0000\u0000\u0000", "PMU.018\u0000\u0000\u0000\u0000\u0000\u0000\u0000\u0000\u0000\u0000\u0012\u0000\u000f\u0000\u0006\u0000\u0003\u0000\u0001PZR.AI          PZR.BV          PZR.CI          PZR.AV          PZR.BI          PZR.CV          ANA1            ANA2            ANA3            DIG.stat1_01    DIG.stat1_02    DIG.stat1_03    DIG.stat1_04    DIG.stat1_05    DIG.stat1_06    DIG.stat1_07    DIG.stat1_08    DIG.stat1_09    DIG.stat1_10    DIG.stat1_11    DIG.stat1_12    DIG.stat1_13    DIG.stat1_14    DIG.stat1_15    DIG.stat1_16    \u0001\u0000\u0000\u0000\u0000\u0000\u0000\u0000\u0001\u0000\u0000\u0000\u0000\u0000\u0000\u0000\u0001\u0000\u0000\u0000\u0000\u0000\u0000\u0000\u0000\u0000\u0000\u0000\u0000\u0000\u0000\u0000\u0000\u0000\u0000\u0000ÿÿ\u0000\u0000\u0000\u0000\u0000\u0000", "PMU.019\u0000\u0000\u0000\u0000\u0000\u0000\u0000\u0000\u0000\u0000\u0013\u0000\u000f\u0000\u0006\u0000\u0003\u0000\u0001PZR.AI          PZR.BV          PZR.CI          PZR.AV          PZR.BI          PZR.CV          ANA1            ANA2            ANA3            DIG.stat1_01    DIG.stat1_02    DIG.stat1_03    DIG.stat1_04    DIG.stat1_05    DIG.stat1_06    DIG.stat1_07    DIG.stat1_08    DIG.stat1_09    DIG.stat1_10    DIG.stat1_11    DIG.stat1_12    DIG.stat1_13    DIG.stat1_14    DIG.stat1_15    DIG.stat1_16    \u0001\u0000\u0000\u0000\u0000\u0000\u0000\u0000\u0001\u0000\u0000\u0000\u0000\u0000\u0000\u0000\u0001\u0000\u0000\u0000\u0000\u0000\u0000\u0000\u0000\u0000\u0000\u0000\u0000\u0000\u0000\u0000\u0000\u0000\u0000\u0000ÿÿ\u0000\u0000\u0000\u0000\u0000\u0000", "PMU.020\u0000\u0000\u0000\u0000\u0000\u0000\u0000\u0000\u0000\u0000\u0014\u0000\u000f\u0000\u0006\u0000\u0003\u0000\u0001PZR.AI          PZR.BV          PZR.CI          PZR.AV          PZR.BI          PZR.CV          ANA1            ANA2            ANA3            DIG.stat1_01    DIG.stat1_02    DIG.stat1_03    DIG.stat1_04    DIG.stat1_05    DIG.stat1_06    DIG.stat1_07    DIG.stat1_08    DIG.stat1_09    DIG.stat1_10    DIG.stat1_11    DIG.stat1_12    DIG.stat1_13    DIG.stat1_14    DIG.stat1_15    DIG.stat1_16    \u0001\u0000\u0000\u0000\u0000\u0000\u0000\u0000\u0001\u0000\u0000\u0000\u0000\u0000\u0000\u0000\u0001\u0000\u0000\u0000\u0000\u0000\u0000\u0000\u0000\u0000\u0000\u0000\u0000\u0000\u0000\u0000\u0000\u0000\u0000\u0000ÿÿ\u0000\u0000\u0000\u0000\u0000\u0000", "PMU.021\u0000\u0000\u0000\u0000\u0000\u0000\u0000\u0000\u0000\u0000\u0015\u0000\u000f\u0000\u0006\u0000\u0003\u0000\u0001PZR.AI          PZR.BV          PZR.CI          PZR.AV          PZR.BI          PZR.CV          ANA1            ANA2            ANA3            DIG.stat1_01    DIG.stat1_02    DIG.stat1_03    DIG.stat1_04    DIG.stat1_05    DIG.stat1_06    DIG.stat1_07    DIG.stat1_08    DIG.stat1_09    DIG.stat1_10    DIG.stat1_11    DIG.stat1_12    DIG.stat1_13    DIG.stat1_14    DIG.stat1_15    DIG.stat1_16    \u0001\u0000\u0000\u0000\u0000\u0000\u0000\u0000\u0001\u0000\u0000\u0000\u0000\u0000\u0000\u0000\u0001\u0000\u0000\u0000\u0000\u0000\u0000\u0000\u0000\u0000\u0000\u0000\u0000\u0000\u0000\u0000\u0000\u0000\u0000\u0000ÿÿ\u0000\u0000\u0000\u0000\u0000\u0000", "PMU.022\u0000\u0000\u0000\u0000\u0000\u0000\u0000\u0000\u0000\u0000\u0016\u0000\u000f\u0000\u0006\u0000\u0003\u0000\u0001PZR.AI          PZR.BV          PZR.CI          PZR.AV          PZR.BI          PZR.CV          ANA1            ANA2            ANA3            DIG.stat1_01    DIG.stat1_02    DIG.stat1_03    DIG.stat1_04    DIG.stat1_05    DIG.stat1_06    DIG.stat1_07    DIG.stat1_08    DIG.stat1_09    DIG.stat1_10    DIG.stat1_11    DIG.stat1_12    DIG.stat1_13    DIG.stat1_14    DIG.stat1_15    DIG.stat1_16    \u0001\u0000\u0000\u0000\u0000\u0000\u0000\u0000\u0001\u0000\u0000\u0000\u0000\u0000\u0000\u0000\u0001\u0000\u0000\u0000\u0000\u0000\u0000\u0000\u0000\u0000\u0000\u0000\u0000\u0000\u0000\u0000\u0000\u0000\u0000\u0000ÿÿ\u0000\u0000\u0000\u0000\u0000\u0000", "PMU.023\u0000\u0000\u0000\u0000\u0000\u0000\u0000\u0000\u0000\u0000\u0017\u0000\u000f\u0000\u0006\u0000\u0003\u0000\u0001PZR.AI          PZR.BV          PZR.CI          PZR.AV          PZR.BI          PZR.CV          ANA1            ANA2            ANA3            DIG.stat1_01    DIG.stat1_02    DIG.stat1_03    DIG.stat1_04    DIG.stat1_05    DIG.stat1_06    DIG.stat1_07    DIG.stat1_08    DIG.stat1_09    DIG.stat1_10    DIG.stat1_11    DIG.stat1_12    DIG.stat1_13    DIG.stat1_14    DIG.stat1_15    DIG.stat1_16    \u0001\u0000\u0000\u0000\u0000\u0000\u0000\u0000\u0001\u0000\u0000\u0000\u0000\u0000\u0000\u0000\u0001\u0000\u0000\u0000\u0000\u0000\u0000\u0000\u0000\u0000\u0000\u0000\u0000\u0000\u0000\u0000\u0000\u0000\u0000\u0000ÿÿ\u0000\u0000\u0000\u0000\u0000\u0000", "PMU.024\u0000\u0000\u0000\u0000\u0000\u0000\u0000\u0000\u0000\u0000\u0018\u0000\u000f\u0000\u0006\u0000\u0003\u0000\u0001PZR.AI          PZR.BV          PZR.CI          PZR.AV          PZR.BI          PZR.CV          ANA1            ANA2            ANA3            DIG.stat1_01    DIG.stat1_02    DIG.stat1_03    DIG.stat1_04    DIG.stat1_05    DIG.stat1_06    DIG.stat1_07    DIG.stat1_08    DIG.stat1_09    DIG.stat1_10    DIG.stat1_11    DIG.stat1_12    DIG.stat1_13    DIG.stat1_14    DIG.stat1_15    DIG.stat1_16    \u0001\u0000\u0000\u0000\u0000\u0000\u0000\u0000\u0001\u0000\u0000\u0000\u0000\u0000\u0000\u0000\u0001\u0000\u0000\u0000\u0000\u0000\u0000\u0000\u0000\u0000\u0000\u0000\u0000\u0000\u0000\u0000\u0000\u0000\u0000\u0000ÿÿ\u0000\u0000\u0000\u0000\u0000\u0000", "PMU.025\u0000\u0000\u0000\u0000\u0000\u0000\u0000\u0000\u0000\u0000\u0019\u0000\u000f\u0000\u0006\u0000\u0003\u0000\u0001PZR.AI          PZR.BV          PZR.CI          PZR.AV          PZR.BI          PZR.CV          ANA1            ANA2            ANA3            DIG.stat1_01    DIG.stat1_02    DIG.stat1_03    DIG.stat1_04    DIG.stat1_05    DIG.stat1_06    DIG.stat1_07    DIG.stat1_08    DIG.stat1_09    DIG.stat1_10    DIG.stat1_11    DIG.stat1_12    DIG.stat1_13    DIG.stat1_14    DIG.stat1_15    DIG.stat1_16    \u0001\u0000\u0000\u0000\u0000\u0000\u0000\u0000\u0001\u0000\u0000\u0000\u0000\u0000\u0000\u0000\u0001\u0000\u0000\u0000\u0000\u0000\u0000\u0000\u0000\u0000\u0000\u0000\u0000\u0000\u0000\u0000\u0000\u0000\u0000\u0000ÿÿ\u0000\u0000\u0000\u0000\u0000\u0000", "PMU.026\u0000\u0000\u0000\u0000\u0000\u0000\u0000\u0000\u0000\u0000\u001a\u0000\u000f\u0000\u0006\u0000\u0003\u0000\u0001PZR.AI          PZR.BV          PZR.CI          PZR.AV          PZR.BI          PZR.CV          ANA1            ANA2            ANA3            DIG.stat1_01    DIG.stat1_02    DIG.stat1_03    DIG.stat1_04    DIG.stat1_05    DIG.stat1_06    DIG.stat1_07    DIG.stat1_08    DIG.stat1_09    DIG.stat1_10    DIG.stat1_11    DIG.stat1_12    DIG.stat1_13    DIG.stat1_14    DIG.stat1_15    DIG.stat1_16    \u0001\u0000\u0000\u0000\u0000\u0000\u0000\u0000\u0001\u0000\u0000\u0000\u0000\u0000\u0000\u0000\u0001\u0000\u0000\u0000\u0000\u0000\u0000\u0000\u0000\u0000\u0000\u0000\u0000\u0000\u0000\u0000\u0000\u0000\u0000\u0000ÿÿ\u0000\u0000\u0000\u0000\u0000\u0000", "PMU.027\u0000\u0000\u0000\u0000\u0000\u0000\u0000\u0000\u0000\u0000\u001b\u0000\u000f\u0000\u0006\u0000\u0003\u0000\u0001PZR.AI          PZR.BV          PZR.CI          PZR.AV          PZR.BI          PZR.CV          ANA1            ANA2            ANA3            DIG.stat1_01    DIG.stat1_02    DIG.stat1_03    DIG.stat1_04    DIG.stat1_05    DIG.stat1_06    DIG.stat1_07    DIG.stat1_08    DIG.stat1_09    DIG.stat1_10    DIG.stat1_11    DIG.stat1_12    DIG.stat1_13    DIG.stat1_14    DIG.stat1_15    DIG.stat1_16    \u0001\u0000\u0000\u0000\u0000\u0000\u0000\u0000\u0001\u0000\u0000\u0000\u0000\u0000\u0000\u0000\u0001\u0000\u0000\u0000\u0000\u0000\u0000\u0000\u0000\u0000\u0000\u0000\u0000\u0000\u0000\u0000\u0000\u0000\u0000\u0000ÿÿ\u0000\u0000\u0000\u0000\u0000\u0000", "PMU.028\u0000\u0000\u0000\u0000\u0000\u0000\u0000\u0000\u0000\u0000\u001c\u0000\u000f\u0000\u0006\u0000\u0003\u0000\u0001PZR.AI          PZR.BV          PZR.CI          PZR.AV          PZR.BI          PZR.CV          ANA1            ANA2            ANA3            DIG.stat1_01    DIG.stat1_02    DIG.stat1_03    DIG.stat1_04    DIG.stat1_05    DIG.stat1_06    DIG.stat1_07    DIG.stat1_08    DIG.stat1_09    DIG.stat1_10    DIG.stat1_11    DIG.stat1_12    DIG.stat1_13    DIG.stat1_14    DIG.stat1_15    DIG.stat1_16    \u0001\u0000\u0000\u0000\u0000\u0000\u0000\u0000\u0001\u0000\u0000\u0000\u0000\u0000\u0000\u0000\u0001\u0000\u0000\u0000\u0000\u0000\u0000\u0000\u0000\u0000\u0000\u0000\u0000\u0000\u0000\u0000\u0000\u0000\u0000\u0000ÿÿ\u0000\u0000\u0000\u0000\u0000\u0000", "PMU.029\u0000\u0000\u0000\u0000\u0000\u0000\u0000\u0000\u0000\u0000\u001d\u0000\u000f\u0000\u0006\u0000\u0003\u0000\u0001PZR.AI          PZR.BV          PZR.CI          PZR.AV          PZR.BI          PZR.CV          ANA1            ANA2            ANA3            DIG.stat1_01    DIG.stat1_02    DIG.stat1_03    DIG.stat1_04    DIG.stat1_05    DIG.stat1_06    DIG.stat1_07    DIG.stat1_08    DIG.stat1_09    DIG.stat1_10    DIG.stat1_11    DIG.stat1_12    DIG.stat1_13    DIG.stat1_14    DIG.stat1_15    DIG.stat1_16    \u0001\u0000\u0000\u0000\u0000\u0000\u0000\u0000\u0001\u0000\u0000\u0000\u0000\u0000\u0000\u0000\u0001\u0000\u0000\u0000\u0000\u0000\u0000\u0000\u0000\u0000\u0000\u0000\u0000\u0000\u0000\u0000\u0000\u0000\u0000\u0000ÿÿ\u0000\u0000\u0000\u0000\u0000\u0000", "PMU.030\u0000\u0000\u0000\u0000\u0000\u0000\u0000\u0000\u0000\u0000\u001e\u0000\u000f\u0000\u0006\u0000\u0003\u0000\u0001PZR.AI          PZR.BV          PZR.CI          PZR.AV          PZR.BI          PZR.CV          ANA1            ANA2            ANA3            DIG.stat1_01    DIG.stat1_02    DIG.stat1_03    DIG.stat1_04    DIG.stat1_05    DIG.stat1_06    DIG.stat1_07    DIG.stat1_08    DIG.stat1_09    DIG.stat1_10    DIG.stat1_11    DIG.stat1_12    DIG.stat1_13    DIG.stat1_14    DIG.stat1_15    DIG.stat1_16    \u0001\u0000\u0000\u0000\u0000\u0000\u0000\u0000\u0001\u0000\u0000\u0000\u0000\u0000\u0000\u0000\u0001\u0000\u0000\u0000\u0000\u0000\u0000\u0000\u0000\u0000\u0000\u0000\u0000\u0000\u0000\u0000\u0000\u0000\u0000\u0000ÿÿ\u0000\u0000\u0000\u0000\u0000\u0000", "PMU.031\u0000\u0000\u0000\u0000\u0000\u0000\u0000\u0000\u0000\u0000\u001f\u0000\u000f\u0000\u0006\u0000\u0003\u0000\u0001PZR.AI          PZR.BV          PZR.CI          PZR.AV          PZR.BI          PZR.CV          ANA1            ANA2            ANA3            DIG.stat1_01    DIG.stat1_02    DIG.stat1_03    DIG.stat1_04    DIG.stat1_05    DIG.stat1_06    DIG.stat1_07    DIG.stat1_08    DIG.stat1_09    DIG.stat1_10    DIG.stat1_11    DIG.stat1_12    DIG.stat1_13    DIG.stat1_14    DIG.stat1_15    DIG.stat1_16    \u0001\u0000\u0000\u0000\u0000\u0000\u0000\u0000\u0001\u0000\u0000\u0000\u0000\u0000\u0000\u0000\u0001\u0000\u0000\u0000\u0000\u0000\u0000\u0000\u0000\u0000\u0000\u0000\u0000\u0000\u0000\u0000\u0000\u0000\u0000\u0000ÿÿ\u0000\u0000\u0000\u0000\u0000\u0000", "PMU.032\u0000\u0000\u0000\u0000\u0000\u0000\u0000\u0000\u0000\u0000 \u0000\u000f\u0000\u0006\u0000\u0003\u0000\u0001PZR.AI          PZR.BV          PZR.CI          PZR.AV          PZR.BI          PZR.CV          ANA1            ANA2            ANA3            DIG.stat1_01    DIG.stat1_02    DIG.stat1_03    DIG.stat1_04    DIG.stat1_05    DIG.stat1_06    DIG.stat1_07    DIG.stat1_08    DIG.stat1_09    DIG.stat1_10    DIG.stat1_11    DIG.stat1_12    DIG.stat1_13    DIG.stat1_14    DIG.stat1_15    DIG.stat1_16    \u0001\u0000\u0000\u0000\u0000\u0000\u0000\u0000\u0001\u0000\u0000\u0000\u0000\u0000\u0000\u0000\u0001\u0000\u0000\u0000\u0000\u0000\u0000\u0000\u0000\u0000\u0000\u0000\u0000\u0000\u0000\u0000\u0000\u0000\u0000\u0000ÿÿ\u0000\u0000\u0000\u0000\u0000\u0000", "PMU.033\u0000\u0000\u0000\u0000\u0000\u0000\u0000\u0000\u0000\u0000!\u0000\u000f\u0000\u0006\u0000\u0003\u0000\u0001PZR.AI          PZR.BV          PZR.CI          PZR.AV          PZR.BI          PZR.CV          ANA1            ANA2            ANA3            DIG.stat1_01    DIG.stat1_02    DIG.stat1_03    DIG.stat1_04    DIG.stat1_05    DIG.stat1_06    DIG.stat1_07    DIG.stat1_08    DIG.stat1_09    DIG.stat1_10    DIG.stat1_11    DIG.stat1_12    DIG.stat1_13    DIG.stat1_14    DIG.stat1_15    DIG.stat1_16    \u0001\u0000\u0000\u0000\u0000\u0000\u0000\u0000\u0001\u0000\u0000\u0000\u0000\u0000\u0000\u0000\u0001\u0000\u0000\u0000\u0000\u0000\u0000\u0000\u0000\u0000\u0000\u0000\u0000\u0000\u0000\u0000\u0000\u0000\u0000\u0000ÿÿ\u0000\u0000\u0000\u0000\u0000\u0000", "PMU.034\u0000\u0000\u0000\u0000\u0000\u0000\u0000\u0000\u0000\u0000\"\u0000\u000f\u0000\u0006\u0000\u0003\u0000\u0001PZR.AI          PZR.BV          PZR.CI          PZR.AV          PZR.BI          PZR.CV          ANA1            ANA2            ANA3            DIG.stat1_01    DIG.stat1_02    DIG.stat1_03    DIG.stat1_04    DIG.stat1_05    DIG.stat1_06    DIG.stat1_07    DIG.stat1_08    DIG.stat1_09    DIG.stat1_10    DIG.stat1_11    DIG.stat1_12    DIG.stat1_13    DIG.stat1_14    DIG.stat1_15    DIG.stat1_16    \u0001\u0000\u0000\u0000\u0000\u0000\u0000\u0000\u0001\u0000\u0000\u0000\u0000\u0000\u0000\u0000\u0001\u0000\u0000\u0000\u0000\u0000\u0000\u0000\u0000\u0000\u0000\u0000\u0000\u0000\u0000\u0000\u0000\u0000\u0000\u0000ÿÿ\u0000\u0000\u0000\u0000\u0000\u0000", "PMU.035\u0000\u0000\u0000\u0000\u0000\u0000\u0000\u0000\u0000\u0000#\u0000\u000f\u0000\u0006\u0000\u0003\u0000\u0001PZR.AI          PZR.BV          PZR.CI          PZR.AV          PZR.BI          PZR.CV          ANA1            ANA2            ANA3            DIG.stat1_01    DIG.stat1_02    DIG.stat1_03    DIG.stat1_04    DIG.stat1_05    DIG.stat1_06    DIG.stat1_07    DIG.stat1_08    DIG.stat1_09    DIG.stat1_10    DIG.stat1_11    DIG.stat1_12    DIG.stat1_13    DIG.stat1_14    DIG.stat1_15    DIG.stat1_16    \u0001\u0000\u0000\u0000\u0000\u0000\u0000\u0000\u0001\u0000\u0000\u0000\u0000\u0000\u0000\u0000\u0001\u0000\u0000\u0000\u0000\u0000\u0000\u0000\u0000\u0000\u0000\u0000\u0000\u0000\u0000\u0000\u0000\u0000\u0000\u0000ÿÿ\u0000\u0000\u0000\u0000\u0000\u0000", "PMU.036\u0000\u0000\u0000\u0000\u0000\u0000\u0000\u0000\u0000\u0000$\u0000\u000f\u0000\u0006\u0000\u0003\u0000\u0001PZR.AI          PZR.BV          PZR.CI          PZR.AV          PZR.BI          PZR.CV          ANA1            ANA2            ANA3            DIG.stat1_01    DIG.stat1_02    DIG.stat1_03    DIG.stat1_04    DIG.stat1_05    DIG.stat1_06    DIG.stat1_07    DIG.stat1_08    DIG.stat1_09    DIG.stat1_10    DIG.stat1_11    DIG.stat1_12    DIG.stat1_13    DIG.stat1_14    DIG.stat1_15    DIG.stat1_16    \u0001\u0000\u0000\u0000\u0000\u0000\u0000\u0000\u0001\u0000\u0000\u0000\u0000\u0000\u0000\u0000\u0001\u0000\u0000\u0000\u0000\u0000\u0000\u0000\u0000\u0000\u0000\u0000\u0000\u0000\u0000\u0000\u0000\u0000\u0000\u0000ÿÿ\u0000\u0000\u0000\u0000\u0000\u0000", "PMU.037\u0000\u0000\u0000\u0000\u0000\u0000\u0000\u0000\u0000\u0000%\u0000\u000f\u0000\u0006\u0000\u0003\u0000\u0001PZR.AI          PZR.BV          PZR.CI          PZR.AV          PZR.BI          PZR.CV          ANA1            ANA2            ANA3            DIG.stat1_01    DIG.stat1_02    DIG.stat1_03    DIG.stat1_04    DIG.stat1_05    DIG.stat1_06    DIG.stat1_07    DIG.stat1_08    DIG.stat1_09    DIG.stat1_10    DIG.stat1_11    DIG.stat1_12    DIG.stat1_13    DIG.stat1_14    DIG.stat1_15    DIG.stat1_16    \u0001\u0000\u0000\u0000\u0000\u0000\u0000\u0000\u0001\u0000\u0000\u0000\u0000\u0000\u0000\u0000\u0001\u0000\u0000\u0000\u0000\u0000\u0000\u0000\u0000\u0000\u0000\u0000\u0000\u0000\u0000\u0000\u0000\u0000\u0000\u0000ÿÿ\u0000\u0000\u0000\u0000\u0000\u0000", "PMU.038\u0000\u0000\u0000\u0000\u0000\u0000\u0000\u0000\u0000\u0000&\u0000\u000f\u0000\u0006\u0000\u0003\u0000\u0001PZR.AI          PZR.BV          PZR.CI          PZR.AV          PZR.BI          PZR.CV          ANA1            ANA2            ANA3            DIG.stat1_01    DIG.stat1_02    DIG.stat1_03    DIG.stat1_04    DIG.stat1_05    DIG.stat1_06    DIG.stat1_07    DIG.stat1_08    DIG.stat1_09    DIG.stat1_10    DIG.stat1_11    DIG.stat1_12    DIG.stat1_13    DIG.stat1_14    DIG.stat1_15    DIG.stat1_16    \u0001\u0000\u0000\u0000\u0000\u0000\u0000\u0000\u0001\u0000\u0000\u0000\u0000\u0000\u0000\u0000\u0001\u0000\u0000\u0000\u0000\u0000\u0000\u0000\u0000\u0000\u0000\u0000\u0000\u0000\u0000\u0000\u0000\u0000\u0000\u0000ÿÿ\u0000\u0000\u0000\u0000\u0000\u0000", "PMU.039\u0000\u0000\u0000\u0000\u0000\u0000\u0000\u0000\u0000\u0000'\u0000\u000f\u0000\u0006\u0000\u0003\u0000\u0001PZR.AI          PZR.BV          PZR.CI          PZR.AV          PZR.BI          PZR.CV          ANA1            ANA2            ANA3            DIG.stat1_01    DIG.stat1_02    DIG.stat1_03    DIG.stat1_04    DIG.stat1_05    DIG.stat1_06    DIG.stat1_07    DIG.stat1_08    DIG.stat1_09    DIG.stat1_10    DIG.stat1_11    DIG.stat1_12    DIG.stat1_13    DIG.stat1_14    DIG.stat1_15    DIG.stat1_16    \u0001\u0000\u0000\u0000\u0000\u0000\u0000\u0000\u0001\u0000\u0000\u0000\u0000\u0000\u0000\u0000\u0001\u0000\u0000\u0000\u0000\u0000\u0000\u0000\u0000\u0000\u0000\u0000\u0000\u0000\u0000\u0000\u0000\u0000\u0000\u0000ÿÿ\u0000\u0000\u0000\u0000\u0000\u0000", "PMU.040\u0000\u0000\u0000\u0000\u0000\u0000\u0000\u0000\u0000\u0000(\u0000\u000f\u0000\u0006\u0000\u0003\u0000\u0001PZR.AI          PZR.BV          PZR.CI          PZR.AV          PZR.BI          PZR.CV          ANA1            ANA2            ANA3            DIG.stat1_01    DIG.stat1_02    DIG.stat1_03    DIG.stat1_04    DIG.stat1_05    DIG.stat1_06    DIG.stat1_07    DIG.stat1_08    DIG.stat1_09    DIG.stat1_10    DIG.stat1_11    DIG.stat1_12    DIG.stat1_13    DIG.stat1_14    DIG.stat1_15    DIG.stat1_16    \u0001\u0000\u0000\u0000\u0000\u0000\u0000\u0000\u0001\u0000\u0000\u0000\u0000\u0000\u0000\u0000\u0001\u0000\u0000\u0000\u0000\u0000\u0000\u0000\u0000\u0000\u0000\u0000\u0000\u0000\u0000\u0000\u0000\u0000\u0000\u0000ÿÿ\u0000\u0000\u0000\u0000\u0000\u0000", "PMU.041\u0000\u0000\u0000\u0000\u0000\u0000\u0000\u0000\u0000\u0000)\u0000\u000f\u0000\u0006\u0000\u0003\u0000\u0001PZR.AI          PZR.BV          PZR.CI          PZR.AV          PZR.BI          PZR.CV          ANA1            ANA2            ANA3            DIG.stat1_01    DIG.stat1_02    DIG.stat1_03    DIG.stat1_04    DIG.stat1_05    DIG.stat1_06    DIG.stat1_07    DIG.stat1_08    DIG.stat1_09    DIG.stat1_10    DIG.stat1_11    DIG.stat1_12    DIG.stat1_13    DIG.stat1_14    DIG.stat1_15    DIG.stat1_16    \u0001\u0000\u0000\u0000\u0000\u0000\u0000\u0000\u0001\u0000\u0000\u0000\u0000\u0000\u0000\u0000\u0001\u0000\u0000\u0000\u0000\u0000\u0000\u0000\u0000\u0000\u0000\u0000\u0000\u0000\u0000\u0000\u0000\u0000\u0000\u0000ÿÿ\u0000\u0000\u0000\u0000\u0000\u0000", "PMU.042\u0000\u0000\u0000\u0000\u0000\u0000\u0000\u0000\u0000\u0000*\u0000\u000f\u0000\u0006\u0000\u0003\u0000\u0001PZR.AI          PZR.BV          PZR.CI          PZR.AV          PZR.BI          PZR.CV          ANA1            ANA2            ANA3            DIG.stat1_01    DIG.stat1_02    DIG.stat1_03    DIG.stat1_04    DIG.stat1_05    DIG.stat1_06    DIG.stat1_07    DIG.stat1_08    DIG.stat1_09    DIG.stat1_10    DIG.stat1_11    DIG.stat1_12    DIG.stat1_13    DIG.stat1_14    DIG.stat1_15    DIG.stat1_16    \u0001\u0000\u0000\u0000\u0000\u0000\u0000\u0000\u0001\u0000\u0000\u0000\u0000\u0000\u0000\u0000\u0001\u0000\u0000\u0000\u0000\u0000\u0000\u0000\u0000\u0000\u0000\u0000\u0000\u0000\u0000\u0000\u0000\u0000\u0000\u0000ÿÿ\u0000\u0000\u0000\u0000\u0000\u0000", "PMU.043\u0000\u0000\u0000\u0000\u0000\u0000\u0000\u0000\u0000\u0000+\u0000\u000f\u0000\u0006\u0000\u0003\u0000\u0001PZR.AI          PZR.BV          PZR.CI          PZR.AV          PZR.BI          PZR.CV          ANA1            ANA2            ANA3            DIG.stat1_01    DIG.stat1_02    DIG.stat1_03    DIG.stat1_04    DIG.stat1_05    DIG.stat1_06    DIG.stat1_07    DIG.stat1_08    DIG.stat1_09    DIG.stat1_10    DIG.stat1_11    DIG.stat1_12    DIG.stat1_13    DIG.stat1_14    DIG.stat1_15    DIG.stat1_16    \u0001\u0000\u0000\u0000\u0000\u0000\u0000\u0000\u0001\u0000\u0000\u0000\u0000\u0000\u0000\u0000\u0001\u0000\u0000\u0000\u0000\u0000\u0000\u0000\u0000\u0000\u0000\u0000\u0000\u0000\u0000\u0000\u0000\u0000\u0000\u0000ÿÿ\u0000\u0000\u0000\u0000\u0000\u0000", "PMU.044\u0000\u0000\u0000\u0000\u0000\u0000\u0000\u0000\u0000\u0000,\u0000\u000f\u0000\u0006\u0000\u0003\u0000\u0001PZR.AI          PZR.BV          PZR.CI          PZR.AV          PZR.BI          PZR.CV          ANA1            ANA2            ANA3            DIG.stat1_01    DIG.stat1_02    DIG.stat1_03    DIG.stat1_04    DIG.stat1_05    DIG.stat1_06    DIG.stat1_07    DIG.stat1_08    DIG.stat1_09    DIG.stat1_10    DIG.stat1_11    DIG.stat1_12    DIG.stat1_13    DIG.stat1_14    DIG.stat1_15    DIG.stat1_16    \u0001\u0000\u0000\u0000\u0000\u0000\u0000\u0000\u0001\u0000\u0000\u0000\u0000\u0000\u0000\u0000\u0001\u0000\u0000\u0000\u0000\u0000\u0000\u0000\u0000\u0000\u0000\u0000\u0000\u0000\u0000\u0000\u0000\u0000\u0000\u0000ÿÿ\u0000\u0000\u0000\u0000\u0000\u0000", "PMU.045\u0000\u0000\u0000\u0000\u0000\u0000\u0000\u0000\u0000\u0000-\u0000\u000f\u0000\u0006\u0000\u0003\u0000\u0001PZR.AI          PZR.BV          PZR.CI          PZR.AV          PZR.BI          PZR.CV          ANA1            ANA2            ANA3            DIG.stat1_01    DIG.stat1_02    DIG.stat1_03    DIG.stat1_04    DIG.stat1_05    DIG.stat1_06    DIG.stat1_07    DIG.stat1_08    DIG.stat1_09    DIG.stat1_10    DIG.stat1_11    DIG.stat1_12    DIG.stat1_13    DIG.stat1_14    DIG.stat1_15    DIG.stat1_16    \u0001\u0000\u0000\u0000\u0000\u0000\u0000\u0000\u0001\u0000\u0000\u0000\u0000\u0000\u0000\u0000\u0001\u0000\u0000\u0000\u0000\u0000\u0000\u0000\u0000\u0000\u0000\u0000\u0000\u0000\u0000\u0000\u0000\u0000\u0000\u0000ÿÿ\u0000\u0000\u0000\u0000\u0000\u0000", "PMU.046\u0000\u0000\u0000\u0000\u0000\u0000\u0000\u0000\u0000\u0000.\u0000\u000f\u0000\u0006\u0000\u0003\u0000\u0001PZR.AI          PZR.BV          PZR.CI          PZR.AV          PZR.BI          PZR.CV          ANA1            ANA2            ANA3            DIG.stat1_01    DIG.stat1_02    DIG.stat1_03    DIG.stat1_04    DIG.stat1_05    DIG.stat1_06    DIG.stat1_07    DIG.stat1_08    DIG.stat1_09    DIG.stat1_10    DIG.stat1_11    DIG.stat1_12    DIG.stat1_13    DIG.stat1_14    DIG.stat1_15    DIG.stat1_16    \u0001\u0000\u0000\u0000\u0000\u0000\u0000\u0000\u0001\u0000\u0000\u0000\u0000\u0000\u0000\u0000\u0001\u0000\u0000\u0000\u0000\u0000\u0000\u0000\u0000\u0000\u0000\u0000\u0000\u0000\u0000\u0000\u0000\u0000\u0000\u0000ÿÿ\u0000\u0000\u0000\u0000\u0000\u0000", "PMU.047\u0000\u0000\u0000\u0000\u0000\u0000\u0000\u0000\u0000\u0000/\u0000\u000f\u0000\u0006\u0000\u0003\u0000\u0001PZR.AI          PZR.BV          PZR.CI          PZR.AV          PZR.BI          PZR.CV          ANA1            ANA2            ANA3            DIG.stat1_01    DIG.stat1_02    DIG.stat1_03    DIG.stat1_04    DIG.stat1_05    DIG.stat1_06    DIG.stat1_07    DIG.stat1_08    DIG.stat1_09    DIG.stat1_10    DIG.stat1_11    DIG.stat1_12    DIG.stat1_13    DIG.stat1_14    DIG.stat1_15    DIG.stat1_16    \u0001\u0000\u0000\u0000\u0000\u0000\u0000\u0000\u0001\u0000\u0000\u0000\u0000\u0000\u0000\u0000\u0001\u0000\u0000\u0000\u0000\u0000\u0000\u0000\u0000\u0000\u0000\u0000\u0000\u0000\u0000\u0000\u0000\u0000\u0000\u0000ÿÿ\u0000\u0000\u0000\u0000\u0000\u0000", "PMU.048\u0000\u0000\u0000\u0000\u0000\u0000\u0000\u0000\u0000\u00000\u0000\u000f\u0000\u0006\u0000\u0003\u0000\u0001PZR.AI          PZR.BV          PZR.CI          PZR.AV          PZR.BI          PZR.CV          ANA1            ANA2            ANA3            DIG.stat1_01    DIG.stat1_02    DIG.stat1_03    DIG.stat1_04    DIG.stat1_05    DIG.stat1_06    DIG.stat1_07    DIG.stat1_08    DIG.stat1_09    DIG.stat1_10    DIG.stat1_11    DIG.stat1_12    DIG.stat1_13    DIG.stat1_14    DIG.stat1_15    DIG.stat1_16    \u0001\u0000\u0000\u0000\u0000\u0000\u0000\u0000\u0001\u0000\u0000\u0000\u0000\u0000\u0000\u0000\u0001\u0000\u0000\u0000\u0000\u0000\u0000\u0000\u0000\u0000\u0000\u0000\u0000\u0000\u0000\u0000\u0000\u0000\u0000\u0000ÿÿ\u0000\u0000\u0000\u0000\u0000\u0000", "PMU.049\u0000\u0000\u0000\u0000\u0000\u0000\u0000\u0000\u0000\u00001\u0000\u000f\u0000\u0006\u0000\u0003\u0000\u0001PZR.AI          PZR.BV          PZR.CI          PZR.AV          PZR.BI          PZR.CV          ANA1            ANA2            ANA3            DIG.stat1_01    DIG.stat1_02    DIG.stat1_03    DIG.stat1_04    DIG.stat1_05    DIG.stat1_06    DIG.stat1_07    DIG.stat1_08    DIG.stat1_09    DIG.stat1_10    DIG.stat1_11    DIG.stat1_12    DIG.stat1_13    DIG.stat1_14    DIG.stat1_15    DIG.stat1_16    \u0001\u0000\u0000\u0000\u0000\u0000\u0000\u0000\u0001\u0000\u0000\u0000\u0000\u0000\u0000\u0000\u0001\u0000\u0000\u0000\u0000\u0000\u0000\u0000\u0000\u0000\u0000\u0000\u0000\u0000\u0000\u0000\u0000\u0000\u0000\u0000ÿÿ\u0000\u0000\u0000\u0000\u0000\u0000", "PMU.050\u0000\u0000\u0000\u0000\u0000\u0000\u0000\u0000\u0000\u00002\u0000\u000f\u0000\u0006\u0000\u0003\u0000\u0001PZR.AI          PZR.BV          PZR.CI          PZR.AV          PZR.BI          PZR.CV          ANA1            ANA2            ANA3            DIG.stat1_01    DIG.stat1_02    DIG.stat1_03    DIG.stat1_04    DIG.stat1_05    DIG.stat1_06    DIG.stat1_07    DIG.stat1_08    DIG.stat1_09    DIG.stat1_10    DIG.stat1_11    DIG.stat1_12    DIG.stat1_13    DIG.stat1_14    DIG.stat1_15    DIG.stat1_16    \u0001\u0000\u0000\u0000\u0000\u0000\u0000\u0000\u0001\u0000\u0000\u0000\u0000\u0000\u0000\u0000\u0001\u0000\u0000\u0000\u0000\u0000\u0000\u0000\u0000\u0000\u0000\u0000\u0000\u0000\u0000\u0000\u0000\u0000\u0000\u0000ÿÿ\u0000\u0000\u0000\u0000\u0000\u0000", "PMU.051\u0000\u0000\u0000\u0000\u0000\u0000\u0000\u0000\u0000\u00003\u0000\u000f\u0000\u0006\u0000\u0003\u0000\u0001PZR.AI          PZR.BV          PZR.CI          PZR.AV          PZR.BI          PZR.CV          ANA1            ANA2            ANA3            DIG.stat1_01    DIG.stat1_02    DIG.stat1_03    DIG.stat1_04    DIG.stat1_05    DIG.stat1_06    DIG.stat1_07    DIG.stat1_08    DIG.stat1_09    DIG.stat1_10    DIG.stat1_11    DIG.stat1_12    DIG.stat1_13    DIG.stat1_14    DIG.stat1_15    DIG.stat1_16    \u0001\u0000\u0000\u0000\u0000\u0000\u0000\u0000\u0001\u0000\u0000\u0000\u0000\u0000\u0000\u0000\u0001\u0000\u0000\u0000\u0000\u0000\u0000\u0000\u0000\u0000\u0000\u0000\u0000\u0000\u0000\u0000\u0000\u0000\u0000\u0000ÿÿ\u0000\u0000\u0000\u0000\u0000\u0000", "PMU.052\u0000\u0000\u0000\u0000\u0000\u0000\u0000\u0000\u0000\u00004\u0000\u000f\u0000\u0006\u0000\u0003\u0000\u0001PZR.AI          PZR.BV          PZR.CI          PZR.AV          PZR.BI          PZR.CV          ANA1            ANA2            ANA3            DIG.stat1_01    DIG.stat1_02    DIG.stat1_03    DIG.stat1_04    DIG.stat1_05    DIG.stat1_06    DIG.stat1_07    DIG.stat1_08    DIG.stat1_09    DIG.stat1_10    DIG.stat1_11    DIG.stat1_12    DIG.stat1_13    DIG.stat1_14    DIG.stat1_15    DIG.stat1_16    \u0001\u0000\u0000\u0000\u0000\u0000\u0000\u0000\u0001\u0000\u0000\u0000\u0000\u0000\u0000\u0000\u0001\u0000\u0000\u0000\u0000\u0000\u0000\u0000\u0000\u0000\u0000\u0000\u0000\u0000\u0000\u0000\u0000\u0000\u0000\u0000ÿÿ\u0000\u0000\u0000\u0000\u0000\u0000", "PMU.053\u0000\u0000\u0000\u0000\u0000\u0000\u0000\u0000\u0000\u00005\u0000\u000f\u0000\u0006\u0000\u0003\u0000\u0001PZR.AI          PZR.BV          PZR.CI          PZR.AV          PZR.BI          PZR.CV          ANA1            ANA2            ANA3            DIG.stat1_01    DIG.stat1_02    DIG.stat1_03    DIG.stat1_04    DIG.stat1_05    DIG.stat1_06    DIG.stat1_07    DIG.stat1_08    DIG.stat1_09    DIG.stat1_10    DIG.stat1_11    DIG.stat1_12    DIG.stat1_13    DIG.stat1_14    DIG.stat1_15    DIG.stat1_16    \u0001\u0000\u0000\u0000\u0000\u0000\u0000\u0000\u0001\u0000\u0000\u0000\u0000\u0000\u0000\u0000\u0001\u0000\u0000\u0000\u0000\u0000\u0000\u0000\u0000\u0000\u0000\u0000\u0000\u0000\u0000\u0000\u0000\u0000\u0000\u0000ÿÿ\u0000\u0000\u0000\u0000\u0000\u0000", "PMU.054\u0000\u0000\u0000\u0000\u0000\u0000\u0000\u0000\u0000\u00006\u0000\u000f\u0000\u0006\u0000\u0003\u0000\u0001PZR.AI          PZR.BV          PZR.CI          PZR.AV          PZR.BI          PZR.CV          ANA1            ANA2            ANA3            DIG.stat1_01    DIG.stat1_02    DIG.stat1_03    DIG.stat1_04    DIG.stat1_05    DIG.stat1_06    DIG.stat1_07    DIG.stat1_08    DIG.stat1_09    DIG.stat1_10    DIG.stat1_11    DIG.stat1_12    DIG.stat1_13    DIG.stat1_14    DIG.stat1_15    DIG.stat1_16    \u0001\u0000\u0000\u0000\u0000\u0000\u0000\u0000\u0001\u0000\u0000\u0000\u0000\u0000\u0000\u0000\u0001\u0000\u0000\u0000\u0000\u0000\u0000\u0000\u0000\u0000\u0000\u0000\u0000\u0000\u0000\u0000\u0000\u0000\u0000\u0000ÿÿ\u0000\u0000\u0000\u0000\u0000\u0000", "PMU.055\u0000\u0000\u0000\u0000\u0000\u0000\u0000\u0000\u0000\u00007\u0000\u000f\u0000\u0006\u0000\u0003\u0000\u0001PZR.AI          PZR.BV          PZR.CI          PZR.AV          PZR.BI          PZR.CV          ANA1            ANA2            ANA3            DIG.stat1_01    DIG.stat1_02    DIG.stat1_03    DIG.stat1_04    DIG.stat1_05    DIG.stat1_06    DIG.stat1_07    DIG.stat1_08    DIG.stat1_09    DIG.stat1_10    DIG.stat1_11    DIG.stat1_12    DIG.stat1_13    DIG.stat1_14    DIG.stat1_15    DIG.stat1_16    \u0001\u0000\u0000\u0000\u0000\u0000\u0000\u0000\u0001\u0000\u0000\u0000\u0000\u0000\u0000\u0000\u0001\u0000\u0000\u0000\u0000\u0000\u0000\u0000\u0000\u0000\u0000\u0000\u0000\u0000\u0000\u0000\u0000\u0000\u0000\u0000ÿÿ\u0000\u0000\u0000\u0000\u0000\u0000", "PMU.056\u0000\u0000\u0000\u0000\u0000\u0000\u0000\u0000\u0000\u00008\u0000\u000f\u0000\u0006\u0000\u0003\u0000\u0001PZR.AI          PZR.BV          PZR.CI          PZR.AV          PZR.BI          PZR.CV          ANA1            ANA2            ANA3            DIG.stat1_01    DIG.stat1_02    DIG.stat1_03    DIG.stat1_04    DIG.stat1_05    DIG.stat1_06    DIG.stat1_07    DIG.stat1_08    DIG.stat1_09    DIG.stat1_10    DIG.stat1_11    DIG.stat1_12    DIG.stat1_13    DIG.stat1_14    DIG.stat1_15    DIG.stat1_16    \u0001\u0000\u0000\u0000\u0000\u0000\u0000\u0000\u0001\u0000\u0000\u0000\u0000\u0000\u0000\u0000\u0001\u0000\u0000\u0000\u0000\u0000\u0000\u0000\u0000\u0000\u0000\u0000\u0000\u0000\u0000\u0000\u0000\u0000\u0000\u0000ÿÿ\u0000\u0000\u0000\u0000\u0000\u0000", "PMU.057\u0000\u0000\u0000\u0000\u0000\u0000\u0000\u0000\u0000\u00009\u0000\u000f\u0000\u0006\u0000\u0003\u0000\u0001PZR.AI          PZR.BV          PZR.CI          PZR.AV          PZR.BI          PZR.CV          ANA1            ANA2            ANA3            DIG.stat1_01    DIG.stat1_02    DIG.stat1_03    DIG.stat1_04    DIG.stat1_05    DIG.stat1_06    DIG.stat1_07    DIG.stat1_08    DIG.stat1_09    DIG.stat1_10    DIG.stat1_11    DIG.stat1_12    DIG.stat1_13    DIG.stat1_14    DIG.stat1_15    DIG.stat1_16    \u0001\u0000\u0000\u0000\u0000\u0000\u0000\u0000\u0001\u0000\u0000\u0000\u0000\u0000\u0000\u0000\u0001\u0000\u0000\u0000\u0000\u0000\u0000\u0000\u0000\u0000\u0000\u0000\u0000\u0000\u0000\u0000\u0000\u0000\u0000\u0000ÿÿ\u0000\u0000\u0000\u0000\u0000\u0000", "PMU.058\u0000\u0000\u0000\u0000\u0000\u0000\u0000\u0000\u0000\u0000:\u0000\u000f\u0000\u0006\u0000\u0003\u0000\u0001PZR.AI          PZR.BV          PZR.CI          PZR.AV          PZR.BI          PZR.CV          ANA1            ANA2            ANA3            DIG.stat1_01    DIG.stat1_02    DIG.stat1_03    DIG.stat1_04    DIG.stat1_05    DIG.stat1_06    DIG.stat1_07    DIG.stat1_08    DIG.stat1_09    DIG.stat1_10    DIG.stat1_11    DIG.stat1_12    DIG.stat1_13    DIG.stat1_14    DIG.stat1_15    DIG.stat1_16    \u0001\u0000\u0000\u0000\u0000\u0000\u0000\u0000\u0001\u0000\u0000\u0000\u0000\u0000\u0000\u0000\u0001\u0000\u0000\u0000\u0000\u0000\u0000\u0000\u0000\u0000\u0000\u0000\u0000\u0000\u0000\u0000\u0000\u0000\u0000\u0000ÿÿ\u0000\u0000\u0000\u0000\u0000\u0000", "PMU.059\u0000\u0000\u0000\u0000\u0000\u0000\u0000\u0000\u0000\u0000;\u0000\u000f\u0000\u0006\u0000\u0003\u0000\u0001PZR.AI          PZR.BV          PZR.CI          PZR.AV          PZR.BI          PZR.CV          ANA1            ANA2            ANA3            DIG.stat1_01    DIG.stat1_02    DIG.stat1_03    DIG.stat1_04    DIG.stat1_05    DIG.stat1_06    DIG.stat1_07    DIG.stat1_08    DIG.stat1_09    DIG.stat1_10    DIG.stat1_11    DIG.stat1_12    DIG.stat1_13    DIG.stat1_14    DIG.stat1_15    DIG.stat1_16    \u0001\u0000\u0000\u0000\u0000\u0000\u0000\u0000\u0001\u0000\u0000\u0000\u0000\u0000\u0000\u0000\u0001\u0000\u0000\u0000\u0000\u0000\u0000\u0000\u0000\u0000\u0000\u0000\u0000\u0000\u0000\u0000\u0000\u0000\u0000\u0000ÿÿ\u0000\u0000\u0000\u0000\u0000\u0000", "PMU.060\u0000\u0000\u0000\u0000\u0000\u0000\u0000\u0000\u0000\u0000<\u0000\u000f\u0000\u0006\u0000\u0003\u0000\u0001PZR.AI          PZR.BV          PZR.CI          PZR.AV          PZR.BI          PZR.CV          ANA1            ANA2            ANA3            DIG.stat1_01    DIG.stat1_02    DIG.stat1_03    DIG.stat1_04    DIG.stat1_05    DIG.stat1_06    DIG.stat1_07    DIG.stat1_08    DIG.stat1_09    DIG.stat1_10    DIG.stat1_11    DIG.stat1_12    DIG.stat1_13    DIG.stat1_14    DIG.stat1_15    DIG.stat1_16    \u0001\u0000\u0000\u0000\u0000\u0000\u0000\u0000\u0001\u0000\u0000\u0000\u0000\u0000\u0000\u0000\u0001\u0000\u0000\u0000\u0000\u0000\u0000\u0000\u0000\u0000\u0000\u0000\u0000\u0000\u0000\u0000\u0000\u0000\u0000\u0000ÿÿ\u0000\u0000\u0000\u0000\u0000\u0000", "PMU.061\u0000\u0000\u0000\u0000\u0000\u0000\u0000\u0000\u0000\u0000=\u0000\u000f\u0000\u0006\u0000\u0003\u0000\u0001PZR.AI          PZR.BV          PZR.CI          PZR.AV          PZR.BI          PZR.CV          ANA1            ANA2            ANA3            DIG.stat1_01    DIG.stat1_02    DIG.stat1_03    DIG.stat1_04    DIG.stat1_05    DIG.stat1_06    DIG.stat1_07    DIG.stat1_08    DIG.stat1_09    DIG.stat1_10    DIG.stat1_11    DIG.stat1_12    DIG.stat1_13    DIG.stat1_14    DIG.stat1_15    DIG.stat1_16    \u0001\u0000\u0000\u0000\u0000\u0000\u0000\u0000\u0001\u0000\u0000\u0000\u0000\u0000\u0000\u0000\u0001\u0000\u0000\u0000\u0000\u0000\u0000\u0000\u0000\u0000\u0000\u0000\u0000\u0000\u0000\u0000\u0000\u0000\u0000\u0000ÿÿ\u0000\u0000\u0000\u0000\u0000\u0000", "PMU.062\u0000\u0000\u0000\u0000\u0000\u0000\u0000\u0000\u0000\u0000>\u0000\u000f\u0000\u0006\u0000\u0003\u0000\u0001PZR.AI          PZR.BV          PZR.CI          PZR.AV          PZR.BI          PZR.CV          ANA1            ANA2            ANA3            DIG.stat1_01    DIG.stat1_02    DIG.stat1_03    DIG.stat1_04    DIG.stat1_05    DIG.stat1_06    DIG.stat1_07    DIG.stat1_08    DIG.stat1_09    DIG.stat1_10    DIG.stat1_11    DIG.stat1_12    DIG.stat1_13    DIG.stat1_14    DIG.stat1_15    DIG.stat1_16    \u0001\u0000\u0000\u0000\u0000\u0000\u0000\u0000\u0001\u0000\u0000\u0000\u0000\u0000\u0000\u0000\u0001\u0000\u0000\u0000\u0000\u0000\u0000\u0000\u0000\u0000\u0000\u0000\u0000\u0000\u0000\u0000\u0000\u0000\u0000\u0000ÿÿ\u0000\u0000\u0000\u0000\u0000\u0000", "PMU.063\u0000\u0000\u0000\u0000\u0000\u0000\u0000\u0000\u0000\u0000?\u0000\u000f\u0000\u0006\u0000\u0003\u0000\u0001PZR.AI          PZR.BV          PZR.CI          PZR.AV          PZR.BI          PZR.CV          ANA1            ANA2            ANA3            DIG.stat1_01    DIG.stat1_02    DIG.stat1_03    DIG.stat1_04    DIG.stat1_05    DIG.stat1_06    DIG.stat1_07    DIG.stat1_08    DIG.stat1_09    DIG.stat1_10    DIG.stat1_11    DIG.stat1_12    DIG.stat1_13    DIG.stat1_14    DIG.stat1_15    DIG.stat1_16    \u0001\u0000\u0000\u0000\u0000\u0000\u0000\u0000\u0001\u0000\u0000\u0000\u0000\u0000\u0000\u0000\u0001\u0000\u0000\u0000\u0000\u0000\u0000\u0000\u0000\u0000\u0000\u0000\u0000\u0000\u0000\u0000\u0000\u0000\u0000\u0000ÿÿ\u0000\u0000\u0000\u0000\u0000\u0000", "PMU.064\u0000\u0000\u0000\u0000\u0000\u0000\u0000\u0000\u0000\u0000@\u0000\u000f\u0000\u0006\u0000\u0003\u0000\u0001PZR.AI          PZR.BV          PZR.CI          PZR.AV          PZR.BI          PZR.CV          ANA1            ANA2            ANA3            DIG.stat1_01    DIG.stat1_02    DIG.stat1_03    DIG.stat1_04    DIG.stat1_05    DIG.stat1_06    DIG.stat1_07    DIG.stat1_08    DIG.stat1_09    DIG.stat1_10    DIG.stat1_11    DIG.stat1_12    DIG.stat1_13    DIG.stat1_14    DIG.stat1_15    DIG.stat1_16    \u0001\u0000\u0000\u0000\u0000\u0000\u0000\u0000\u0001\u0000\u0000\u0000\u0000\u0000\u0000\u0000\u0001\u0000\u0000\u0000\u0000\u0000\u0000\u0000\u0000\u0000\u0000\u0000\u0000\u0000\u0000\u0000\u0000\u0000\u0000\u0000ÿÿ\u0000\u0000\u0000\u0000\u0000\u0000", "PMU.065\u0000\u0000\u0000\u0000\u0000\u0000\u0000\u0000\u0000\u0000A\u0000\u000f\u0000\u0006\u0000\u0003\u0000\u0001PZR.AI          PZR.BV          PZR.CI          PZR.AV          PZR.BI          PZR.CV          ANA1            ANA2            ANA3            DIG.stat1_01    DIG.stat1_02    DIG.stat1_03    DIG.stat1_04    DIG.stat1_05    DIG.stat1_06    DIG.stat1_07    DIG.stat1_08    DIG.stat1_09    DIG.stat1_10    DIG.stat1_11    DIG.stat1_12    DIG.stat1_13    DIG.stat1_14    DIG.stat1_15    DIG.stat1_16    \u0001\u0000\u0000\u0000\u0000\u0000\u0000\u0000\u0001\u0000\u0000\u0000\u0000\u0000\u0000\u0000\u0001\u0000\u0000\u0000\u0000\u0000\u0000\u0000\u0000\u0000\u0000\u0000\u0000\u0000\u0000\u0000\u0000\u0000\u0000\u0000ÿÿ\u0000\u0000\u0000\u0000\u0000\u0000", "PMU.066\u0000\u0000\u0000\u0000\u0000\u0000\u0000\u0000\u0000\u0000B\u0000\u000f\u0000\u0006\u0000\u0003\u0000\u0001PZR.AI          PZR.BV          PZR.CI          PZR.AV          PZR.BI          PZR.CV          ANA1            ANA2            ANA3            DIG.stat1_01    DIG.stat1_02    DIG.stat1_03    DIG.stat1_04    DIG.stat1_05    DIG.stat1_06    DIG.stat1_07    DIG.stat1_08    DIG.stat1_09    DIG.stat1_10    DIG.stat1_11    DIG.stat1_12    DIG.stat1_13    DIG.stat1_14    DIG.stat1_15    DIG.stat1_16    \u0001\u0000\u0000\u0000\u0000\u0000\u0000\u0000\u0001\u0000\u0000\u0000\u0000\u0000\u0000\u0000\u0001\u0000\u0000\u0000\u0000\u0000\u0000\u0000\u0000\u0000\u0000\u0000\u0000\u0000\u0000\u0000\u0000\u0000\u0000\u0000ÿÿ\u0000\u0000\u0000\u0000\u0000\u0000", "PMU.067\u0000\u0000\u0000\u0000\u0000\u0000\u0000\u0000\u0000\u0000C\u0000\u000f\u0000\u0006\u0000\u0003\u0000\u0001PZR.AI          PZR.BV          PZR.CI          PZR.AV          PZR.BI          PZR.CV          ANA1            ANA2            ANA3            DIG.stat1_01    DIG.stat1_02    DIG.stat1_03    DIG.stat1_04    DIG.stat1_05    DIG.stat1_06    DIG.stat1_07    DIG.stat1_08    DIG.stat1_09    DIG.stat1_10    DIG.stat1_11    DIG.stat1_12    DIG.stat1_13    DIG.stat1_14    DIG.stat1_15    DIG.stat1_16    \u0001\u0000\u0000\u0000\u0000\u0000\u0000\u0000\u0001\u0000\u0000\u0000\u0000\u0000\u0000\u0000\u0001\u0000\u0000\u0000\u0000\u0000\u0000\u0000\u0000\u0000\u0000\u0000\u0000\u0000\u0000\u0000\u0000\u0000\u0000\u0000ÿÿ\u0000\u0000\u0000\u0000\u0000\u0000", "PMU.068\u0000\u0000\u0000\u0000\u0000\u0000\u0000\u0000\u0000\u0000D\u0000\u000f\u0000\u0006\u0000\u0003\u0000\u0001PZR.AI          PZR.BV          PZR.CI          PZR.AV          PZR.BI          PZR.CV          ANA1            ANA2            ANA3            DIG.stat1_01    DIG.stat1_02    DIG.stat1_03    DIG.stat1_04    DIG.stat1_05    DIG.stat1_06    DIG.stat1_07    DIG.stat1_08    DIG.stat1_09    DIG.stat1_10    DIG.stat1_11    DIG.stat1_12    DIG.stat1_13    DIG.stat1_14    DIG.stat1_15    DIG.stat1_16    \u0001\u0000\u0000\u0000\u0000\u0000\u0000\u0000\u0001\u0000\u0000\u0000\u0000\u0000\u0000\u0000\u0001\u0000\u0000\u0000\u0000\u0000\u0000\u0000\u0000\u0000\u0000\u0000\u0000\u0000\u0000\u0000\u0000\u0000\u0000\u0000ÿÿ\u0000\u0000\u0000\u0000\u0000\u0000", "PMU.069\u0000\u0000\u0000\u0000\u0000\u0000\u0000\u0000\u0000\u0000E\u0000\u000f\u0000\u0006\u0000\u0003\u0000\u0001PZR.AI          PZR.BV          PZR.CI          PZR.AV          PZR.BI          PZR.CV          ANA1            ANA2            ANA3            DIG.stat1_01    DIG.stat1_02    DIG.stat1_03    DIG.stat1_04    DIG.stat1_05    DIG.stat1_06    DIG.stat1_07    DIG.stat1_08    DIG.stat1_09    DIG.stat1_10    DIG.stat1_11    DIG.stat1_12    DIG.stat1_13    DIG.stat1_14    DIG.stat1_15    DIG.stat1_16    \u0001\u0000\u0000\u0000\u0000\u0000\u0000\u0000\u0001\u0000\u0000\u0000\u0000\u0000\u0000\u0000\u0001\u0000\u0000\u0000\u0000\u0000\u0000\u0000\u0000\u0000\u0000\u0000\u0000\u0000\u0000\u0000\u0000\u0000\u0000\u0000ÿÿ\u0000\u0000\u0000\u0000\u0000\u0000", "PMU.070\u0000\u0000\u0000\u0000\u0000\u0000\u0000\u0000\u0000\u0000F\u0000\u000f\u0000\u0006\u0000\u0003\u0000\u0001PZR.AI          PZR.BV          PZR.CI          PZR.AV          PZR.BI          PZR.CV          ANA1            ANA2            ANA3            DIG.stat1_01    DIG.stat1_02    DIG.stat1_03    DIG.stat1_04    DIG.stat1_05    DIG.stat1_06    DIG.stat1_07    DIG.stat1_08    DIG.stat1_09    DIG.stat1_10    DIG.stat1_11    DIG.stat1_12    DIG.stat1_13    DIG.stat1_14    DIG.stat1_15    DIG.stat1_16    \u0001\u0000\u0000\u0000\u0000\u0000\u0000\u0000\u0001\u0000\u0000\u0000\u0000\u0000\u0000\u0000\u0001\u0000\u0000\u0000\u0000\u0000\u0000\u0000\u0000\u0000\u0000\u0000\u0000\u0000\u0000\u0000\u0000\u0000\u0000\u0000ÿÿ\u0000\u0000\u0000\u0000\u0000\u0000", "PMU.071\u0000\u0000\u0000\u0000\u0000\u0000\u0000\u0000\u0000\u0000G\u0000\u000f\u0000\u0006\u0000\u0003\u0000\u0001PZR.AI          PZR.BV          PZR.CI          PZR.AV          PZR.BI          PZR.CV          ANA1            ANA2            ANA3            DIG.stat1_01    DIG.stat1_02    DIG.stat1_03    DIG.stat1_04    DIG.stat1_05    DIG.stat1_06    DIG.stat1_07    DIG.stat1_08    DIG.stat1_09    DIG.stat1_10    DIG.stat1_11    DIG.stat1_12    DIG.stat1_13    DIG.stat1_14    DIG.stat1_15    DIG.stat1_16    \u0001\u0000\u0000\u0000\u0000\u0000\u0000\u0000\u0001\u0000\u0000\u0000\u0000\u0000\u0000\u0000\u0001\u0000\u0000\u0000\u0000\u0000\u0000\u0000\u0000\u0000\u0000\u0000\u0000\u0000\u0000\u0000\u0000\u0000\u0000\u0000ÿÿ\u0000\u0000\u0000\u0000\u0000\u0000", "PMU.072\u0000\u0000\u0000\u0000\u0000\u0000\u0000\u0000\u0000\u0000H\u0000\u000f\u0000\u0006\u0000\u0003\u0000\u0001PZR.AI          PZR.BV          PZR.CI          PZR.AV          PZR.BI          PZR.CV          ANA1            ANA2            ANA3            DIG.stat1_01    DIG.stat1_02    DIG.stat1_03    DIG.stat1_04    DIG.stat1_05    DIG.stat1_06    DIG.stat1_07    DIG.stat1_08    DIG.stat1_09    DIG.stat1_10    DIG.stat1_11    DIG.stat1_12    DIG.stat1_13    DIG.stat1_14    DIG.stat1_15    DIG.stat1_16    \u0001\u0000\u0000\u0000\u0000\u0000\u0000\u0000\u0001\u0000\u0000\u0000\u0000\u0000\u0000\u0000\u0001\u0000\u0000\u0000\u0000\u0000\u0000\u0000\u0000\u0000\u0000\u0000\u0000\u0000\u0000\u0000\u0000\u0000\u0000\u0000ÿÿ\u0000\u0000\u0000\u0000\u0000\u0000", "PMU.073\u0000\u0000\u0000\u0000\u0000\u0000\u0000\u0000\u0000\u0000I\u0000\u000f\u0000\u0006\u0000\u0003\u0000\u0001PZR.AI          PZR.BV          PZR.CI          PZR.AV          PZR.BI          PZR.CV          ANA1            ANA2            ANA3            DIG.stat1_01    DIG.stat1_02    DIG.stat1_03    DIG.stat1_04    DIG.stat1_05    DIG.stat1_06    DIG.stat1_07    DIG.stat1_08    DIG.stat1_09    DIG.stat1_10    DIG.stat1_11    DIG.stat1_12    DIG.stat1_13    DIG.stat1_14    DIG.stat1_15    DIG.stat1_16    \u0001\u0000\u0000\u0000\u0000\u0000\u0000\u0000\u0001\u0000\u0000\u0000\u0000\u0000\u0000\u0000\u0001\u0000\u0000\u0000\u0000\u0000\u0000\u0000\u0000\u0000\u0000\u0000\u0000\u0000\u0000\u0000\u0000\u0000\u0000\u0000ÿÿ\u0000\u0000\u0000\u0000\u0000\u0000", "PMU.074\u0000\u0000\u0000\u0000\u0000\u0000\u0000\u0000\u0000\u0000J\u0000\u000f\u0000\u0006\u0000\u0003\u0000\u0001PZR.AI          PZR.BV          PZR.CI          PZR.AV          PZR.BI          PZR.CV          ANA1            ANA2            ANA3            DIG.stat1_01    DIG.stat1_02    DIG.stat1_03    DIG.stat1_04    DIG.stat1_05    DIG.stat1_06    DIG.stat1_07    DIG.stat1_08    DIG.stat1_09    DIG.stat1_10    DIG.stat1_11    DIG.stat1_12    DIG.stat1_13    DIG.stat1_14    DIG.stat1_15    DIG.stat1_16    \u0001\u0000\u0000\u0000\u0000\u0000\u0000\u0000\u0001\u0000\u0000\u0000\u0000\u0000\u0000\u0000\u0001\u0000\u0000\u0000\u0000\u0000\u0000\u0000\u0000\u0000\u0000\u0000\u0000\u0000\u0000\u0000\u0000\u0000\u0000\u0000ÿÿ\u0000\u0000\u0000\u0000\u0000\u0000", "PMU.075\u0000\u0000\u0000\u0000\u0000\u0000\u0000\u0000\u0000\u0000K\u0000\u000f\u0000\u0006\u0000\u0003\u0000\u0001PZR.AI          PZR.BV          PZR.CI          PZR.AV          PZR.BI          PZR.CV          ANA1            ANA2            ANA3            DIG.stat1_01    DIG.stat1_02    DIG.stat1_03    DIG.stat1_04    DIG.stat1_05    DIG.stat1_06    DIG.stat1_07    DIG.stat1_08    DIG.stat1_09    DIG.stat1_10    DIG.stat1_11    DIG.stat1_12    DIG.stat1_13    DIG.stat1_14    DIG.stat1_15    DIG.stat1_16    \u0001\u0000\u0000\u0000\u0000\u0000\u0000\u0000\u0001\u0000\u0000\u0000\u0000\u0000\u0000\u0000\u0001\u0000\u0000\u0000\u0000\u0000\u0000\u0000\u0000\u0000\u0000\u0000\u0000\u0000\u0000\u0000\u0000\u0000\u0000\u0000ÿÿ\u0000\u0000\u0000\u0000\u0000\u0000", "PMU.076\u0000\u0000\u0000\u0000\u0000\u0000\u0000\u0000\u0000\u0000L\u0000\u000f\u0000\u0006\u0000\u0003\u0000\u0001PZR.AI          PZR.BV          PZR.CI          PZR.AV          PZR.BI          PZR.CV          ANA1            ANA2            ANA3            DIG.stat1_01    DIG.stat1_02    DIG.stat1_03    DIG.stat1_04    DIG.stat1_05    DIG.stat1_06    DIG.stat1_07    DIG.stat1_08    DIG.stat1_09    DIG.stat1_10    DIG.stat1_11    DIG.stat1_12    DIG.stat1_13    DIG.stat1_14    DIG.stat1_15    DIG.stat1_16    \u0001\u0000\u0000\u0000\u0000\u0000\u0000\u0000\u0001\u0000\u0000\u0000\u0000\u0000\u0000\u0000\u0001\u0000\u0000\u0000\u0000\u0000\u0000\u0000\u0000\u0000\u0000\u0000\u0000\u0000\u0000\u0000\u0000\u0000\u0000\u0000ÿÿ\u0000\u0000\u0000\u0000\u0000\u0000", "PMU.077\u0000\u0000\u0000\u0000\u0000\u0000\u0000\u0000\u0000\u0000M\u0000\u000f\u0000\u0006\u0000\u0003\u0000\u0001PZR.AI          PZR.BV          PZR.CI          PZR.AV          PZR.BI          PZR.CV          ANA1            ANA2            ANA3            DIG.stat1_01    DIG.stat1_02    DIG.stat1_03    DIG.stat1_04    DIG.stat1_05    DIG.stat1_06    DIG.stat1_07    DIG.stat1_08    DIG.stat1_09    DIG.stat1_10    DIG.stat1_11    DIG.stat1_12    DIG.stat1_13    DIG.stat1_14    DIG.stat1_15    DIG.stat1_16    \u0001\u0000\u0000\u0000\u0000\u0000\u0000\u0000\u0001\u0000\u0000\u0000\u0000\u0000\u0000\u0000\u0001\u0000\u0000\u0000\u0000\u0000\u0000\u0000\u0000\u0000\u0000\u0000\u0000\u0000\u0000\u0000\u0000\u0000\u0000\u0000ÿÿ\u0000\u0000\u0000\u0000\u0000\u0000", "PMU.078\u0000\u0000\u0000\u0000\u0000\u0000\u0000\u0000\u0000\u0000N\u0000\u000f\u0000\u0006\u0000\u0003\u0000\u0001PZR.AI          PZR.BV          PZR.CI          PZR.AV          PZR.BI          PZR.CV          ANA1            ANA2            ANA3            DIG.stat1_01    DIG.stat1_02    DIG.stat1_03    DIG.stat1_04    DIG.stat1_05    DIG.stat1_06    DIG.stat1_07    DIG.stat1_08    DIG.stat1_09    DIG.stat1_10    DIG.stat1_11    DIG.stat1_12    DIG.stat1_13    DIG.stat1_14    DIG.stat1_15    DIG.stat1_16    \u0001\u0000\u0000\u0000\u0000\u0000\u0000\u0000\u0001\u0000\u0000\u0000\u0000\u0000\u0000\u0000\u0001\u0000\u0000\u0000\u0000\u0000\u0000\u0000\u0000\u0000\u0000\u0000\u0000\u0000\u0000\u0000\u0000\u0000\u0000\u0000ÿÿ\u0000\u0000\u0000\u0000\u0000\u0000", "PMU.079\u0000\u0000\u0000\u0000\u0000\u0000\u0000\u0000\u0000\u0000O\u0000\u000f\u0000\u0006\u0000\u0003\u0000\u0001PZR.AI          PZR.BV          PZR.CI          PZR.AV          PZR.BI          PZR.CV          ANA1            ANA2            ANA3            DIG.stat1_01    DIG.stat1_02    DIG.stat1_03    DIG.stat1_04    DIG.stat1_05    DIG.stat1_06    DIG.stat1_07    DIG.stat1_08    DIG.stat1_09    DIG.stat1_10    DIG.stat1_11    DIG.stat1_12    DIG.stat1_13    DIG.stat1_14    DIG.stat1_15    DIG.stat1_16    \u0001\u0000\u0000\u0000\u0000\u0000\u0000\u0000\u0001\u0000\u0000\u0000\u0000\u0000\u0000\u0000\u0001\u0000\u0000\u0000\u0000\u0000\u0000\u0000\u0000\u0000\u0000\u0000\u0000\u0000\u0000\u0000\u0000\u0000\u0000\u0000ÿÿ\u0000\u0000\u0000\u0000\u0000\u0000", "PMU.080\u0000\u0000\u0000\u0000\u0000\u0000\u0000\u0000\u0000\u0000P\u0000\u000f\u0000\u0006\u0000\u0003\u0000\u0001PZR.AI          PZR.BV          PZR.CI          PZR.AV          PZR.BI          PZR.CV          ANA1            ANA2            ANA3            DIG.stat1_01    DIG.stat1_02    DIG.stat1_03    DIG.stat1_04    DIG.stat1_05    DIG.stat1_06    DIG.stat1_07    DIG.stat1_08    DIG.stat1_09    DIG.stat1_10    DIG.stat1_11    DIG.stat1_12    DIG.stat1_13    DIG.stat1_14    DIG.stat1_15    DIG.stat1_16    \u0001\u0000\u0000\u0000\u0000\u0000\u0000\u0000\u0001\u0000\u0000\u0000\u0000\u0000\u0000\u0000\u0001\u0000\u0000\u0000\u0000\u0000\u0000\u0000\u0000\u0000\u0000\u0000\u0000\u0000\u0000\u0000\u0000\u0000\u0000\u0000ÿÿ\u0000\u0000\u0000\u0000\u0000\u0000", "PMU.081\u0000\u0000\u0000\u0000\u0000\u0000\u0000\u0000\u0000\u0000Q\u0000\u000f\u0000\u0006\u0000\u0003\u0000\u0001PZR.AI          PZR.BV          PZR.CI          PZR.AV          PZR.BI          PZR.CV          ANA1            ANA2            ANA3            DIG.stat1_01    DIG.stat1_02    DIG.stat1_03    DIG.stat1_04    DIG.stat1_05    DIG.stat1_06    DIG.stat1_07    DIG.stat1_08    DIG.stat1_09    DIG.stat1_10    DIG.stat1_11    DIG.stat1_12    DIG.stat1_13    DIG.stat1_14    DIG.stat1_15    DIG.stat1_16    \u0001\u0000\u0000\u0000\u0000\u0000\u0000\u0000\u0001\u0000\u0000\u0000\u0000\u0000\u0000\u0000\u0001\u0000\u0000\u0000\u0000\u0000\u0000\u0000\u0000\u0000\u0000\u0000\u0000\u0000\u0000\u0000\u0000\u0000\u0000\u0000ÿÿ\u0000\u0000\u0000\u0000\u0000\u0000", "PMU.082\u0000\u0000\u0000\u0000\u0000\u0000\u0000\u0000\u0000\u0000R\u0000\u000f\u0000\u0006\u0000\u0003\u0000\u0001PZR.AI          PZR.BV          PZR.CI          PZR.AV          PZR.BI          PZR.CV          ANA1            ANA2            ANA3            DIG.stat1_01    DIG.stat1_02    DIG.stat1_03    DIG.stat1_04    DIG.stat1_05    DIG.stat1_06    DIG.stat1_07    DIG.stat1_08    DIG.stat1_09    DIG.stat1_10    DIG.stat1_11    DIG.stat1_12    DIG.stat1_13    DIG.stat1_14    DIG.stat1_15    DIG.stat1_16    \u0001\u0000\u0000\u0000\u0000\u0000\u0000\u0000\u0001\u0000\u0000\u0000\u0000\u0000\u0000\u0000\u0001\u0000\u0000\u0000\u0000\u0000\u0000\u0000\u0000\u0000\u0000\u0000\u0000\u0000\u0000\u0000\u0000\u0000\u0000\u0000ÿÿ\u0000\u0000\u0000\u0000\u0000\u0000", "PMU.083\u0000\u0000\u0000\u0000\u0000\u0000\u0000\u0000\u0000\u0000S\u0000\u000f\u0000\u0006\u0000\u0003\u0000\u0001PZR.AI          PZR.BV          PZR.CI          PZR.AV          PZR.BI          PZR.CV          ANA1            ANA2            ANA3            DIG.stat1_01    DIG.stat1_02    DIG.stat1_03    DIG.stat1_04    DIG.stat1_05    DIG.stat1_06    DIG.stat1_07    DIG.stat1_08    DIG.stat1_09    DIG.stat1_10    DIG.stat1_11    DIG.stat1_12    DIG.stat1_13    DIG.stat1_14    DIG.stat1_15    DIG.stat1_16    \u0001\u0000\u0000\u0000\u0000\u0000\u0000\u0000\u0001\u0000\u0000\u0000\u0000\u0000\u0000\u0000\u0001\u0000\u0000\u0000\u0000\u0000\u0000\u0000\u0000\u0000\u0000\u0000\u0000\u0000\u0000\u0000\u0000\u0000\u0000\u0000ÿÿ\u0000\u0000\u0000\u0000\u0000\u0000", "PMU.084\u0000\u0000\u0000\u0000\u0000\u0000\u0000\u0000\u0000\u0000T\u0000\u000f\u0000\u0006\u0000\u0003\u0000\u0001PZR.AI          PZR.BV          PZR.CI          PZR.AV          PZR.BI          PZR.CV          ANA1            ANA2            ANA3            DIG.stat1_01    DIG.stat1_02    DIG.stat1_03    DIG.stat1_04    DIG.stat1_05    DIG.stat1_06    DIG.stat1_07    DIG.stat1_08    DIG.stat1_09    DIG.stat1_10    DIG.stat1_11    DIG.stat1_12    DIG.stat1_13    DIG.stat1_14    DIG.stat1_15    DIG.stat1_16    \u0001\u0000\u0000\u0000\u0000\u0000\u0000\u0000\u0001\u0000\u0000\u0000\u0000\u0000\u0000\u0000\u0001\u0000\u0000\u0000\u0000\u0000\u0000\u0000\u0000\u0000\u0000\u0000\u0000\u0000\u0000\u0000\u0000\u0000\u0000\u0000ÿÿ\u0000\u0000\u0000\u0000\u0000\u0000", "PMU.085\u0000\u0000\u0000\u0000\u0000\u0000\u0000\u0000\u0000\u0000U\u0000\u000f\u0000\u0006\u0000\u0003\u0000\u0001PZR.AI          PZR.BV          PZR.CI          PZR.AV          PZR.BI          PZR.CV          ANA1            ANA2            ANA3            DIG.stat1_01    DIG.stat1_02    DIG.stat1_03    DIG.stat1_04    DIG.stat1_05    DIG.stat1_06    DIG.stat1_07    DIG.stat1_08    DIG.stat1_09    DIG.stat1_10    DIG.stat1_11    DIG.stat1_12    DIG.stat1_13    DIG.stat1_14    DIG.stat1_15    DIG.stat1_16    \u0001\u0000\u0000\u0000\u0000\u0000\u0000\u0000\u0001\u0000\u0000\u0000\u0000\u0000\u0000\u0000\u0001\u0000\u0000\u0000\u0000\u0000\u0000\u0000\u0000\u0000\u0000\u0000\u0000\u0000\u0000\u0000\u0000\u0000\u0000\u0000ÿÿ\u0000\u0000\u0000\u0000\u0000\u0000", "PMU.086\u0000\u0000\u0000\u0000\u0000\u0000\u0000\u0000\u0000\u0000V\u0000\u000f\u0000\u0006\u0000\u0003\u0000\u0001PZR.AI          PZR.BV          PZR.CI          PZR.AV          PZR.BI          PZR.CV          ANA1            ANA2            ANA3            DIG.stat1_01    DIG.stat1_02    DIG.stat1_03    DIG.stat1_04    DIG.stat1_05    DIG.stat1_06    DIG.stat1_07    DIG.stat1_08    DIG.stat1_09    DIG.stat1_10    DIG.stat1_11    DIG.stat1_12    DIG.stat1_13    DIG.stat1_14    DIG.stat1_15    DIG.stat1_16    \u0001\u0000\u0000\u0000\u0000\u0000\u0000\u0000\u0001\u0000\u0000\u0000\u0000\u0000\u0000\u0000\u0001\u0000\u0000\u0000\u0000\u0000\u0000\u0000\u0000\u0000\u0000\u0000\u0000\u0000\u0000\u0000\u0000\u0000\u0000\u0000ÿÿ\u0000\u0000\u0000\u0000\u0000\u0000", "PMU.087\u0000\u0000\u0000\u0000\u0000\u0000\u0000\u0000\u0000\u0000W\u0000\u000f\u0000\u0006\u0000\u0003\u0000\u0001PZR.AI          PZR.BV          PZR.CI          PZR.AV          PZR.BI          PZR.CV          ANA1            ANA2            ANA3            DIG.stat1_01    DIG.stat1_02    DIG.stat1_03    DIG.stat1_04    DIG.stat1_05    DIG.stat1_06    DIG.stat1_07    DIG.stat1_08    DIG.stat1_09    DIG.stat1_10    DIG.stat1_11    DIG.stat1_12    DIG.stat1_13    DIG.stat1_14    DIG.stat1_15    DIG.stat1_16    \u0001\u0000\u0000\u0000\u0000\u0000\u0000\u0000\u0001\u0000\u0000\u0000\u0000\u0000\u0000\u0000\u0001\u0000\u0000\u0000\u0000\u0000\u0000\u0000\u0000\u0000\u0000\u0000\u0000\u0000\u0000\u0000\u0000\u0000\u0000\u0000ÿÿ\u0000\u0000\u0000\u0000\u0000\u0000", "PMU.088\u0000\u0000\u0000\u0000\u0000\u0000\u0000\u0000\u0000\u0000X\u0000\u000f\u0000\u0006\u0000\u0003\u0000\u0001PZR.AI          PZR.BV          PZR.CI          PZR.AV          PZR.BI          PZR.CV          ANA1            ANA2            ANA3            DIG.stat1_01    DIG.stat1_02    DIG.stat1_03    DIG.stat1_04    DIG.stat1_05    DIG.stat1_06    DIG.stat1_07    DIG.stat1_08    DIG.stat1_09    DIG.stat1_10    DIG.stat1_11    DIG.stat1_12    DIG.stat1_13    DIG.stat1_14    DIG.stat1_15    DIG.stat1_16    \u0001\u0000\u0000\u0000\u0000\u0000\u0000\u0000\u0001\u0000\u0000\u0000\u0000\u0000\u0000\u0000\u0001\u0000\u0000\u0000\u0000\u0000\u0000\u0000\u0000\u0000\u0000\u0000\u0000\u0000\u0000\u0000\u0000\u0000\u0000\u0000ÿÿ\u0000\u0000\u0000\u0000\u0000\u0000", "PMU.089\u0000\u0000\u0000\u0000\u0000\u0000\u0000\u0000\u0000\u0000Y\u0000\u000f\u0000\u0006\u0000\u0003\u0000\u0001PZR.AI          PZR.BV          PZR.CI          PZR.AV          PZR.BI          PZR.CV          ANA1            ANA2            ANA3            DIG.stat1_01    DIG.stat1_02    DIG.stat1_03    DIG.stat1_04    DIG.stat1_05    DIG.stat1_06    DIG.stat1_07    DIG.stat1_08    DIG.stat1_09    DIG.stat1_10    DIG.stat1_11    DIG.stat1_12    DIG.stat1_13    DIG.stat1_14    DIG.stat1_15    DIG.stat1_16    \u0001\u0000\u0000\u0000\u0000\u0000\u0000\u0000\u0001\u0000\u0000\u0000\u0000\u0000\u0000\u0000\u0001\u0000\u0000\u0000\u0000\u0000\u0000\u0000\u0000\u0000\u0000\u0000\u0000\u0000\u0000\u0000\u0000\u0000\u0000\u0000ÿÿ\u0000\u0000\u0000\u0000\u0000\u0000", "PMU.090\u0000\u0000\u0000\u0000\u0000\u0000\u0000\u0000\u0000\u0000Z\u0000\u000f\u0000\u0006\u0000\u0003\u0000\u0001PZR.AI          PZR.BV          PZR.CI          PZR.AV          PZR.BI          PZR.CV          ANA1            ANA2            ANA3            DIG.stat1_01    DIG.stat1_02    DIG.stat1_03    DIG.stat1_04    DIG.stat1_05    DIG.stat1_06    DIG.stat1_07    DIG.stat1_08    DIG.stat1_09    DIG.stat1_10    DIG.stat1_11    DIG.stat1_12    DIG.stat1_13    DIG.stat1_14    DIG.stat1_15    DIG.stat1_16    \u0001\u0000\u0000\u0000\u0000\u0000\u0000\u0000\u0001\u0000\u0000\u0000\u0000\u0000\u0000\u0000\u0001\u0000\u0000\u0000\u0000\u0000\u0000\u0000\u0000\u0000\u0000\u0000\u0000\u0000\u0000\u0000\u0000\u0000\u0000\u0000ÿÿ\u0000\u0000\u0000\u0000\u0000\u0000", "PMU.091\u0000\u0000\u0000\u0000\u0000\u0000\u0000\u0000\u0000\u0000[\u0000\u000f\u0000\u0006\u0000\u0003\u0000\u0001PZR.AI          PZR.BV          PZR.CI          PZR.AV          PZR.BI          PZR.CV          ANA1            ANA2            ANA3            DIG.stat1_01    DIG.stat1_02    DIG.stat1_03    DIG.stat1_04    DIG.stat1_05    DIG.stat1_06    DIG.stat1_07    DIG.stat1_08    DIG.stat1_09    DIG.stat1_10    DIG.stat1_11    DIG.stat1_12    DIG.stat1_13    DIG.stat1_14    DIG.stat1_15    DIG.stat1_16    \u0001\u0000\u0000\u0000\u0000\u0000\u0000\u0000\u0001\u0000\u0000\u0000\u0000\u0000\u0000\u0000\u0001\u0000\u0000\u0000\u0000\u0000\u0000\u0000\u0000\u0000\u0000\u0000\u0000\u0000\u0000\u0000\u0000\u0000\u0000\u0000ÿÿ\u0000\u0000\u0000\u0000\u0000\u0000", "PMU.092\u0000\u0000\u0000\u0000\u0000\u0000\u0000\u0000\u0000\u0000\\\u0000\u000f\u0000\u0006\u0000\u0003\u0000\u0001PZR.AI          PZR.BV          PZR.CI          PZR.AV          PZR.BI          PZR.CV          ANA1            ANA2            ANA3            DIG.stat1_01    DIG.stat1_02    DIG.stat1_03    DIG.stat1_04    DIG.stat1_05    DIG.stat1_06    DIG.stat1_07    DIG.stat1_08    DIG.stat1_09    DIG.stat1_10    DIG.stat1_11    DIG.stat1_12    DIG.stat1_13    DIG.stat1_14    DIG.stat1_15    DIG.stat1_16    \u0001\u0000\u0000\u0000\u0000\u0000\u0000\u0000\u0001\u0000\u0000\u0000\u0000\u0000\u0000\u0000\u0001\u0000\u0000\u0000\u0000\u0000\u0000\u0000\u0000\u0000\u0000\u0000\u0000\u0000\u0000\u0000\u0000\u0000\u0000\u0000ÿÿ\u0000\u0000\u0000\u0000\u0000\u0000", "PMU.093\u0000\u0000\u0000\u0000\u0000\u0000\u0000\u0000\u0000\u0000]\u0000\u000f\u0000\u0006\u0000\u0003\u0000\u0001PZR.AI          PZR.BV          PZR.CI          PZR.AV          PZR.BI          PZR.CV          ANA1            ANA2            ANA3            DIG.stat1_01    DIG.stat1_02    DIG.stat1_03    DIG.stat1_04    DIG.stat1_05    DIG.stat1_06    DIG.stat1_07    DIG.stat1_08    DIG.stat1_09    DIG.stat1_10    DIG.stat1_11    DIG.stat1_12    DIG.stat1_13    DIG.stat1_14    DIG.stat1_15    DIG.stat1_16    \u0001\u0000\u0000\u0000\u0000\u0000\u0000\u0000\u0001\u0000\u0000\u0000\u0000\u0000\u0000\u0000\u0001\u0000\u0000\u0000\u0000\u0000\u0000\u0000\u0000\u0000\u0000\u0000\u0000\u0000\u0000\u0000\u0000\u0000\u0000\u0000ÿÿ\u0000\u0000\u0000\u0000\u0000\u0000", "PMU.094\u0000\u0000\u0000\u0000\u0000\u0000\u0000\u0000\u0000\u0000^\u0000\u000f\u0000\u0006\u0000\u0003\u0000\u0001PZR.AI          PZR.BV          PZR.CI          PZR.AV          PZR.BI          PZR.CV          ANA1            ANA2            ANA3            DIG.stat1_01    DIG.stat1_02    DIG.stat1_03    DIG.stat1_04    DIG.stat1_05    DIG.stat1_06    DIG.stat1_07    DIG.stat1_08    DIG.stat1_09    DIG.stat1_10    DIG.stat1_11    DIG.stat1_12    DIG.stat1_13    DIG.stat1_14    DIG.stat1_15    DIG.stat1_16    \u0001\u0000\u0000\u0000\u0000\u0000\u0000\u0000\u0001\u0000\u0000\u0000\u0000\u0000\u0000\u0000\u0001\u0000\u0000\u0000\u0000\u0000\u0000\u0000\u0000\u0000\u0000\u0000\u0000\u0000\u0000\u0000\u0000\u0000\u0000\u0000ÿÿ\u0000\u0000\u0000\u0000\u0000\u0000", "PMU.095\u0000\u0000\u0000\u0000\u0000\u0000\u0000\u0000\u0000\u0000_\u0000\u000f\u0000\u0006\u0000\u0003\u0000\u0001PZR.AI          PZR.BV          PZR.CI          PZR.AV          PZR.BI          PZR.CV          ANA1            ANA2            ANA3            DIG.stat1_01    DIG.stat1_02    DIG.stat1_03    DIG.stat1_04    DIG.stat1_05    DIG.stat1_06    DIG.stat1_07    DIG.stat1_08    DIG.stat1_09    DIG.stat1_10    DIG.stat1_11    DIG.stat1_12    DIG.stat1_13    DIG.stat1_14    DIG.stat1_15    DIG.stat1_16    \u0001\u0000\u0000\u0000\u0000\u0000\u0000\u0000\u0001\u0000\u0000\u0000\u0000\u0000\u0000\u0000\u0001\u0000\u0000\u0000\u0000\u0000\u0000\u0000\u0000\u0000\u0000\u0000\u0000\u0000\u0000\u0000\u0000\u0000\u0000\u0000ÿÿ\u0000\u0000\u0000\u0000\u0000\u0000", "PMU.096\u0000\u0000\u0000\u0000\u0000\u0000\u0000\u0000\u0000\u0000`\u0000\u000f\u0000\u0006\u0000\u0003\u0000\u0001PZR.AI          PZR.BV          PZR.CI          PZR.AV          PZR.BI          PZR.CV          ANA1            ANA2            ANA3            DIG.stat1_01    DIG.stat1_02    DIG.stat1_03    DIG.stat1_04    DIG.stat1_05    DIG.stat1_06    DIG.stat1_07    DIG.stat1_08    DIG.stat1_09    DIG.stat1_10    DIG.stat1_11    DIG.stat1_12    DIG.stat1_13    DIG.stat1_14    DIG.stat1_15    DIG.stat1_16    \u0001\u0000\u0000\u0000\u0000\u0000\u0000\u0000\u0001\u0000\u0000\u0000\u0000\u0000\u0000\u0000\u0001\u0000\u0000\u0000\u0000\u0000\u0000\u0000\u0000\u0000\u0000\u0000\u0000\u0000\u0000\u0000\u0000\u0000\u0000\u0000ÿÿ\u0000\u0000\u0000\u0000\u0000\u0000", "PMU.097\u0000\u0000\u0000\u0000\u0000\u0000\u0000\u0000\u0000\u0000a\u0000\u000f\u0000\u0006\u0000\u0003\u0000\u0001PZR.AI          PZR.BV          PZR.CI          PZR.AV          PZR.BI          PZR.CV          ANA1            ANA2            ANA3            DIG.stat1_01    DIG.stat1_02    DIG.stat1_03    DIG.stat1_04    DIG.stat1_05    DIG.stat1_06    DIG.stat1_07    DIG.stat1_08    DIG.stat1_09    DIG.stat1_10    DIG.stat1_11    DIG.stat1_12    DIG.stat1_13    DIG.stat1_14    DIG.stat1_15    DIG.stat1_16    \u0001\u0000\u0000\u0000\u0000\u0000\u0000\u0000\u0001\u0000\u0000\u0000\u0000\u0000\u0000\u0000\u0001\u0000\u0000\u0000\u0000\u0000\u0000\u0000\u0000\u0000\u0000\u0000\u0000\u0000\u0000\u0000\u0000\u0000\u0000\u0000ÿÿ\u0000\u0000\u0000\u0000\u0000\u0000", "PMU.098\u0000\u0000\u0000\u0000\u0000\u0000\u0000\u0000\u0000\u0000b\u0000\u000f\u0000\u0006\u0000\u0003\u0000\u0001PZR.AI          PZR.BV          PZR.CI          PZR.AV          PZR.BI          PZR.CV          ANA1            ANA2            ANA3            DIG.stat1_01    DIG.stat1_02    DIG.stat1_03    DIG.stat1_04    DIG.stat1_05    DIG.stat1_06    DIG.stat1_07    DIG.stat1_08    DIG.stat1_09    DIG.stat1_10    DIG.stat1_11    DIG.stat1_12    DIG.stat1_13    DIG.stat1_14    DIG.stat1_15    DIG.stat1_16    \u0001\u0000\u0000\u0000\u0000\u0000\u0000\u0000\u0001\u0000\u0000\u0000\u0000\u0000\u0000\u0000\u0001\u0000\u0000\u0000\u0000\u0000\u0000\u0000\u0000\u0000\u0000\u0000\u0000\u0000\u0000\u0000\u0000\u0000\u0000\u0000ÿÿ\u0000\u0000\u0000\u0000\u0000\u0000", "PMU.099\u0000\u0000\u0000\u0000\u0000\u0000\u0000\u0000\u0000\u0000c\u0000\u000f\u0000\u0006\u0000\u0003\u0000\u0001PZR.AI          PZR.BV          PZR.CI          PZR.AV          PZR.BI          PZR.CV          ANA1            ANA2            ANA3            DIG.stat1_01    DIG.stat1_02    DIG.stat1_03    DIG.stat1_04    DIG.stat1_05    DIG.stat1_06    DIG.stat1_07    DIG.stat1_08    DIG.stat1_09    DIG.stat1_10    DIG.stat1_11    DIG.stat1_12    DIG.stat1_13    DIG.stat1_14    DIG.stat1_15    DIG.stat1_16    \u0001\u0000\u0000\u0000\u0000\u0000\u0000\u0000\u0001\u0000\u0000\u0000\u0000\u0000\u0000\u0000\u0001\u0000\u0000\u0000\u0000\u0000\u0000\u0000\u0000\u0000\u0000\u0000\u0000\u0000\u0000\u0000\u0000\u0000\u0000\u0000ÿÿ\u0000\u0000\u0000\u0000\u0000\u0000", "PMU.100\u0000\u0000\u0000\u0000\u0000\u0000\u0000\u0000\u0000\u0000d\u0000\u000f\u0000\u0006\u0000\u0003\u0000\u0001PZR.AI          PZR.BV          PZR.CI          PZR.AV          PZR.BI          PZR.CV          ANA1            ANA2            ANA3            DIG.stat1_01    DIG.stat1_02    DIG.stat1_03    DIG.stat1_04    DIG.stat1_05    DIG.stat1_06    DIG.stat1_07    DIG.stat1_08    DIG.stat1_09    DIG.stat1_10    DIG.stat1_11    DIG.stat1_12    DIG.stat1_13    DIG.stat1_14    DIG.stat1_15    DIG.stat1_16    \u0001\u0000\u0000\u0000\u0000\u0000\u0000\u0000\u0001\u0000\u0000\u0000\u0000\u0000\u0000\u0000\u0001\u0000\u0000\u0000\u0000\u0000\u0000\u0000\u0000\u0000\u0000\u0000\u0000\u0000\u0000\u0000\u0000\u0000\u0000\u0000ÿÿ\u0000\u0000\u0000\u0000\u0000\u0000", "PMU.101\u0000\u0000\u0000\u0000\u0000\u0000\u0000\u0000\u0000\u0000e\u0000\u000f\u0000\u0006\u0000\u0003\u0000\u0001PZR.AI          PZR.BV          PZR.CI          PZR.AV          PZR.BI          PZR.CV          ANA1            ANA2            ANA3            DIG.stat1_01    DIG.stat1_02    DIG.stat1_03    DIG.stat1_04    DIG.stat1_05    DIG.stat1_06    DIG.stat1_07    DIG.stat1_08    DIG.stat1_09    DIG.stat1_10    DIG.stat1_11    DIG.stat1_12    DIG.stat1_13    DIG.stat1_14    DIG.stat1_15    DIG.stat1_16    \u0001\u0000\u0000\u0000\u0000\u0000\u0000\u0000\u0001\u0000\u0000\u0000\u0000\u0000\u0000\u0000\u0001\u0000\u0000\u0000\u0000\u0000\u0000\u0000\u0000\u0000\u0000\u0000\u0000\u0000\u0000\u0000\u0000\u0000\u0000\u0000ÿÿ\u0000\u0000\u0000\u0000\u0000\u0000", "PMU.102\u0000\u0000\u0000\u0000\u0000\u0000\u0000\u0000\u0000\u0000f\u0000\u000f\u0000\u0006\u0000\u0003\u0000\u0001PZR.AI          PZR.BV          PZR.CI          PZR.AV          PZR.BI          PZR.CV          ANA1            ANA2            ANA3            DIG.stat1_01    DIG.stat1_02    DIG.stat1_03    DIG.stat1_04    DIG.stat1_05    DIG.stat1_06    DIG.stat1_07    DIG.stat1_08    DIG.stat1_09    DIG.stat1_10    DIG.stat1_11    DIG.stat1_12    DIG.stat1_13    DIG.stat1_14    DIG.stat1_15    DIG.stat1_16    \u0001\u0000\u0000\u0000\u0000\u0000\u0000\u0000\u0001\u0000\u0000\u0000\u0000\u0000\u0000\u0000\u0001\u0000\u0000\u0000\u0000\u0000\u0000\u0000\u0000\u0000\u0000\u0000\u0000\u0000\u0000\u0000\u0000\u0000\u0000\u0000ÿÿ\u0000\u0000\u0000\u0000\u0000\u0000", "PMU.103\u0000\u0000\u0000\u0000\u0000\u0000\u0000\u0000\u0000\u0000g\u0000\u000f\u0000\u0006\u0000\u0003\u0000\u0001PZR.AI          PZR.BV          PZR.CI          PZR.AV          PZR.BI          PZR.CV          ANA1            ANA2            ANA3            DIG.stat1_01    DIG.stat1_02    DIG.stat1_03    DIG.stat1_04    DIG.stat1_05    DIG.stat1_06    DIG.stat1_07    DIG.stat1_08    DIG.stat1_09    DIG.stat1_10    DIG.stat1_11    DIG.stat1_12    DIG.stat1_13    DIG.stat1_14    DIG.stat1_15    DIG.stat1_16    \u0001\u0000\u0000\u0000\u0000\u0000\u0000\u0000\u0001\u0000\u0000\u0000\u0000\u0000\u0000\u0000\u0001\u0000\u0000\u0000\u0000\u0000\u0000\u0000\u0000\u0000\u0000\u0000\u0000\u0000\u0000\u0000\u0000\u0000\u0000\u0000ÿÿ\u0000\u0000\u0000\u0000\u0000\u0000", "PMU.104\u0000\u0000\u0000\u0000\u0000\u0000\u0000\u0000\u0000\u0000h\u0000\u000f\u0000\u0006\u0000\u0003\u0000\u0001PZR.AI          PZR.BV          PZR.CI          PZR.AV          PZR.BI          PZR.CV          ANA1            ANA2            ANA3            DIG.stat1_01    DIG.stat1_02    DIG.stat1_03    DIG.stat1_04    DIG.stat1_05    DIG.stat1_06    DIG.stat1_07    DIG.stat1_08    DIG.stat1_09    DIG.stat1_10    DIG.stat1_11    DIG.stat1_12    DIG.stat1_13    DIG.stat1_14    DIG.stat1_15    DIG.stat1_16    \u0001\u0000\u0000\u0000\u0000\u0000\u0000\u0000\u0001\u0000\u0000\u0000\u0000\u0000\u0000\u0000\u0001\u0000\u0000\u0000\u0000\u0000\u0000\u0000\u0000\u0000\u0000\u0000\u0000\u0000\u0000\u0000\u0000\u0000\u0000\u0000ÿÿ\u0000\u0000\u0000\u0000\u0000\u0000", "PMU.105\u0000\u0000\u0000\u0000\u0000\u0000\u0000\u0000\u0000\u0000i\u0000\u000f\u0000\u0006\u0000\u0003\u0000\u0001PZR.AI          PZR.BV          PZR.CI          PZR.AV          PZR.BI          PZR.CV          ANA1            ANA2            ANA3            DIG.stat1_01    DIG.stat1_02    DIG.stat1_03    DIG.stat1_04    DIG.stat1_05    DIG.stat1_06    DIG.stat1_07    DIG.stat1_08    DIG.stat1_09    DIG.stat1_10    DIG.stat1_11    DIG.stat1_12    DIG.stat1_13    DIG.stat1_14    DIG.stat1_15    DIG.stat1_16    \u0001\u0000\u0000\u0000\u0000\u0000\u0000\u0000\u0001\u0000\u0000\u0000\u0000\u0000\u0000\u0000\u0001\u0000\u0000\u0000\u0000\u0000\u0000\u0000\u0000\u0000\u0000\u0000\u0000\u0000\u0000\u0000\u0000\u0000\u0000\u0000ÿÿ\u0000\u0000\u0000\u0000\u0000\u0000", "PMU.106\u0000\u0000\u0000\u0000\u0000\u0000\u0000\u0000\u0000\u0000j\u0000\u000f\u0000\u0006\u0000\u0003\u0000\u0001PZR.AI          PZR.BV          PZR.CI          PZR.AV          PZR.BI          PZR.CV          ANA1            ANA2            ANA3            DIG.stat1_01    DIG.stat1_02    DIG.stat1_03    DIG.stat1_04    DIG.stat1_05    DIG.stat1_06    DIG.stat1_07    DIG.stat1_08    DIG.stat1_09    DIG.stat1_10    DIG.stat1_11    DIG.stat1_12    DIG.stat1_13    DIG.stat1_14    DIG.stat1_15    DIG.stat1_16    \u0001\u0000\u0000\u0000\u0000\u0000\u0000\u0000\u0001\u0000\u0000\u0000\u0000\u0000\u0000\u0000\u0001\u0000\u0000\u0000\u0000\u0000\u0000\u0000\u0000\u0000\u0000\u0000\u0000\u0000\u0000\u0000\u0000\u0000\u0000\u0000ÿÿ\u0000\u0000\u0000\u0000\u0000\u0000", "PMU.107\u0000\u0000\u0000\u0000\u0000\u0000\u0000\u0000\u0000\u0000k\u0000\u000f\u0000\u0006\u0000\u0003\u0000\u0001PZR.AI          PZR.BV          PZR.CI          PZR.AV          PZR.BI          PZR.CV          ANA1            ANA2            ANA3            DIG.stat1_01    DIG.stat1_02    DIG.stat1_03    DIG.stat1_04    DIG.stat1_05    DIG.stat1_06    DIG.stat1_07    DIG.stat1_08    DIG.stat1_09    DIG.stat1_10    DIG.stat1_11    DIG.stat1_12    DIG.stat1_13    DIG.stat1_14    DIG.stat1_15    DIG.stat1_16    \u0001\u0000\u0000\u0000\u0000\u0000\u0000\u0000\u0001\u0000\u0000\u0000\u0000\u0000\u0000\u0000\u0001\u0000\u0000\u0000\u0000\u0000\u0000\u0000\u0000\u0000\u0000\u0000\u0000\u0000\u0000\u0000\u0000\u0000\u0000\u0000ÿÿ\u0000\u0000\u0000\u0000\u0000\u0000", "PMU.108\u0000\u0000\u0000\u0000\u0000\u0000\u0000\u0000\u0000\u0000l\u0000\u000f\u0000\u0006\u0000\u0003\u0000\u0001PZR.AI          PZR.BV          PZR.CI          PZR.AV          PZR.BI          PZR.CV          ANA1            ANA2            ANA3            DIG.stat1_01    DIG.stat1_02    DIG.stat1_03    DIG.stat1_04    DIG.stat1_05    DIG.stat1_06    DIG.stat1_07    DIG.stat1_08    DIG.stat1_09    DIG.stat1_10    DIG.stat1_11    DIG.stat1_12    DIG.stat1_13    DIG.stat1_14    DIG.stat1_15    DIG.stat1_16    \u0001\u0000\u0000\u0000\u0000\u0000\u0000\u0000\u0001\u0000\u0000\u0000\u0000\u0000\u0000\u0000\u0001\u0000\u0000\u0000\u0000\u0000\u0000\u0000\u0000\u0000\u0000\u0000\u0000\u0000\u0000\u0000\u0000\u0000\u0000\u0000ÿÿ\u0000\u0000\u0000\u0000\u0000\u0000", "PMU.109\u0000\u0000\u0000\u0000\u0000\u0000\u0000\u0000\u0000\u0000m\u0000\u000f\u0000\u0006\u0000\u0003\u0000\u0001PZR.AI          PZR.BV          PZR.CI          PZR.AV          PZR.BI          PZR.CV          ANA1            ANA2            ANA3            DIG.stat1_01    DIG.stat1_02    DIG.stat1_03    DIG.stat1_04    DIG.stat1_05    DIG.stat1_06    DIG.stat1_07    DIG.stat1_08    DIG.stat1_09    DIG.stat1_10    DIG.stat1_11    DIG.stat1_12    DIG.stat1_13    DIG.stat1_14    DIG.stat1_15    DIG.stat1_16    \u0001\u0000\u0000\u0000\u0000\u0000\u0000\u0000\u0001\u0000\u0000\u0000\u0000\u0000\u0000\u0000\u0001\u0000\u0000\u0000\u0000\u0000\u0000\u0000\u0000\u0000\u0000\u0000\u0000\u0000\u0000\u0000\u0000\u0000\u0000\u0000ÿÿ\u0000\u0000\u0000\u0000\u0000\u0000", "PMU.110\u0000\u0000\u0000\u0000\u0000\u0000\u0000\u0000\u0000\u0000n\u0000\u000f\u0000\u0006\u0000\u0003\u0000\u0001PZR.AI          PZR.BV          PZR.CI          PZR.AV          PZR.BI          PZR.CV          ANA1            ANA2            ANA3            DIG.stat1_01    DIG.stat1_02    DIG.stat1_03    DIG.stat1_04    DIG.stat1_05    DIG.stat1_06    DIG.stat1_07    DIG.stat1_08    DIG.stat1_09    DIG.stat1_10    DIG.stat1_11    DIG.stat1_12    DIG.stat1_13    DIG.stat1_14    DIG.stat1_15    DIG.stat1_16    \u0001\u0000\u0000\u0000\u0000\u0000\u0000\u0000\u0001\u0000\u0000\u0000\u0000\u0000\u0000\u0000\u0001\u0000\u0000\u0000\u0000\u0000\u0000\u0000\u0000\u0000\u0000\u0000\u0000\u0000\u0000\u0000\u0000\u0000\u0000\u0000ÿÿ\u0000\u0000\u0000\u0000\u0000\u0000", "PMU.111\u0000\u0000\u0000\u0000\u0000\u0000\u0000\u0000\u0000\u0000o\u0000\u000f\u0000\u0006\u0000\u0003\u0000\u0001PZR.AI          PZR.BV          PZR.CI          PZR.AV          PZR.BI          PZR.CV          ANA1            ANA2            ANA3            DIG.stat1_01    DIG.stat1_02    DIG.stat1_03    DIG.stat1_04    DIG.stat1_05    DIG.stat1_06    DIG.stat1_07    DIG.stat1_08    DIG.stat1_09    DIG.stat1_10    DIG.stat1_11    DIG.stat1_12    DIG.stat1_13    DIG.stat1_14    DIG.stat1_15    DIG.stat1_16    \u0001\u0000\u0000\u0000\u0000\u0000\u0000\u0000\u0001\u0000\u0000\u0000\u0000\u0000\u0000\u0000\u0001\u0000\u0000\u0000\u0000\u0000\u0000\u0000\u0000\u0000\u0000\u0000\u0000\u0000\u0000\u0000\u0000\u0000\u0000\u0000ÿÿ\u0000\u0000\u0000\u0000\u0000\u0000", "PMU.112\u0000\u0000\u0000\u0000\u0000\u0000\u0000\u0000\u0000\u0000p\u0000\u000f\u0000\u0006\u0000\u0003\u0000\u0001PZR.AI          PZR.BV          PZR.CI          PZR.AV          PZR.BI          PZR.CV          ANA1            ANA2            ANA3            DIG.stat1_01    DIG.stat1_02    DIG.stat1_03    DIG.stat1_04    DIG.stat1_05    DIG.stat1_06    DIG.stat1_07    DIG.stat1_08    DIG.stat1_09    DIG.stat1_10    DIG.stat1_11    DIG.stat1_12    DIG.stat1_13    DIG.stat1_14    DIG.stat1_15    DIG.stat1_16    \u0001\u0000\u0000\u0000\u0000\u0000\u0000\u0000\u0001\u0000\u0000\u0000\u0000\u0000\u0000\u0000\u0001\u0000\u0000\u0000\u0000\u0000\u0000\u0000\u0000\u0000\u0000\u0000\u0000\u0000\u0000\u0000\u0000\u0000\u0000\u0000ÿÿ\u0000\u0000\u0000\u0000\u0000\u0000", "PMU.113\u0000\u0000\u0000\u0000\u0000\u0000\u0000\u0000\u0000\u0000q\u0000\u000f\u0000\u0006\u0000\u0003\u0000\u0001PZR.AI          PZR.BV          PZR.CI          PZR.AV          PZR.BI          PZR.CV          ANA1            ANA2            ANA3            DIG.stat1_01    DIG.stat1_02    DIG.stat1_03    DIG.stat1_04    DIG.stat1_05    DIG.stat1_06    DIG.stat1_07    DIG.stat1_08    DIG.stat1_09    DIG.stat1_10    DIG.stat1_11    DIG.stat1_12    DIG.stat1_13    DIG.stat1_14    DIG.stat1_15    DIG.stat1_16    \u0001\u0000\u0000\u0000\u0000\u0000\u0000\u0000\u0001\u0000\u0000\u0000\u0000\u0000\u0000\u0000\u0001\u0000\u0000\u0000\u0000\u0000\u0000\u0000\u0000\u0000\u0000\u0000\u0000\u0000\u0000\u0000\u0000\u0000\u0000\u0000ÿÿ\u0000\u0000\u0000\u0000\u0000\u0000", "PMU.114\u0000\u0000\u0000\u0000\u0000\u0000\u0000\u0000\u0000\u0000r\u0000\u000f\u0000\u0006\u0000\u0003\u0000\u0001PZR.AI          PZR.BV          PZR.CI          PZR.AV          PZR.BI          PZR.CV          ANA1            ANA2            ANA3            DIG.stat1_01    DIG.stat1_02    DIG.stat1_03    DIG.stat1_04    DIG.stat1_05    DIG.stat1_06    DIG.stat1_07    DIG.stat1_08    DIG.stat1_09    DIG.stat1_10    DIG.stat1_11    DIG.stat1_12    DIG.stat1_13    DIG.stat1_14    DIG.stat1_15    DIG.stat1_16    \u0001\u0000\u0000\u0000\u0000\u0000\u0000\u0000\u0001\u0000\u0000\u0000\u0000\u0000\u0000\u0000\u0001\u0000\u0000\u0000\u0000\u0000\u0000\u0000\u0000\u0000\u0000\u0000\u0000\u0000\u0000\u0000\u0000\u0000\u0000\u0000ÿÿ\u0000\u0000\u0000\u0000\u0000\u0000", "PMU.115\u0000\u0000\u0000\u0000\u0000\u0000\u0000\u0000\u0000\u0000s\u0000\u000f\u0000\u0006\u0000\u0003\u0000\u0001PZR.AI          PZR.BV          PZR.CI          PZR.AV          PZR.BI          PZR.CV          ANA1            ANA2            ANA3            DIG.stat1_01    DIG.stat1_02    DIG.stat1_03    DIG.stat1_04    DIG.stat1_05    DIG.stat1_06    DIG.stat1_07    DIG.stat1_08    DIG.stat1_09    DIG.stat1_10    DIG.stat1_11    DIG.stat1_12    DIG.stat1_13    DIG.stat1_14    DIG.stat1_15    DIG.stat1_16    \u0001\u0000\u0000\u0000\u0000\u0000\u0000\u0000\u0001\u0000\u0000\u0000\u0000\u0000\u0000\u0000\u0001\u0000\u0000\u0000\u0000\u0000\u0000\u0000\u0000\u0000\u0000\u0000\u0000\u0000\u0000\u0000\u0000\u0000\u0000\u0000ÿÿ\u0000\u0000\u0000\u0000\u0000\u0000", "PMU.116\u0000\u0000\u0000\u0000\u0000\u0000\u0000\u0000\u0000\u0000t\u0000\u000f\u0000\u0006\u0000\u0003\u0000\u0001PZR.AI          PZR.BV          PZR.CI          PZR.AV          PZR.BI          PZR.CV          ANA1            ANA2            ANA3            DIG.stat1_01    DIG.stat1_02    DIG.stat1_03    DIG.stat1_04    DIG.stat1_05    DIG.stat1_06    DIG.stat1_07    DIG.stat1_08    DIG.stat1_09    DIG.stat1_10    DIG.stat1_11    DIG.stat1_12    DIG.stat1_13    DIG.stat1_14    DIG.stat1_15    DIG.stat1_16    \u0001\u0000\u0000\u0000\u0000\u0000\u0000\u0000\u0001\u0000\u0000\u0000\u0000\u0000\u0000\u0000\u0001\u0000\u0000\u0000\u0000\u0000\u0000\u0000\u0000\u0000\u0000\u0000\u0000\u0000\u0000\u0000\u0000\u0000\u0000\u0000ÿÿ\u0000\u0000\u0000\u0000\u0000\u0000", "PMU.117\u0000\u0000\u0000\u0000\u0000\u0000\u0000\u0000\u0000\u0000u\u0000\u000f\u0000\u0006\u0000\u0003\u0000\u0001PZR.AI          PZR.BV          PZR.CI          PZR.AV          PZR.BI          PZR.CV          ANA1            ANA2            ANA3            DIG.stat1_01    DIG.stat1_02    DIG.stat1_03    DIG.stat1_04    DIG.stat1_05    DIG.stat1_06    DIG.stat1_07    DIG.stat1_08    DIG.stat1_09    DIG.stat1_10    DIG.stat1_11    DIG.stat1_12    DIG.stat1_13    DIG.stat1_14    DIG.stat1_15    DIG.stat1_16    \u0001\u0000\u0000\u0000\u0000\u0000\u0000\u0000\u0001\u0000\u0000\u0000\u0000\u0000\u0000\u0000\u0001\u0000\u0000\u0000\u0000\u0000\u0000\u0000\u0000\u0000\u0000\u0000\u0000\u0000\u0000\u0000\u0000\u0000\u0000\u0000ÿÿ\u0000\u0000\u0000\u0000\u0000\u0000", "PMU.118\u0000\u0000\u0000\u0000\u0000\u0000\u0000\u0000\u0000\u0000v\u0000\u000f\u0000\u0006\u0000\u0003\u0000\u0001PZR.AI          PZR.BV          PZR.CI          PZR.AV          PZR.BI          PZR.CV          ANA1            ANA2            ANA3            DIG.stat1_01    DIG.stat1_02    DIG.stat1_03    DIG.stat1_04    DIG.stat1_05    DIG.stat1_06    DIG.stat1_07    DIG.stat1_08    DIG.stat1_09    DIG.stat1_10    DIG.stat1_11    DIG.stat1_12    DIG.stat1_13    DIG.stat1_14    DIG.stat1_15    DIG.stat1_16    \u0001\u0000\u0000\u0000\u0000\u0000\u0000\u0000\u0001\u0000\u0000\u0000\u0000\u0000\u0000\u0000\u0001\u0000\u0000\u0000\u0000\u0000\u0000\u0000\u0000\u0000\u0000\u0000\u0000\u0000\u0000\u0000\u0000\u0000\u0000\u0000ÿÿ\u0000\u0000\u0000\u0000\u0000\u0000", "PMU.119\u0000\u0000\u0000\u0000\u0000\u0000\u0000\u0000\u0000\u0000w\u0000\u000f\u0000\u0006\u0000\u0003\u0000\u0001PZR.AI          PZR.BV          PZR.CI          PZR.AV          PZR.BI          PZR.CV          ANA1            ANA2            ANA3            DIG.stat1_01    DIG.stat1_02    DIG.stat1_03    DIG.stat1_04    DIG.stat1_05    DIG.stat1_06    DIG.stat1_07    DIG.stat1_08    DIG.stat1_09    DIG.stat1_10    DIG.stat1_11    DIG.stat1_12    DIG.stat1_13    DIG.stat1_14    DIG.stat1_15    DIG.stat1_16    \u0001\u0000\u0000\u0000\u0000\u0000\u0000\u0000\u0001\u0000\u0000\u0000\u0000\u0000\u0000\u0000\u0001\u0000\u0000\u0000\u0000\u0000\u0000\u0000\u0000\u0000\u0000\u0000\u0000\u0000\u0000\u0000\u0000\u0000\u0000\u0000ÿÿ\u0000\u0000\u0000\u0000\u0000\u0000", "PMU.120\u0000\u0000\u0000\u0000\u0000\u0000\u0000\u0000\u0000\u0000x\u0000\u000f\u0000\u0006\u0000\u0003\u0000\u0001PZR.AI          PZR.BV          PZR.CI          PZR.AV          PZR.BI          PZR.CV          ANA1            ANA2            ANA3            DIG.stat1_01    DIG.stat1_02    DIG.stat1_03    DIG.stat1_04    DIG.stat1_05    DIG.stat1_06    DIG.stat1_07    DIG.stat1_08    DIG.stat1_09    DIG.stat1_10    DIG.stat1_11    DIG.stat1_12    DIG.stat1_13    DIG.stat1_14    DIG.stat1_15    DIG.stat1_16    \u0001\u0000\u0000\u0000\u0000\u0000\u0000\u0000\u0001\u0000\u0000\u0000\u0000\u0000\u0000\u0000\u0001\u0000\u0000\u0000\u0000\u0000\u0000\u0000\u0000\u0000\u0000\u0000\u0000\u0000\u0000\u0000\u0000\u0000\u0000\u0000ÿÿ\u0000\u0000\u0000\u0000\u0000\u0000", "PMU.121\u0000\u0000\u0000\u0000\u0000\u0000\u0000\u0000\u0000\u0000y\u0000\u000f\u0000\u0006\u0000\u0003\u0000\u0001PZR.AI          PZR.BV          PZR.CI          PZR.AV          PZR.BI          PZR.CV          ANA1            ANA2            ANA3            DIG.stat1_01    DIG.stat1_02    DIG.stat1_03    DIG.stat1_04    DIG.stat1_05    DIG.stat1_06    DIG.stat1_07    DIG.stat1_08    DIG.stat1_09    DIG.stat1_10    DIG.stat1_11    DIG.stat1_12    DIG.stat1_13    DIG.stat1_14    DIG.stat1_15    DIG.stat1_16    \u0001\u0000\u0000\u0000\u0000\u0000\u0000\u0000\u0001\u0000\u0000\u0000\u0000\u0000\u0000\u0000\u0001\u0000\u0000\u0000\u0000\u0000\u0000\u0000\u0000\u0000\u0000\u0000\u0000\u0000\u0000\u0000\u0000\u0000\u0000\u0000ÿÿ\u0000\u0000\u0000\u0000\u0000\u0000", "PMU.122\u0000\u0000\u0000\u0000\u0000\u0000\u0000\u0000\u0000\u0000z\u0000\u000f\u0000\u0006\u0000\u0003\u0000\u0001PZR.AI          PZR.BV          PZR.CI          PZR.AV          PZR.BI          PZR.CV          ANA1            ANA2            ANA3            DIG.stat1_01    DIG.stat1_02    DIG.stat1_03    DIG.stat1_04    DIG.stat1_05    DIG.stat1_06    DIG.stat1_07    DIG.stat1_08    DIG.stat1_09    DIG.stat1_10    DIG.stat1_11    DIG.stat1_12    DIG.stat1_13    DIG.stat1_14    DIG.stat1_15    DIG.stat1_16    \u0001\u0000\u0000\u0000\u0000\u0000\u0000\u0000\u0001\u0000\u0000\u0000\u0000\u0000\u0000\u0000\u0001\u0000\u0000\u0000\u0000\u0000\u0000\u0000\u0000\u0000\u0000\u0000\u0000\u0000\u0000\u0000\u0000\u0000\u0000\u0000ÿÿ\u0000\u0000\u0000\u0000\u0000\u0000", "PMU.123\u0000\u0000\u0000\u0000\u0000\u0000\u0000\u0000\u0000\u0000{\u0000\u000f\u0000\u0006\u0000\u0003\u0000\u0001PZR.AI          PZR.BV          PZR.CI          PZR.AV          PZR.BI          PZR.CV          ANA1            ANA2            ANA3            DIG.stat1_01    DIG.stat1_02    DIG.stat1_03    DIG.stat1_04    DIG.stat1_05    DIG.stat1_06    DIG.stat1_07    DIG.stat1_08    DIG.stat1_09    DIG.stat1_10    DIG.stat1_11    DIG.stat1_12    DIG.stat1_13    DIG.stat1_14    DIG.stat1_15    DIG.stat1_16    \u0001\u0000\u0000\u0000\u0000\u0000\u0000\u0000\u0001\u0000\u0000\u0000\u0000\u0000\u0000\u0000\u0001\u0000\u0000\u0000\u0000\u0000\u0000\u0000\u0000\u0000\u0000\u0000\u0000\u0000\u0000\u0000\u0000\u0000\u0000\u0000ÿÿ\u0000\u0000\u0000\u0000\u0000\u0000", "PMU.124\u0000\u0000\u0000\u0000\u0000\u0000\u0000\u0000\u0000\u0000|\u0000\u000f\u0000\u0006\u0000\u0003\u0000\u0001PZR.AI          PZR.BV          PZR.CI          PZR.AV          PZR.BI          PZR.CV          ANA1            ANA2            ANA3            DIG.stat1_01    DIG.stat1_02    DIG.stat1_03    DIG.stat1_04    DIG.stat1_05    DIG.stat1_06    DIG.stat1_07    DIG.stat1_08    DIG.stat1_09    DIG.stat1_10    DIG.stat1_11    DIG.stat1_12    DIG.stat1_13    DIG.stat1_14    DIG.stat1_15    DIG.stat1_16    \u0001\u0000\u0000\u0000\u0000\u0000\u0000\u0000\u0001\u0000\u0000\u0000\u0000\u0000\u0000\u0000\u0001\u0000\u0000\u0000\u0000\u0000\u0000\u0000\u0000\u0000\u0000\u0000\u0000\u0000\u0000\u0000\u0000\u0000\u0000\u0000ÿÿ\u0000\u0000\u0000\u0000\u0000\u0000", "PMU.125\u0000\u0000\u0000\u0000\u0000\u0000\u0000\u0000\u0000\u0000}\u0000\u000f\u0000\u0006\u0000\u0003\u0000\u0001PZR.AI          PZR.BV          PZR.CI          PZR.AV          PZR.BI          PZR.CV          ANA1            ANA2            ANA3            DIG.stat1_01    DIG.stat1_02    DIG.stat1_03    DIG.stat1_04    DIG.stat1_05    DIG.stat1_06    DIG.stat1_07    DIG.stat1_08    DIG.stat1_09    DIG.stat1_10    DIG.stat1_11    DIG.stat1_12    DIG.stat1_13    DIG.stat1_14    DIG.stat1_15    DIG.stat1_16    \u0001\u0000\u0000\u0000\u0000\u0000\u0000\u0000\u0001\u0000\u0000\u0000\u0000\u0000\u0000\u0000\u0001\u0000\u0000\u0000\u0000\u0000\u0000\u0000\u0000\u0000\u0000\u0000\u0000\u0000\u0000\u0000\u0000\u0000\u0000\u0000ÿÿ\u0000\u0000\u0000\u0000\u0000\u0000", "PMU.126\u0000\u0000\u0000\u0000\u0000\u0000\u0000\u0000\u0000\u0000~\u0000\u000f\u0000\u0006\u0000\u0003\u0000\u0001PZR.AI          PZR.BV          PZR.CI          PZR.AV          PZR.BI          PZR.CV          ANA1            ANA2            ANA3            DIG.stat1_01    DIG.stat1_02    DIG.stat1_03    DIG.stat1_04    DIG.stat1_05    DIG.stat1_06    DIG.stat1_07    DIG.stat1_08    DIG.stat1_09    DIG.stat1_10    DIG.stat1_11    DIG.stat1_12    DIG.stat1_13    DIG.stat1_14    DIG.stat1_15    DIG.stat1_16    \u0001\u0000\u0000\u0000\u0000\u0000\u0000\u0000\u0001\u0000\u0000\u0000\u0000\u0000\u0000\u0000\u0001\u0000\u0000\u0000\u0000\u0000\u0000\u0000\u0000\u0000\u0000\u0000\u0000\u0000\u0000\u0000\u0000\u0000\u0000\u0000ÿÿ\u0000\u0000\u0000\u0000\u0000\u0000", "PMU.127\u0000\u0000\u0000\u0000\u0000\u0000\u0000\u0000\u0000\u0000\u0000\u000f\u0000\u0006\u0000\u0003\u0000\u0001PZR.AI          PZR.BV          PZR.CI          PZR.AV          PZR.BI          PZR.CV          ANA1            ANA2            ANA3            DIG.stat1_01    DIG.stat1_02    DIG.stat1_03    DIG.stat1_04    DIG.stat1_05    DIG.stat1_06    DIG.stat1_07    DIG.stat1_08    DIG.stat1_09    DIG.stat1_10    DIG.stat1_11    DIG.stat1_12    DIG.stat1_13    DIG.stat1_14    DIG.stat1_15    DIG.stat1_16    \u0001\u0000\u0000\u0000\u0000\u0000\u0000\u0000\u0001\u0000\u0000\u0000\u0000\u0000\u0000\u0000\u0001\u0000\u0000\u0000\u0000\u0000\u0000\u0000\u0000\u0000\u0000\u0000\u0000\u0000\u0000\u0000\u0000\u0000\u0000\u0000ÿÿ\u0000\u0000\u0000\u0000\u0000\u0000", "PMU.128\u0000\u0000\u0000\u0000\u0000\u0000\u0000\u0000\u0000\u0000€\u0000\u000f\u0000\u0006\u0000\u0003\u0000\u0001PZR.AI          PZR.BV          PZR.CI          PZR.AV          PZR.BI          PZR.CV          ANA1            ANA2            ANA3            DIG.stat1_01    DIG.stat1_02    DIG.stat1_03    DIG.stat1_04    DIG.stat1_05    DIG.stat1_06    DIG.stat1_07    DIG.stat1_08    DIG.stat1_09    DIG.stat1_10    DIG.stat1_11    DIG.stat1_12    DIG.stat1_13    DIG.stat1_14    DIG.stat1_15    DIG.stat1_16    \u0001\u0000\u0000\u0000\u0000\u0000\u0000\u0000\u0001\u0000\u0000\u0000\u0000\u0000\u0000\u0000\u0001\u0000\u0000\u0000\u0000\u0000\u0000\u0000\u0000\u0000\u0000\u0000\u0000\u0000\u0000\u0000\u0000\u0000\u0000\u0000ÿÿ\u0000\u0000\u0000\u0000\u0000\u0000", "PMU.129\u0000\u0000\u0000\u0000\u0000\u0000\u0000\u0000\u0000\u0000\u0000\u000f\u0000\u0006\u0000\u0003\u0000\u0001PZR.AI          PZR.BV          PZR.CI          PZR.AV          PZR.BI          PZR.CV          ANA1            ANA2            ANA3            DIG.stat1_01    DIG.stat1_02    DIG.stat1_03    DIG.stat1_04    DIG.stat1_05    DIG.stat1_06    DIG.stat1_07    DIG.stat1_08    DIG.stat1_09    DIG.stat1_10    DIG.stat1_11    DIG.stat1_12    DIG.stat1_13    DIG.stat1_14    DIG.stat1_15    DIG.stat1_16    \u0001\u0000\u0000\u0000\u0000\u0000\u0000\u0000\u0001\u0000\u0000\u0000\u0000\u0000\u0000\u0000\u0001\u0000\u0000\u0000\u0000\u0000\u0000\u0000\u0000\u0000\u0000\u0000\u0000\u0000\u0000\u0000\u0000\u0000\u0000\u0000ÿÿ\u0000\u0000\u0000\u0000\u0000\u0000", "PMU.130\u0000\u0000\u0000\u0000\u0000\u0000\u0000\u0000\u0000\u0000‚\u0000\u000f\u0000\u0006\u0000\u0003\u0000\u0001PZR.AI          PZR.BV          PZR.CI          PZR.AV          PZR.BI          PZR.CV          ANA1            ANA2            ANA3            DIG.stat1_01    DIG.stat1_02    DIG.stat1_03    DIG.stat1_04    DIG.stat1_05    DIG.stat1_06    DIG.stat1_07    DIG.stat1_08    DIG.stat1_09    DIG.stat1_10    DIG.stat1_11    DIG.stat1_12    DIG.stat1_13    DIG.stat1_14    DIG.stat1_15    DIG.stat1_16    \u0001\u0000\u0000\u0000\u0000\u0000\u0000\u0000\u0001\u0000\u0000\u0000\u0000\u0000\u0000\u0000\u0001\u0000\u0000\u0000\u0000\u0000\u0000\u0000\u0000\u0000\u0000\u0000\u0000\u0000\u0000\u0000\u0000\u0000\u0000\u0000ÿÿ\u0000\u0000\u0000\u0000\u0000\u0000", "PMU.131\u0000\u0000\u0000\u0000\u0000\u0000\u0000\u0000\u0000\u0000ƒ\u0000\u000f\u0000\u0006\u0000\u0003\u0000\u0001PZR.AI          PZR.BV          PZR.CI          PZR.AV          PZR.BI          PZR.CV          ANA1            ANA2            ANA3            DIG.stat1_01    DIG.stat1_02    DIG.stat1_03    DIG.stat1_04    DIG.stat1_05    DIG.stat1_06    DIG.stat1_07    DIG.stat1_08    DIG.stat1_09    DIG.stat1_10    DIG.stat1_11    DIG.stat1_12    DIG.stat1_13    DIG.stat1_14    DIG.stat1_15    DIG.stat1_16    \u0001\u0000\u0000\u0000\u0000\u0000\u0000\u0000\u0001\u0000\u0000\u0000\u0000\u0000\u0000\u0000\u0001\u0000\u0000\u0000\u0000\u0000\u0000\u0000\u0000\u0000\u0000\u0000\u0000\u0000\u0000\u0000\u0000\u0000\u0000\u0000ÿÿ\u0000\u0000\u0000\u0000\u0000\u0000", "PMU.132\u0000\u0000\u0000\u0000\u0000\u0000\u0000\u0000\u0000\u0000„\u0000\u000f\u0000\u0006\u0000\u0003\u0000\u0001PZR.AI          PZR.BV          PZR.CI          PZR.AV          PZR.BI          PZR.CV          ANA1            ANA2            ANA3            DIG.stat1_01    DIG.stat1_02    DIG.stat1_03    DIG.stat1_04    DIG.stat1_05    DIG.stat1_06    DIG.stat1_07    DIG.stat1_08    DIG.stat1_09    DIG.stat1_10    DIG.stat1_11    DIG.stat1_12    DIG.stat1_13    DIG.stat1_14    DIG.stat1_15    DIG.stat1_16    \u0001\u0000\u0000\u0000\u0000\u0000\u0000\u0000\u0001\u0000\u0000\u0000\u0000\u0000\u0000\u0000\u0001\u0000\u0000\u0000\u0000\u0000\u0000\u0000\u0000\u0000\u0000\u0000\u0000\u0000\u0000\u0000\u0000\u0000\u0000\u0000ÿÿ\u0000\u0000\u0000\u0000\u0000\u0000", "PMU.133\u0000\u0000\u0000\u0000\u0000\u0000\u0000\u0000\u0000\u0000…\u0000\u000f\u0000\u0006\u0000\u0003\u0000\u0001PZR.AI          PZR.BV          PZR.CI          PZR.AV          PZR.BI          PZR.CV          ANA1            ANA2            ANA3            DIG.stat1_01    DIG.stat1_02    DIG.stat1_03    DIG.stat1_04    DIG.stat1_05    DIG.stat1_06    DIG.stat1_07    DIG.stat1_08    DIG.stat1_09    DIG.stat1_10    DIG.stat1_11    DIG.stat1_12    DIG.stat1_13    DIG.stat1_14    DIG.stat1_15    DIG.stat1_16    \u0001\u0000\u0000\u0000\u0000\u0000\u0000\u0000\u0001\u0000\u0000\u0000\u0000\u0000\u0000\u0000\u0001\u0000\u0000\u0000\u0000\u0000\u0000\u0000\u0000\u0000\u0000\u0000\u0000\u0000\u0000\u0000\u0000\u0000\u0000\u0000ÿÿ\u0000\u0000\u0000\u0000\u0000\u0000", "PMU.134\u0000\u0000\u0000\u0000\u0000\u0000\u0000\u0000\u0000\u0000†\u0000\u000f\u0000\u0006\u0000\u0003\u0000\u0001PZR.AI          PZR.BV          PZR.CI          PZR.AV          PZR.BI          PZR.CV          ANA1            ANA2            ANA3            DIG.stat1_01    DIG.stat1_02    DIG.stat1_03    DIG.stat1_04    DIG.stat1_05    DIG.stat1_06    DIG.stat1_07    DIG.stat1_08    DIG.stat1_09    DIG.stat1_10    DIG.stat1_11    DIG.stat1_12    DIG.stat1_13    DIG.stat1_14    DIG.stat1_15    DIG.stat1_16    \u0001\u0000\u0000\u0000\u0000\u0000\u0000\u0000\u0001\u0000\u0000\u0000\u0000\u0000\u0000\u0000\u0001\u0000\u0000\u0000\u0000\u0000\u0000\u0000\u0000\u0000\u0000\u0000\u0000\u0000\u0000\u0000\u0000\u0000\u0000\u0000ÿÿ\u0000\u0000\u0000\u0000\u0000\u0000", "PMU.135\u0000\u0000\u0000\u0000\u0000\u0000\u0000\u0000\u0000\u0000‡\u0000\u000f\u0000\u0006\u0000\u0003\u0000\u0001PZR.AI          PZR.BV          PZR.CI          PZR.AV          PZR.BI          PZR.CV          ANA1            ANA2            ANA3            DIG.stat1_01    DIG.stat1_02    DIG.stat1_03    DIG.stat1_04    DIG.stat1_05    DIG.stat1_06    DIG.stat1_07    DIG.stat1_08    DIG.stat1_09    DIG.stat1_10    DIG.stat1_11    DIG.stat1_12    DIG.stat1_13    DIG.stat1_14    DIG.stat1_15    DIG.stat1_16    \u0001\u0000\u0000\u0000\u0000\u0000\u0000\u0000\u0001\u0000\u0000\u0000\u0000\u0000\u0000\u0000\u0001\u0000\u0000\u0000\u0000\u0000\u0000\u0000\u0000\u0000\u0000\u0000\u0000\u0000\u0000\u0000\u0000\u0000\u0000\u0000ÿÿ\u0000\u0000\u0000\u0000\u0000\u0000", "PMU.136\u0000\u0000\u0000\u0000\u0000\u0000\u0000\u0000\u0000\u0000ˆ\u0000\u000f\u0000\u0006\u0000\u0003\u0000\u0001PZR.AI          PZR.BV          PZR.CI          PZR.AV          PZR.BI          PZR.CV          ANA1            ANA2            ANA3            DIG.stat1_01    DIG.stat1_02    DIG.stat1_03    DIG.stat1_04    DIG.stat1_05    DIG.stat1_06    DIG.stat1_07    DIG.stat1_08    DIG.stat1_09    DIG.stat1_10    DIG.stat1_11    DIG.stat1_12    DIG.stat1_13    DIG.stat1_14    DIG.stat1_15    DIG.stat1_16    \u0001\u0000\u0000\u0000\u0000\u0000\u0000\u0000\u0001\u0000\u0000\u0000\u0000\u0000\u0000\u0000\u0001\u0000\u0000\u0000\u0000\u0000\u0000\u0000\u0000\u0000\u0000\u0000\u0000\u0000\u0000\u0000\u0000\u0000\u0000\u0000ÿÿ\u0000\u0000\u0000\u0000\u0000\u0000", "PMU.137\u0000\u0000\u0000\u0000\u0000\u0000\u0000\u0000\u0000\u0000‰\u0000\u000f\u0000\u0006\u0000\u0003\u0000\u0001PZR.AI          PZR.BV          PZR.CI          PZR.AV          PZR.BI          PZR.CV          ANA1            ANA2            ANA3            DIG.stat1_01    DIG.stat1_02    DIG.stat1_03    DIG.stat1_04    DIG.stat1_05    DIG.stat1_06    DIG.stat1_07    DIG.stat1_08    DIG.stat1_09    DIG.stat1_10    DIG.stat1_11    DIG.stat1_12    DIG.stat1_13    DIG.stat1_14    DIG.stat1_15    DIG.stat1_16    \u0001\u0000\u0000\u0000\u0000\u0000\u0000\u0000\u0001\u0000\u0000\u0000\u0000\u0000\u0000\u0000\u0001\u0000\u0000\u0000\u0000\u0000\u0000\u0000\u0000\u0000\u0000\u0000\u0000\u0000\u0000\u0000\u0000\u0000\u0000\u0000ÿÿ\u0000\u0000\u0000\u0000\u0000\u0000", "PMU.138\u0000\u0000\u0000\u0000\u0000\u0000\u0000\u0000\u0000\u0000Š\u0000\u000f\u0000\u0006\u0000\u0003\u0000\u0001PZR.AI          PZR.BV          PZR.CI          PZR.AV          PZR.BI          PZR.CV          ANA1            ANA2            ANA3            DIG.stat1_01    DIG.stat1_02    DIG.stat1_03    DIG.stat1_04    DIG.stat1_05    DIG.stat1_06    DIG.stat1_07    DIG.stat1_08    DIG.stat1_09    DIG.stat1_10    DIG.stat1_11    DIG.stat1_12    DIG.stat1_13    DIG.stat1_14    DIG.stat1_15    DIG.stat1_16    \u0001\u0000\u0000\u0000\u0000\u0000\u0000\u0000\u0001\u0000\u0000\u0000\u0000\u0000\u0000\u0000\u0001\u0000\u0000\u0000\u0000\u0000\u0000\u0000\u0000\u0000\u0000\u0000\u0000\u0000\u0000\u0000\u0000\u0000\u0000\u0000ÿÿ\u0000\u0000\u0000\u0000\u0000\u0000", "PMU.139\u0000\u0000\u0000\u0000\u0000\u0000\u0000\u0000\u0000\u0000‹\u0000\u000f\u0000\u0006\u0000\u0003\u0000\u0001PZR.AI          PZR.BV          PZR.CI          PZR.AV          PZR.BI          PZR.CV          ANA1            ANA2            ANA3            DIG.stat1_01    DIG.stat1_02    DIG.stat1_03    DIG.stat1_04    DIG.stat1_05    DIG.stat1_06    DIG.stat1_07    DIG.stat1_08    DIG.stat1_09    DIG.stat1_10    DIG.stat1_11    DIG.stat1_12    DIG.stat1_13    DIG.stat1_14    DIG.stat1_15    DIG.stat1_16    \u0001\u0000\u0000\u0000\u0000\u0000\u0000\u0000\u0001\u0000\u0000\u0000\u0000\u0000\u0000\u0000\u0001\u0000\u0000\u0000\u0000\u0000\u0000\u0000\u0000\u0000\u0000\u0000\u0000\u0000\u0000\u0000\u0000\u0000\u0000\u0000ÿÿ\u0000\u0000\u0000\u0000\u0000\u0000"]}, "DATA Type"=w380, "CFG Type"=w379) -> (w378:cluster{"DATA Type":string, "CFG Type":string[]})
    n179 = local read "Stop Button"() -> (w388:bool)
    n180 = Enqueue Element(queue=w384, element=w378, error in (no error)=w381) -> (queue out=w383:refnum<queue>, error out=w382:errorcluster)  [unwired: 1 in, 1 out]
  }
  n181 = while {
    shift-right: [w397] -> _
    shift-left: string[] [] -> [w410]
    shift-right: [w405] -> _
    shift-left: u16[] [] -> [w406]
    shift-right: [w404] -> _
    shift-left: u16 0 -> [w408]
    shift-right: [w400] -> _
    shift-left: u16[] [] -> [w402]
    shift-right: [w398] -> _
    shift-left: u16[] [] -> [w399]
    stop <- w413 stop-if-true
    n182 = event shown="[0] \"PMU Phasors List 2\": Double Click" {
      selector: _ -> [_]
      dyn-events: _ -> [_]
      timeout: _ -> [_]
      event "PMU Phasors List 2": Double Click {
        n183 = event-data() -> ("Row"=→"PMU Row Number":i32)  [unwired: 1 in]
        n184 = local read "PMU1 CFG Packet 2"() -> (w415:string[])
        n185 = Index Array(array=w415, index="PMU Phasors List 2") -> (element=w421:string)
        n186 = call "PMU_INFO.vi"("data in"=w421) -> ("RET_DATA"=w425:T10)
        n187 = Unbundle By Name(w425) -> ("NUMs.PHNMR"=w424:u8, "Station Name"=w418:string)
        n188 = String Length(string=w421) -> (length=w422:i32)
        n189 = String Subset(string=w421, offset (0)=26, length (rest)=w422) -> (substring=w420:string)
        n190 = for {
          N: w424 -> [_]
          tunnel: w420 -> [w434]
          shift-right: [w430] -> _
          shift-left: 0 ("offset (0)") -> [w432]
          tunnel: w418 -> [w428]
          tunnel: [w426] -> w414 mode=indexing
          n191 = String Subset(string=w434, offset (0)=w432, length (rest)=16 ("length (rest)")) -> (substring=w427:string)
          n192 = Add(x=w432, y=16) -> (x+y=w430:i32)
          n193 = Concatenate Strings(w428, "/", w427) -> (w426:string)
        }
        n194 = property on="PMU Phasors List" class="LstBox (strict)"("Item Names"=w414) -> ()  [unwired: 2 in, 2 out]
      }
    }
    n195 = event shown="[0] \"PMU Phasors List\": Double Click" {
      selector: _ -> [_]
      dyn-events: _ -> [_]
      timeout: _ -> [_]
      tunnel: [w454] -> w409
      tunnel: w408 -> [w453]
      tunnel: [w452] -> w404
      tunnel: [w451] -> w401
      event "PMU Phasors List": Double Click {
        n196 = event-data() -> ("Row"=w451:i32)  [unwired: 1 in]
        "Phasor Row Number" <- w451
        n197 = Increment(x=w453) -> (x+1=w452:u16)
        n198 = property on="PMU Phasors List" class="LstBox (strict)"() -> ("Item Names"=w455:string[])  [unwired: 2 in, 2 out]
        n199 = Index Array(array=w455, index=w451) -> (element=w454:string)
      }
    }
    n200 = Equal?(x="", y=w409) -> (x = y?=w411:bool)
    n201 = Equal?(x=w404, y=u16 0) -> (x = y?=w403:bool)
    n202 = case shown="False" w403 {
      tunnel: w402 -> [w440 w442]
      tunnel: [w438 w442] -> w400
      tunnel: w401 -> [w439 _]
      tunnel: w399 -> [w437 w441]
      tunnel: [w436 w441] -> w398
      frame False {
        n203 = local read "PMU Row Number"() -> (w435:i32)
        n204 = Build Array (concatenate)(w437, w435) -> (w436:i32[])
        "PMU number in List" <- w436
        n205 = Build Array (concatenate)(w440, w439) -> (w438:i32[])
        "Phasor number in selected PMU" <- w438
      }
      frame True {
      }
    }
    n206 = case shown="True" w411 {
      tunnel: w410 -> [w447 w450]
      tunnel: [w449 w450] -> w397
      tunnel: w409 -> [w448 _]
      frame False {
        n207 = Build Array (concatenate)(w447, w448) -> (w449:string[])
      }
      frame True {
      }
    }
    "Phasor_Names" <- w397
    n208 = case shown="False" w403 {
      tunnel: w406 -> [w445 w446]
      tunnel: w404 -> [w444 _]
      tunnel: [w443 w446] -> w405
      frame False {
        n209 = Build Array (concatenate)(w445, w444) -> (w443:u16[])
        "Phasors Index" <- w443
      }
      frame True {
      }
    }
    n210 = property on="Chosen Data 2" class="LstBox (strict)"("Item Names"=w397) -> ()  [unwired: 2 in, 2 out]
    n211 = local read "Stop Button"() -> (w413:bool)
  }
  n212 = while {
    tunnel: w19 -> [w531]
    tunnel: w18 -> [w530]
    tunnel: w4 -> [w529]
    tunnel: w3 -> [w528]
    tunnel: [w527] -> _
    tunnel: [w526] -> _
    tunnel: [w525] -> _
    tunnel: [w524] -> _
    stop <- w552 stop-if-true
    w489 = u16 8
    w492 = u16 4
    w497 = u16 1
    w506 = u16 2
    w547 = u32 0
    w543 = 4 ("length (rest)")
    n213 = Dequeue Element(queue=w531, error in (no error)=w530) -> (queue out=w527:refnum<queue>, element=w551:cluster{"DATA Type":string, "CFG Type":string[]}, error out=w526:errorcluster)  [unwired: 1 in, 1 out]
    n214 = Unbundle By Name(w551) -> ("DATA Type"=w539:string, "CFG Type"=w550:string[])
    "DATA FRAME 2" <- w539
    n215 = property on="Names of PMUs" class="LstBox (strict)"() -> ("Value"=w522:i32)  [unwired: 2 in, 2 out]
    n216 = property on="TIME_BASE" class="DigNum (strict)"() -> ("Value"=w521:u32)  [unwired: 2 in, 2 out]
    n217 = String Subset(string=w539, offset (0)=6, length (rest)=w543) -> (substring=w545:string)
    n218 = String Subset(string=w539, offset (0)=10, length (rest)=w543) -> (substring=w541:string)
    n219 = Index Array(array=w550, index=w522) -> (element=w544:string)
    n220 = property on="NUM_of_PMUs" class="DigNum (strict)"() -> ("Value"=w523:u32)  [unwired: 2 in, 2 out]
    n221 = Type Cast(type=w547, x=w545) -> (*(type *) &x=w546:u32)
    n222 = Type Cast(type=w547, x=w541) -> (*(type *) &x=w540:u32)
    n223 = call "PMU_INFO.vi"("data in"=w544) -> ("RET_DATA"=w537:T10)
    n224 = call "PMU_DATA_PACK.vi"("DATA FRAME"=w539, "DATA_IN"=w537, "PMUs_NUM"=w523) -> ("PMU DATA Packet"=→"PMU DATA Packet 2":string[], "DATA_DTLD"=w519:T11)  [unwired: 6 in]
    n225 = call "UNIX-DATE_TIME.vi"("TIME_BASE"=w521, "FRACSEC"=w540, "SOC"=w546) -> ("Date/Time"=w535:string, "seconds"=→"seconds":dbl)
    n226 = Not Equal?(x=w535, y="1-1-1970, 2:0:0 0.000000") -> (x != y?=w538:bool)
    n227 = Unbundle By Name(w537) -> ("UNITs"=→"UNITs 2":T2)
    n228 = case shown="True" w538 {
      tunnel: [_ w688] -> w532
      tunnel: w535 -> [_ w688]
      frame False {
      }
      frame True {
      }
    }
    "Date/Time 3" <- w532
    n229 = Bundle By Name(cluster=T7 {"Date/Time"="26-12-2013, 0:30:36 0.866666", "DATA_DTLD"={"PZRs Packet"=[], "FREQ Packet"=[], "DFREQ Packet"=[], "ANG Packet"=[], "DGTL Packet"=[]}}, "DATA_DTLD"=w519, "Date/Time"=w532) -> (w520:T7)
    n230 = Unbundle By Name(w519) -> ("PZRs Packet"=w512:string[], "FREQ Packet"=w518:string[], "DFREQ Packet"=w517:string[], "ANG Packet"=w493:string[], "DGTL Packet"=w482:string[])
    "PZRs Packet" <- w512
    "FREQ Packet" <- w518
    "DFREQ Packet" <- w517
    "ANG Packet" <- w493
    "DGTL Packet" <- w482
    n231 = Enqueue Element(queue=w529, element=w520, error in (no error)=w528) -> (queue out=w525:refnum<queue>, error out=w524:errorcluster)  [unwired: 1 in, 1 out]
    n232 = local read "Stop Button"() -> (w552:bool)
    n233 = local read "Phasors Floatingpoint?"() -> (w504:bool[])
    n234 = local read "Polar?"() -> (w494:bool[])
    n235 = for {
      tunnel: w493 -> [w580] mode=indexing
      tunnel: [w578] -> w485 mode=indexing
      tunnel: [w577] -> w462 mode=indexing
      i -> [w582]
      n236 = local read "Analog"() -> (w581:u16[])
      n237 = Index Array(array=w581, index=w582) -> (element=w576:u16)
      n238 = for {
        N: w576 -> [w586]
        tunnel: w580 -> [w591]
        shift-right: [w587] -> _
        shift-left: 0 ("offset (0)") -> [w589]
        tunnel: [w585] -> w578 mode=indexing
        tunnel: [w583] -> w577 mode=indexing
        n239 = String Length(string=w591) -> (length=w590:i32)
        n240 = Divide(x=w590, y=w586) -> (x/y=w588:dbl)
        n241 = Add(x=w589, y=w588) -> (x+y=w587:dbl)
        n242 = String Subset(string=w591, offset (0)=w589, length (rest)=w588) -> (substring=w585:string)
        n243 = Type Cast(type=sgl 0.0 ("32-bit IEEE 754"), x=w585) -> (*(type *) &x=w583:sgl)
      }
    }
    "Analogs" <- w485
    n244 = for {
      tunnel: w482 -> [w562] mode=indexing
      tunnel: [w558] -> w484 mode=indexing
      tunnel: [w557] -> w483 mode=indexing
      tunnel: w482 -> [w554] mode=indexing
      tunnel: [w553] -> w481 mode=indexing
      i -> [w563]
      n245 = local read "Digitals"() -> (w560:u16[])
      n246 = Index Array(array=w560, index=w563) -> (element=w559:u16)
      n247 = for {
        N: w559 -> [w570]
        tunnel: w562 -> [w575]
        shift-right: [w571] -> _
        shift-left: 0 ("offset (0)") -> [w573]
        tunnel: [w566] -> w558 mode=indexing
        tunnel: [w569] -> w557 mode=indexing
        tunnel: [w564] -> _ mode=indexing
        n248 = String Length(string=w575) -> (length=w574:i32)
        n249 = Divide(x=w574, y=w570) -> (x/y=w572:dbl)
        n250 = Add(x=w573, y=w572) -> (x+y=w571:dbl)
        n251 = String Subset(string=w575, offset (0)=w573, length (rest)=w572) -> (substring=w566:string)
        n252 = Type Cast(type=u16 0 ("offset (0)"), x=w566) -> (*(type *) &x=w565:u16)
        n253 = Type Cast(type=u16 1 ("y"), x=w566) -> (*(type *) &x=w569:u16)
        n254 = Number To Boolean Array(number=w565) -> (Boolean array=w564:bool[])
      }
      n255 = Type Cast(type=u16 0 ("offset (0)"), x=w554) -> (*(type *) &x=w556:u16)
      n256 = Number To Boolean Array(number=w556) -> (Boolean array=w553:bool[])
    }
    "Array" <- w484
    "Array 2" <- w483
    "Boolean array" <- w481
    n257 = for {
      tunnel: w518 -> [w687] mode=indexing
      tunnel: [w686] -> w478 mode=indexing
      n258 = call "HEX_DEC.vi"("HEX IN"=w687) -> ("DEC OUT"=w686:sgl)
    }
    n259 = for {
      tunnel: w517 -> [w685] mode=indexing
      tunnel: [w684] -> w477 mode=indexing
      n260 = call "HEX_DEC.vi"("HEX IN"=w685) -> ("DEC OUT"=w684:sgl)
    }
    n261 = for {
      tunnel: w512 -> [w602] mode=indexing
      tunnel: [w605] -> w511 mode=indexing
      tunnel: [w603] -> w509 mode=indexing
      tunnel: w504 -> [w601] mode=indexing
      tunnel: [w599] -> w502 mode=indexing
      tunnel: [w595] -> w501 mode=indexing
      tunnel: [w594] -> w500 mode=indexing
      tunnel: w494 -> [w596] mode=indexing
      tunnel: [w597] -> w479 mode=indexing
      tunnel: [w593] -> w476 mode=indexing
      tunnel: [w592] -> w480 mode=indexing
      i -> [w607]
      n262 = local read "Phasor"() -> (w608:u16[])
      n263 = Index Array(array=w608, index=w607) -> (element=w598:u16)
      n264 = for {
        N: w598 -> [w653]
        tunnel: w602 -> [w659]
        shift-right: [w655] -> _
        shift-left: 0 ("offset (0)") -> [w657]
        tunnel: [w654] -> w605 mode=indexing
        n265 = String Length(string=w659) -> (length=w658:i32)
        n266 = Divide(x=w658, y=w653) -> (x/y=w656:dbl)
        n267 = Add(x=w657, y=w656) -> (x+y=w655:dbl)
        n268 = String Subset(string=w659, offset (0)=w657, length (rest)=w656) -> (substring=w654:string)
      }
      n269 = for {
        N: w598 -> [w645]
        tunnel: w602 -> [w650]
        shift-right: [w643] -> _
        shift-left: 0 ("offset (0)") -> [w648]
        tunnel: [w640] -> w603 mode=indexing
        tunnel: w601 -> [w642]
        tunnel: [w638] -> w595 mode=indexing
        n270 = String Length(string=w650) -> (length=w649:i32)
        n271 = Multiply(x=w645, y=2) -> (x*y=w646:i32)
        n272 = Divide(x=w649, y=w646) -> (x/y=w647:dbl)
        n273 = String Subset(string=w650, offset (0)=w648, length (rest)=w647) -> (substring=w640:string)
        n274 = case shown="False" w642 {
          tunnel: [4 ("y") 8 ("y")] -> w641
          frame False {
          }
          frame True {
          }
        }
        n275 = Add(x=w648, y=w641) -> (x+y=w643:i32)
        n276 = Type Cast(type=sgl 0.0 ("32-bit IEEE 754"), x=w640) -> (*(type *) &x=w638:sgl)
      }
      n277 = for {
        N: w598 -> [w630]
        tunnel: w602 -> [w635]
        shift-right: [w628] -> _
        shift-left: 4 -> [w633]
        tunnel: [w624] -> w599 mode=indexing
        tunnel: w601 -> [w627]
        tunnel: [w623] -> w594 mode=indexing
        n278 = String Length(string=w635) -> (length=w634:i32)
        n279 = Multiply(x=w630, y=2) -> (x*y=w631:i32)
        n280 = Divide(x=w634, y=w631) -> (x/y=w632:dbl)
        n281 = String Subset(string=w635, offset (0)=w633, length (rest)=w632) -> (substring=w624:string)
        n282 = case shown="False" w627 {
          tunnel: [4 ("y") 8 ("y")] -> w626
          frame False {
          }
          frame True {
          }
        }
        n283 = Add(x=w633, y=w626) -> (x+y=w628:i32)
        n284 = Type Cast(type=sgl 0.0 ("32-bit IEEE 754"), x=w624) -> (*(type *) &x=w623:sgl)
      }
      n285 = case shown="False" w596 {
        tunnel: w595 -> [w617 w622]
        tunnel: w594 -> [w616 w621]
        tunnel: [w615 w620] -> w597
        frame False {
          n286 = Re/Im To Polar(2:w616, 3:w617) -> (0:w618:sgl[], 1:w619:sgl[])
          n287 = Polar To Complex(1:w618, 2:w619) -> (0:w615:csg[])
        }
        frame True {
          n288 = Polar To Complex(1:w621, 2:w622) -> (0:w620:csg[])
        }
      }
      n289 = case shown="True" w596 {
        tunnel: w595 -> [w612 w614]
        tunnel: w594 -> [w611 w613]
        tunnel: [w610 w614] -> w593
        tunnel: [w609 w613] -> w592
        frame False {
          n290 = Re/Im To Polar(2:w611, 3:w612) -> (0:w609:sgl[], 1:w610:sgl[])
        }
        frame True {
        }
      }
    }
    n291 = property on="Frequency" class="Arr (strict)"("Value"=w478) -> ()  [unwired: 2 in, 2 out]
    n292 = local read "PMU1 CFG Packet"() -> (w513:string[])
    n293 = property on="dFreq" class="Arr (strict)"("Value"=w477) -> ()  [unwired: 2 in, 2 out]
    n294 = for {
      tunnel: w513 -> [w665] mode=indexing
      tunnel: [w679] -> w516 mode=indexing
      tunnel: [w671] -> w515 mode=indexing
      tunnel: [w670] -> w514 mode=indexing
      tunnel: [w660] -> w487 mode=indexing
      n295 = String Subset(string=w665, offset (0)=20, length (rest)=2 ("length (rest)")) -> (substring=w681:string)
      n296 = String Subset(string=w665, offset (0)=22, length (rest)=2 ("length (rest)")) -> (substring=w677:string)
      n297 = String Subset(string=w665, offset (0)=18, length (rest)=2 ("length (rest)")) -> (substring=w668:string)
      n298 = String Subset(string=w665, offset (0)=24, length (rest)=2 ("length (rest)")) -> (substring=w672:string)
      n299 = Type Cast(type=u16 0, x=w681) -> (*(type *) &x=w679:u16)
      n300 = Type Cast(type=u16 0, x=w677) -> (*(type *) &x=w671:u16)
      n301 = Type Cast(type=u16 0 ("element"), x=w668) -> (*(type *) &x=w664:u16)
      n302 = Type Cast(type=u16 0, x=w672) -> (*(type *) &x=w670:u16)
      n303 = Split Number(x=w664) -> (lo(x)=w663:u8)  [unwired: 1 out]
      n304 = And(x=w663, y=u16 15 ("element")) -> (x .and. y?=w660:u16)
    }
    "Phasor" <- w516
    "Analog" <- w515
    "Digitals" <- w514
    "Format" <- w487
    n305 = local read "Names of PMUs"() -> (w461:i32)
    n306 = Transpose 2D Array(2D array=w501) -> (transposed array=→"transposed array 4":sgl[][])
    n307 = And(x=w487, y=w506) -> (x .and. y?=w507:u16[])
    n308 = property on="Complex Phasors" class="Arr (strict)"("Value"=w479) -> ()  [unwired: 2 in, 2 out]
    n309 = Transpose 2D Array(2D array=w509) -> (transposed array=→"Real":string[][])
    n310 = Transpose 2D Array(2D array=w502) -> (transposed array=→"Imaginary":string[][])
    n311 = Transpose 2D Array(2D array=w500) -> (transposed array=→"transposed array 5":sgl[][])
    n312 = And(x=w487, y=w489) -> (x .and. y?=w488:u16[])
    n313 = And(x=w487, y=w492) -> (x .and. y?=w491:u16[])
    n314 = And(x=w487, y=w497) -> (x .and. y?=w496:u16[])
    n315 = Transpose 2D Array(2D array=w511) -> (transposed array=→"Transposed":string[][])
    n316 = property on="Magnitude" class="Arr (strict)"("Value"=w476) -> ()  [unwired: 2 in, 2 out]
    n317 = property on="Angle" class="Arr (strict)"("Value"=w480) -> ()  [unwired: 2 in, 2 out]
    n318 = property on="Analog Values" class="Arr (strict)"("Value"=w462) -> ()  [unwired: 2 in, 2 out]
    n319 = Index Array(array=w476, index (row)=w461) -> (element=w472:sgl[])  [unwired: 1 in]
    n320 = Equal?(x=w507, y=w506) -> (x = y?=→"Phasors Floatingpoint?":bool[])
    n321 = Equal?(x=w488, y=w489) -> (x = y?=→"Freq Floating?":bool[])
    n322 = Equal?(x=w491, y=w492) -> (x = y?=→"Analog Floating?":bool[])
    n323 = Equal?(x=w496, y=w497) -> (x = y?=→"Polar?":bool[])
    n324 = Index Array(array=w462, index (row)=w461) -> (element=w459:sgl[])  [unwired: 1 in]
    n325 = local read "Frequency"() -> (w456:sgl[])
    n326 = local read "dFreq"() -> (w464:sgl[])
    n327 = local read "seconds"() -> (w474:dbl)
    n328 = Index Array(array=w456, index=w461) -> (element=w468:sgl)
    n329 = Index Array(array=w464, index=w461) -> (element=w465:sgl)
    n330 = local read "DATA_RATE"() -> (w470:u32)
    n331 = Build Array(w468) -> (w467:sgl[])
    n332 = Build Array(w465) -> (w466:sgl[])
    n333 = Seconds To Date/Time(time stamp (now)=w474) -> (date time rec=w473:T12)  [unwired: 1 in]
    n334 = Reciprocal(x=w470) -> (1/x=w458:dbl)
    n335 = Date/Time To Seconds(2:w473) -> (0:w460:timestamp)  [unwired: 1 in]
    n336 = Bundle By Name("t0"=w460, "Y"=w472, "dt"=w458) -> (→"MagnitudePMU":waveform(sgl))  [unwired: 1 in]
    n337 = Bundle By Name("t0"=w460, "Y"=w467, "dt"=w458) -> (→"FrequencyPMU":waveform(sgl))  [unwired: 1 in]
    n338 = Bundle By Name("t0"=w460, "Y"=w466, "dt"=w458) -> (→"PMUROCOF":waveform(sgl))  [unwired: 1 in]
    n339 = Bundle By Name("t0"=w460, "Y"=w459, "dt"=w458) -> (→"PMUAnalogs":waveform(sgl))  [unwired: 1 in]
  }
  n340 = while {
    tunnel: w4 -> [w716]
    tunnel: w3 -> [w715]
    tunnel: w2 -> [w693]
    tunnel: w1 -> [w692]
    tunnel: [w690] -> _
    tunnel: [w689] -> _
    stop <- w717 stop-if-true
    # "Character Set"
    n341 = Dequeue Element(queue=w716, error in (no error)=w715) -> (element=w702:T7)  [unwired: 1 in, 3 out]
    n342 = property on="Phasor number in selected PMU" class="Arr (strict)"() -> ("Value"=w712:i32[])  [unwired: 2 in, 2 out]
    n343 = property on="PMU number in List" class="Arr (strict)"() -> ("Value"=w713:i32[])  [unwired: 2 in, 2 out]
    n344 = property on="Complex Phasors" class="Arr (strict)"() -> ("Value"=w711:csg[][])  [unwired: 2 in, 2 out]
    n345 = property on="Analog Values" class="Arr (strict)"() -> ("Value"=w710:sgl[][])  [unwired: 2 in, 2 out]
    n346 = property on="Frequency" class="Arr (strict)"() -> ("Value"=w709:sgl[])  [unwired: 2 in, 2 out]
    n347 = property on="dFreq" class="Arr (strict)"() -> ("Value"=w708:sgl[])  [unwired: 2 in, 2 out]
    n348 = Unbundle By Name(w702) -> ("Date/Time"=→"Date/Time 4":string)
    n349 = property on="Phasors Index" class="Arr (strict)"() -> ("Value"=w714:u16[])  [unwired: 2 in, 2 out]
    n350 = local read "Boolean array"() -> (w707:bool[][])
    n351 = call "DataChosen.vi"("Phasor Index"=w714, "Boolean array"=w707, "PMU Number in List"=w713, "Phasor  Number in List"=w712, "Complex Phasors"=w711, "Analog Values"=w710, "Frequency"=w709, "dFreq"=w708) -> ("Complex Phasors Output"=w705:csg[], "FREQ Values"=w704:dbl[], "DFREQ Values"=w703:dbl[])  [unwired: 5 in]
    "FREQ Values" <- w704
    "DFREQ Values" <- w703
    "Complex Phasors" <- w705
    n352 = Complex To Polar(r * e^(i*theta)=w705) -> (r=w700:sgl[], theta=w699:sgl[])
    "Angle" <- w699
    "Magnitude" <- w700
    n353 = property on="Phasor_Names" class="Arr (strict)"() -> ("Value"=w706:string[])  [unwired: 2 in, 2 out]
    n354 = for {
      tunnel: w706 -> [w732] mode=indexing
      tunnel: w705 -> [_] mode=indexing
      tunnel: w704 -> [w726] mode=indexing
      tunnel: w703 -> [w723] mode=indexing
      tunnel: w700 -> [w730] mode=indexing
      tunnel: w699 -> [w728] mode=indexing
      shift-right: [w718] -> _
      shift-left: "" ("string") -> [w719]
      tunnel: [w718] -> w696 mode=indexing
      w724 = ";" ("string")
      n355 = local read "Date/Time 4"() -> (w731:string)
      n356 = Number To Fractional String(number=w726) -> (F-format string=w725:string)  [unwired: 3 in]
      n357 = Number To Fractional String(number=w730) -> (F-format string=w729:string)  [unwired: 3 in]
      n358 = Number To Fractional String(number=w723) -> (F-format string=w722:string)  [unwired: 3 in]
      n359 = Number To Fractional String(number=w728) -> (F-format string=w727:string)  [unwired: 3 in]
      n360 = Concatenate Strings(w732, w724, w731, w724, w729, w724, w727, w724, w725, w724, w722) -> (w720:string)
      n361 = Concatenate Strings(w719, w720, "#" ("string")) -> (w718:string)
    }
    n362 = local read "Stop Button"() -> (w717:bool)
    n363 = property on="Phasors Index" class="Arr (strict)"() -> ("Value"=w695:u16[])  [unwired: 2 in, 2 out]
    n364 = Array Max & Min(array=w695) -> (max value=w694:u16)  [unwired: 3 out]
    n365 = Decrement(x=w694) -> (x-1=w697:u16)
    n366 = Index Array(array=w696, index=w697) -> (element=w691:string)
    "UDP STRNG 2" <- w691
    n367 = Enqueue Element(queue=w693, element=w691, error in (no error)=w692) -> (queue out=w690:refnum<queue>, error out=w689:errorcluster)  [unwired: 1 in, 1 out]
  }
  n368 = Flush Queue(queue=w36, error in (no error)=w35) -> ()  [unwired: 3 out]
